vi "TLB Native Dynamic Events ver 0.17h.vi"() -> ()   [LabVIEW 2018]
uses:
  Labview Training Phase 2/Enum Controls/States for Action Engine.ctl
  TLB Type Definitions/State Type Definitions, for 0.26g versions and later 2.ctl
  TLB Type Definitions/Intruction Type Definitions.ctl
  TLB Type Definitions/Encoder cluster.ctl
  TLB Type Definitions/PING CLUSTER.ctl
  <vilib>/Studica/Studica Toolkit/NavX/NavX.lvlib
  <vilib>/Studica/Studica Toolkit/Background/DIO Channel.ctl
  Underlying VI's/NavX VI/navX type def.ctl
  <vilib>/Studica/Studica Toolkit/Background/I2C Channel.ctl
  TLB Type Definitions/Vision cluster.ctl
  <vilib>/NI_Real-Time Target Support.lvlib
  TLB Type Definitions/Stepper cluster.ctl
  Experimental VI's/Archived VI's/MOTOR CONTROL NO PID Type Def.ctl
  Underlying VI's/I2C Master VI/I2C MASTER Type Def.ctl
  Underlying VI's/I2C Master VI/I2C_MASTER_WRITE_NEW Type Def.ctl
  <vilib>/userdefined/High Color/IMAQdx.ctl
  Underlying VI's/I2C Master VI/Arduino_Interfacing.ctl
  TLB Type Definitions/Yaw Cluster.ctl
  TLB Type Definitions/Time cluster.ctl
  TLB Type Definitions/Y Stepper cluster.ctl
  Underlying VI's/Modified webcam FGV/Webcam AE.ctl
  Underlying VI's/Elasped Timer/Elapsed timer control.ctl
  Underlying VI's/Motor Control VI with PID/MOTOR CONTROL WITH PID AE DATA MODE TYPE DEF.ctl
  Underlying VI's/Motor Control VI with PID/MOTOR CONTROL WITH PID AE DIRECTION TYPE DEF.ctl
  TLB Type Definitions/IR Sensor Type Def.ctl
  <vilib>/myRIO/Common/Instrument Driver Framework/myRIO v1.0/AI/typedefs/AI Channels Enum.ctl
  <vilib>/myRIO/Common/Instrument Driver Framework/myRIO v1.0/AI/typedefs/AI Channels List.ctl
  TLB Type Definitions/Motor Speed Cluster.ctl
  <vilib>/Utility/RT CPU Load.ctl
panel:
  out "x-y":dbl
  out "Left IR Sensor":dbl
  out "Obstacle detected":bool
  out "Speed & distance":T1
  out "Object Center Coordinates":cluster{"x":sgl, "y":sgl}
  out "Object detection cluster":T2
  out "Time up flag":bool
  out "Task selection":u8
  in  "Object recognition mode":enum16{"Ball", "Soap", "Gel", "Pipe", "None"}(ring)
  out "NavX Readings":T3
  out "Arduino Data":T4
  out "CPU loads":T5[](array[typedef]) {"ISR (%)" format="%#.2f"; "Idle (%)" format="%#.2f"; "Background (%)" format="%#.2f"; "Normal (%)" format="%#.2f"; "Above Normal (%)" format="%#.2f"; "High (%)" format="%#.2g"; "Timed Structures (%)" format="%#.2g"; "Time Critical (%)" format="%#.2g"; "Total (%)" format="%#.2g"}
  out "TASK ENABLE":bool
  out "Rising Edge":bool
  in  "Green LED":bool
  out "I2C Error":errorcluster
  out "State Logic":T6=enum."Startup"
  out "elements":T7[](array[typedef])
  in  "STOP TASK":bool
  in  "OK Button":bool
  in  "STOP":bool
  out "error out":errorcluster
  out "Action Queue Items":i32
  out "State Logic Queue Items":i32
  out "Action Queues items":string[](array[string])=["Hardware reset", "Software reset", ""]
  out "Action State":string
  # "System Health Status Update"
  # "VISION"
  # "TLB FRAMEWORK STATUS"
  # "Test Programme written by Calvin Loke    Dated: 28 Aug 2019\nTest Programme revised by Dr Alex See   Dated 30 Aug 2019\n\nRevision date: 20/03/2020\nProgramme version:   TLB Native Dynamic Events ver 0.14a"
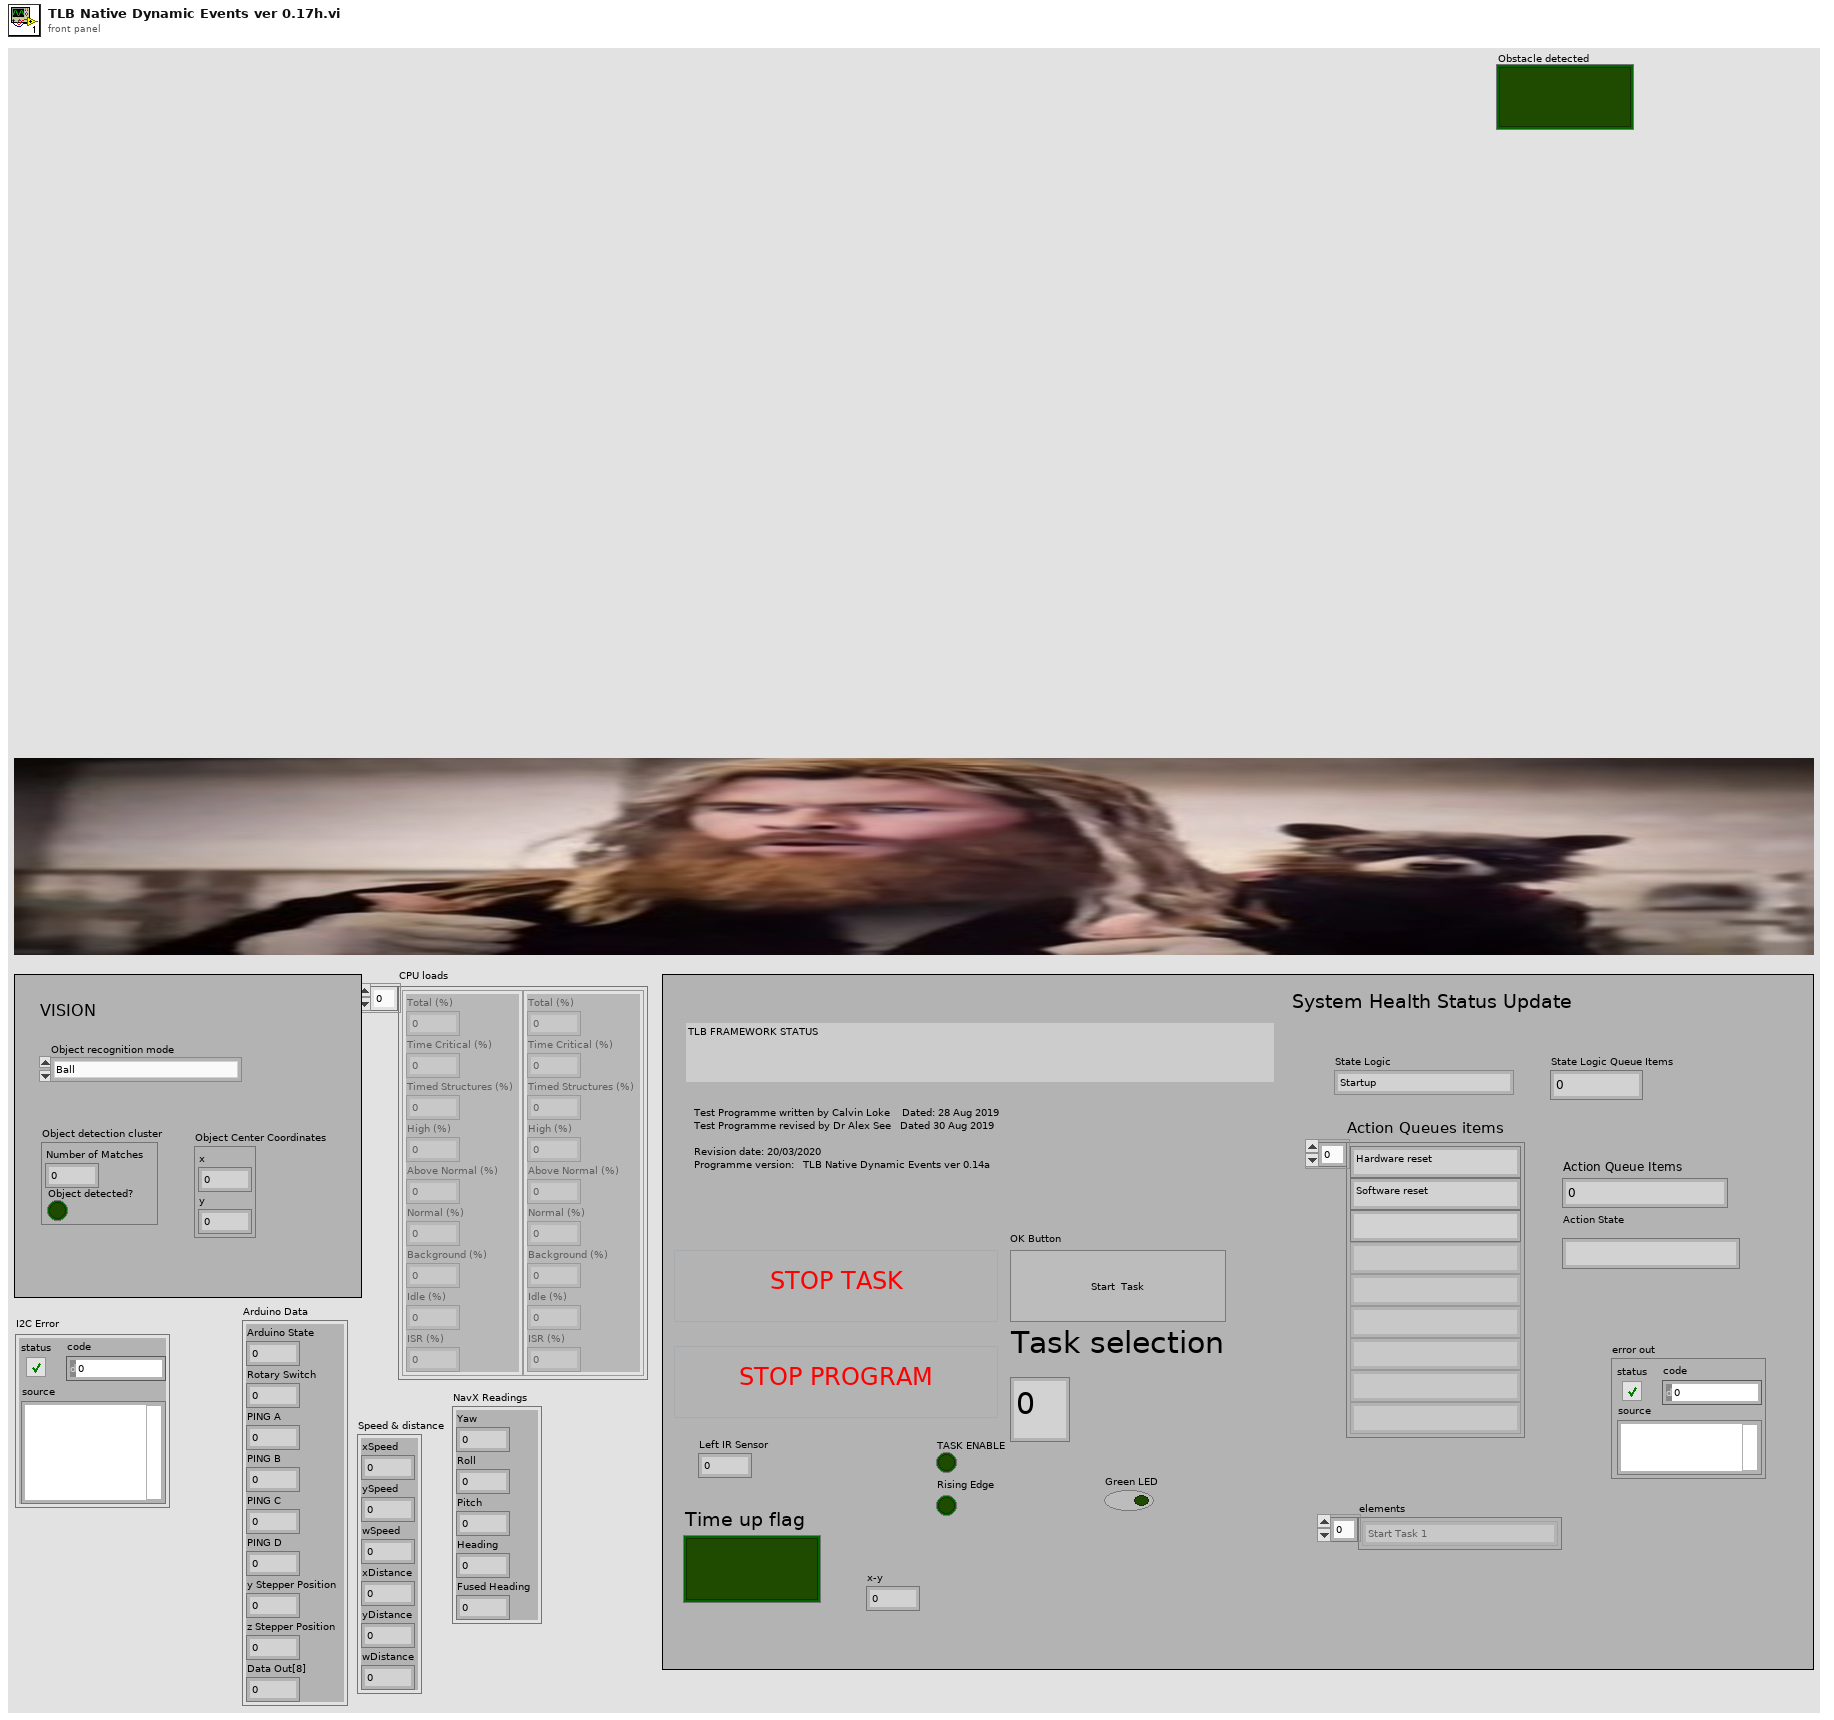
[diagram p1: front panel]
types:
  T1 = cluster{"xSpeed":dbl, "ySpeed":dbl, "wSpeed":dbl, "xDistance":dbl, "yDistance":dbl, "wDistance":dbl}
  T2 = cluster{"Number of Matches":i32, "Object detected?":bool}
  T3 = cluster{"Yaw":dbl, "Roll":dbl, "Pitch":dbl, "Heading":dbl, "Fused Heading":dbl}
  T4 = cluster{"Arduino State":u8, "Rotary Switch":u8, "PING A":u8, "PING B":u8, "PING C":u8, "PING D":u8, "y Stepper Position":u8, "z Stepper Position":u8, "Data Out[8]":u8}
  T5 = typedef "NI_Real-Time Target Support.lvlib/RT CPU Load.ctl" = cluster{"Total (%)":dbl, "Time Critical (%)":dbl, "Timed Structures (%)":dbl, "High (%)":dbl, "Above Normal (%)":dbl, "Normal (%)":dbl, "Background (%)":dbl, "Idle (%)":dbl, "ISR (%)":dbl}
  T6 = typedef "State Type Definitions, for 0.26g versions and later 2.ctl" = enum16{"None", "Startup", "Move to Angle", "True Stop", "Idle", "Shutdown", "Task 1A", "Task 1B", "Task 2:Raise Arm", "Task 2:Sensor Mode", "Task 2:Reverse Mode", "Task 3", "Task 4_A", "Task 4_B", "Task 4_C", "Task 4_D", "Task 5A", "Task 5B", "Task 5C", "Task 5D", "Task 5E: POSITION ARM", "Task 5F: ARM GRAB HEIGHT", "Task 5G: CLOSE CLAW", "Task 5H: RAISE ARM", "Task 6_A", "Task 6_B", "Task 7", "Task 8A: RAISE ARM", "Task 8B: MOVE TO BOX", "Task 8C: CAM BURST", "Task 8D: PROCESS IMAGE", "Task 8E: ROBOT ADJUST", "Task 8F: CAM BURST 2", "Task 8G: PROCESS IMAGE 2", "Task 8H: ARM ADJUST", "Task 8I: ARM GRAB HEIGHT", "Task 8J: CLOSE CLAW", "Task 8K: RAISE MY SWORD", "Task 9A: Raise Arm", "Task 9B: Rotate to Angle", "Task 9C: Detect Box", "Task 9D: MOVE FORWARD", "Task 9E: MOVE LEFT", "Task 9F: SCAN BOX", "Task 9G: MOVE RIGHT", "Task 9H: SCAN BOX 2", "Task 9I: ROTATE 90 CW", "Task 9J: FORWARD", "Task 9K: RAM WALL", "Task 9L: MOVE RIGHT", "Task 9M: SCAN BOX 3", "Task 9M: MOVE RIGHT", "Task 9N: SCAN BOX 4", "PENIS", "PENIS 2", "PENIS 3", "Task 9R: PROCESS COLOUR", "Task A1: Task 9 Open cam", "Task A2: Task 9 Move Arm", "Task A3: Task 9 Set Timer", "Task A4: Tasl 9 Capture images", "Task A5: Task 9 Close camera", "Task A6: Process Colour", "Task A7: Dispose Camera Buffer"}
  T7 = typedef "Intruction Type Definitions.ctl" = enum16{"None", "Start Task 1", "Start Task 2", "Start Task 3", "Start Task 4", "Start Task 5", "Start Task 6", "Start Task 7", "Start Task 8 - BALL", "Start Task 8 - Gel", "Start Task 8 - Pipe", "Start Task 8 - Soap", "Start Task 9", "Start Task A", "Start Task B", "Exit"}
  T8 = typedef "Motor Speed Cluster.ctl" = cluster{"ySpeed":dbl, "xSpeed":dbl, "wSpeed":dbl}
  T9 = typedef "IR Sensor Type Def.ctl" = cluster{"Left IR Sensor":dbl, "Arm IR Sensor":dbl, "Bottom IR Sensor":dbl}
  T10 = typedef "Y Stepper cluster.ctl" = cluster{"yStepper desired":u8}
  T11 = typedef "Time cluster.ctl" = cluster{"Time up flag":bool, "SET TIME TO CHECK":dbl}
  T12 = typedef "Yaw Cluster.ctl" = cluster{"Yaw":dbl, "Compass":dbl}
  T13 = typedef "Stepper cluster.ctl" = cluster{"y Stepper Position":u8, "z Stepper Position":u8}
  T14 = typedef "DIO Channel.ctl" = enum16{"Not Connected", "A/DIO1", "A/DIO2", "A/DIO3", "A/DIO4", "A/DIO5", "A/DIO6", "A/DIO7", "A/DIO13", "B/DIO1", "B/DIO2", "B/DIO3", "B/DIO4", "B/DIO5", "B/DIO6", "B/DIO7", "B/DIO13", "C/DIO0", "C/DIO1", "C/DIO2", "C/DIO3", "C/DIO4", "C/DIO5", "C/DIO6", "C/DIO7"}
  T15 = typedef "Vision cluster.ctl" = cluster{"Recognized Object":bool, "Object X coordinate":dbl, "Object Y coordinate":dbl}
  T16 = typedef "PING CLUSTER.ctl" = cluster{"PING_A":u8, "PING_B":u8, "PING_C":u8, "PING_D":u8}
  T17 = typedef "Encoder cluster.ctl" = cluster{"xDistance":dbl, "yDistance":dbl, "wDistance":dbl}
  T18 = cluster{"DIO Channel":T14, "FPGA VI Reference Out":refnum<k20>}
  T19 = typedef "navX type def.ctl" = enum16{"Get i2C reference", "Read Values", "Zero Yaw"}
  T20 = typedef "Arduino_Interfacing.ctl" = enum16{"Initialize", "Write to Arduino", "Read From Arduino"}
  T21 = typedef "I2C Channel.ctl" = enum16{"Not Connected", "A", "B"}
  T22 = typedef "States for Action Engine.ctl" = enum16{"Initialize", "Write", "Read"}
  T23 = cluster{"I2C Ref Out":cluster{"I2C Channel":T21, "FPGA VI Reference Out":refnum<k20>}, "Connected":bool, "Slave Address (7-bit)":u8, "Registry":u8[]}
  T24 = typedef "Intruction Type Definitions.ctl" = enum16{"None", "Start Task 1", "Start Task 2", "Start Task 3", "Start Task 4", "Start Task 5", "Start Task 6", "Start Task 7", "Start Task 8", "Start Task 9", "Start Task A", "Start Task B", "Exit"}
  T25 = typedef "IMAQ Image.ctl" = refnum<image>
  T26 = typedef "State Type Definitions.ctl" = enum16{"None", "Startup", "Move to Angle", "True Stop", "Idle", "Shutdown", "Task 1", "Task 2:Raise Arm", "Task 2:Sensor Mode", "Task 2:Reverse Mode", "Task 3", "Task 4_A", "Task 4_B", "Task 4_C", "Task 4_D", "Task 5A: ARM CAM HEIGHT", "Task 5B: MOVE TO BOX", "Task 5C: CAM BURST", "Task 5D: PROCESS IMAGE", "Task 5E: POSITION ARM", "Task 5F: ARM GRAB HEIGHT", "Task 5G: CLOSE CLAW", "Task 5H: RAISE ARM", "Task 6_A", "Task 6_B", "Task 7", "Task 8A: RAISE ARM", "Task 8B: MOVE TO BOX", "Task 8C: CAM BURST", "Task 8D: PROCESS IMAGE", "Task 8E: ROBOT ADJUST", "Task 8F: CAM BURST 2", "Task 8G: PROCESS IMAGE 2", "Task 8H: ARM ADJUST", "Task 8I: ARM GRAB HEIGHT", "Task 8J: CLOSE CLAW", "Task 8K: RAISE MY SWORD", "Task 9A: Raise Arm", "Task 9B: Rotate to Angle", "Task 9C: Rotation alignmnet", "Task B"}
  T27 = typedef "MOTOR CONTROL WITH PID AE DIRECTION TYPE DEF.ctl" = enum16{"y-axis movement", "x-axis movement", "rotation", "stop", "reset encoders"}
  T28 = typedef "MOTOR CONTROL WITH PID AE DATA MODE TYPE DEF.ctl" = enum16{"Init AE", "Write to AE", "Read from AE"}
  T29 = typedef "Elapsed timer control.ctl" = enum16{"Start", "Pause", "Initialize"}
  T30 = typedef "I2C_MASTER_WRITE_NEW Type Def.ctl" = enum16{"Ultrasonic sensors", "Stepper origin", "zStepper 13.3k", "zStepper 13k", "zStepper 12k", "zStepper 11k", "zStepper 10k", "zStepper 9k", "zStepper 8k", "zStepper 7k", "zStepper 6k", "zStepper 5k", "zStepper 4k", "zStepper 3k", "zStepper 2k", "zStepper 1k", "zStepper 900", "zStepper 800", "zStepper 700", "zStepper 600", "zStepper 500", "zStepper 400", "zStepper 300", "zStepper 200", "zStepper 100", "zStepper 0", "yStepper control", "Open Claw", "Close Claw", "Soft Reset"}
  T31 = typedef "Webcam AE.ctl" = enum16{"Initialize Camera", "Open Camera", "Continuous Acquisition", "Close Camera", "Retrieve Image", "Dispose Camera Image Buffer"}
  T32 = typedef "IMAQdx.ctl" = refnum<k21>
  T33 = typedef "Webcam AE.ctl" = enum16{"Initialize Camera", "Open Camera", "Continuous Acquisition", "Close Camera", "Retrieve Image", "Dispose Image Buffers"}
  T34 = typedef "MOTOR CONTROL NO PID Type Def.ctl" = enum16{"Init", "Front Back", "Left Right", "Rotate", "Stop", "Latch"}
  T35 = typedef "AI Channels List.ctl" = T36[]
  T36 = typedef "AI Channels Enum.ctl" = enum16{"Not Connected", "AudioIn/Left", "AudioIn/Right", "C/AI0", "C/AI1", "A/AI0", "A/AI1", "A/AI2", "A/AI3", "A/AI4", "A/AI5", "A/AI6", "A/AI7", "B/AI0", "B/AI1", "B/AI2", "B/AI3", "B/AI4", "B/AI5", "B/AI6", "B/AI7", "AI/AI0", "AI/AI1", "AI/AI2", "AI/AI3", "A/AI0 (DIFF)", "A/AI1 (DIFF)", "A/AI2 (DIFF)", "A/AI3 (DIFF)", "B/AI0 (DIFF)", "B/AI1 (DIFF)", "B/AI2 (DIFF)", "B/AI3 (DIFF)"}
  T37 = typedef "I2C MASTER Type Def.ctl" = enum16{"Last State", "Mode 0", "Mode 1", "Mode 2", "Mode 3", "Mode 4", "Mode 5", "Mode 6", "Mode 7", "Mode 8", "Mode 9", "Mode 10"}
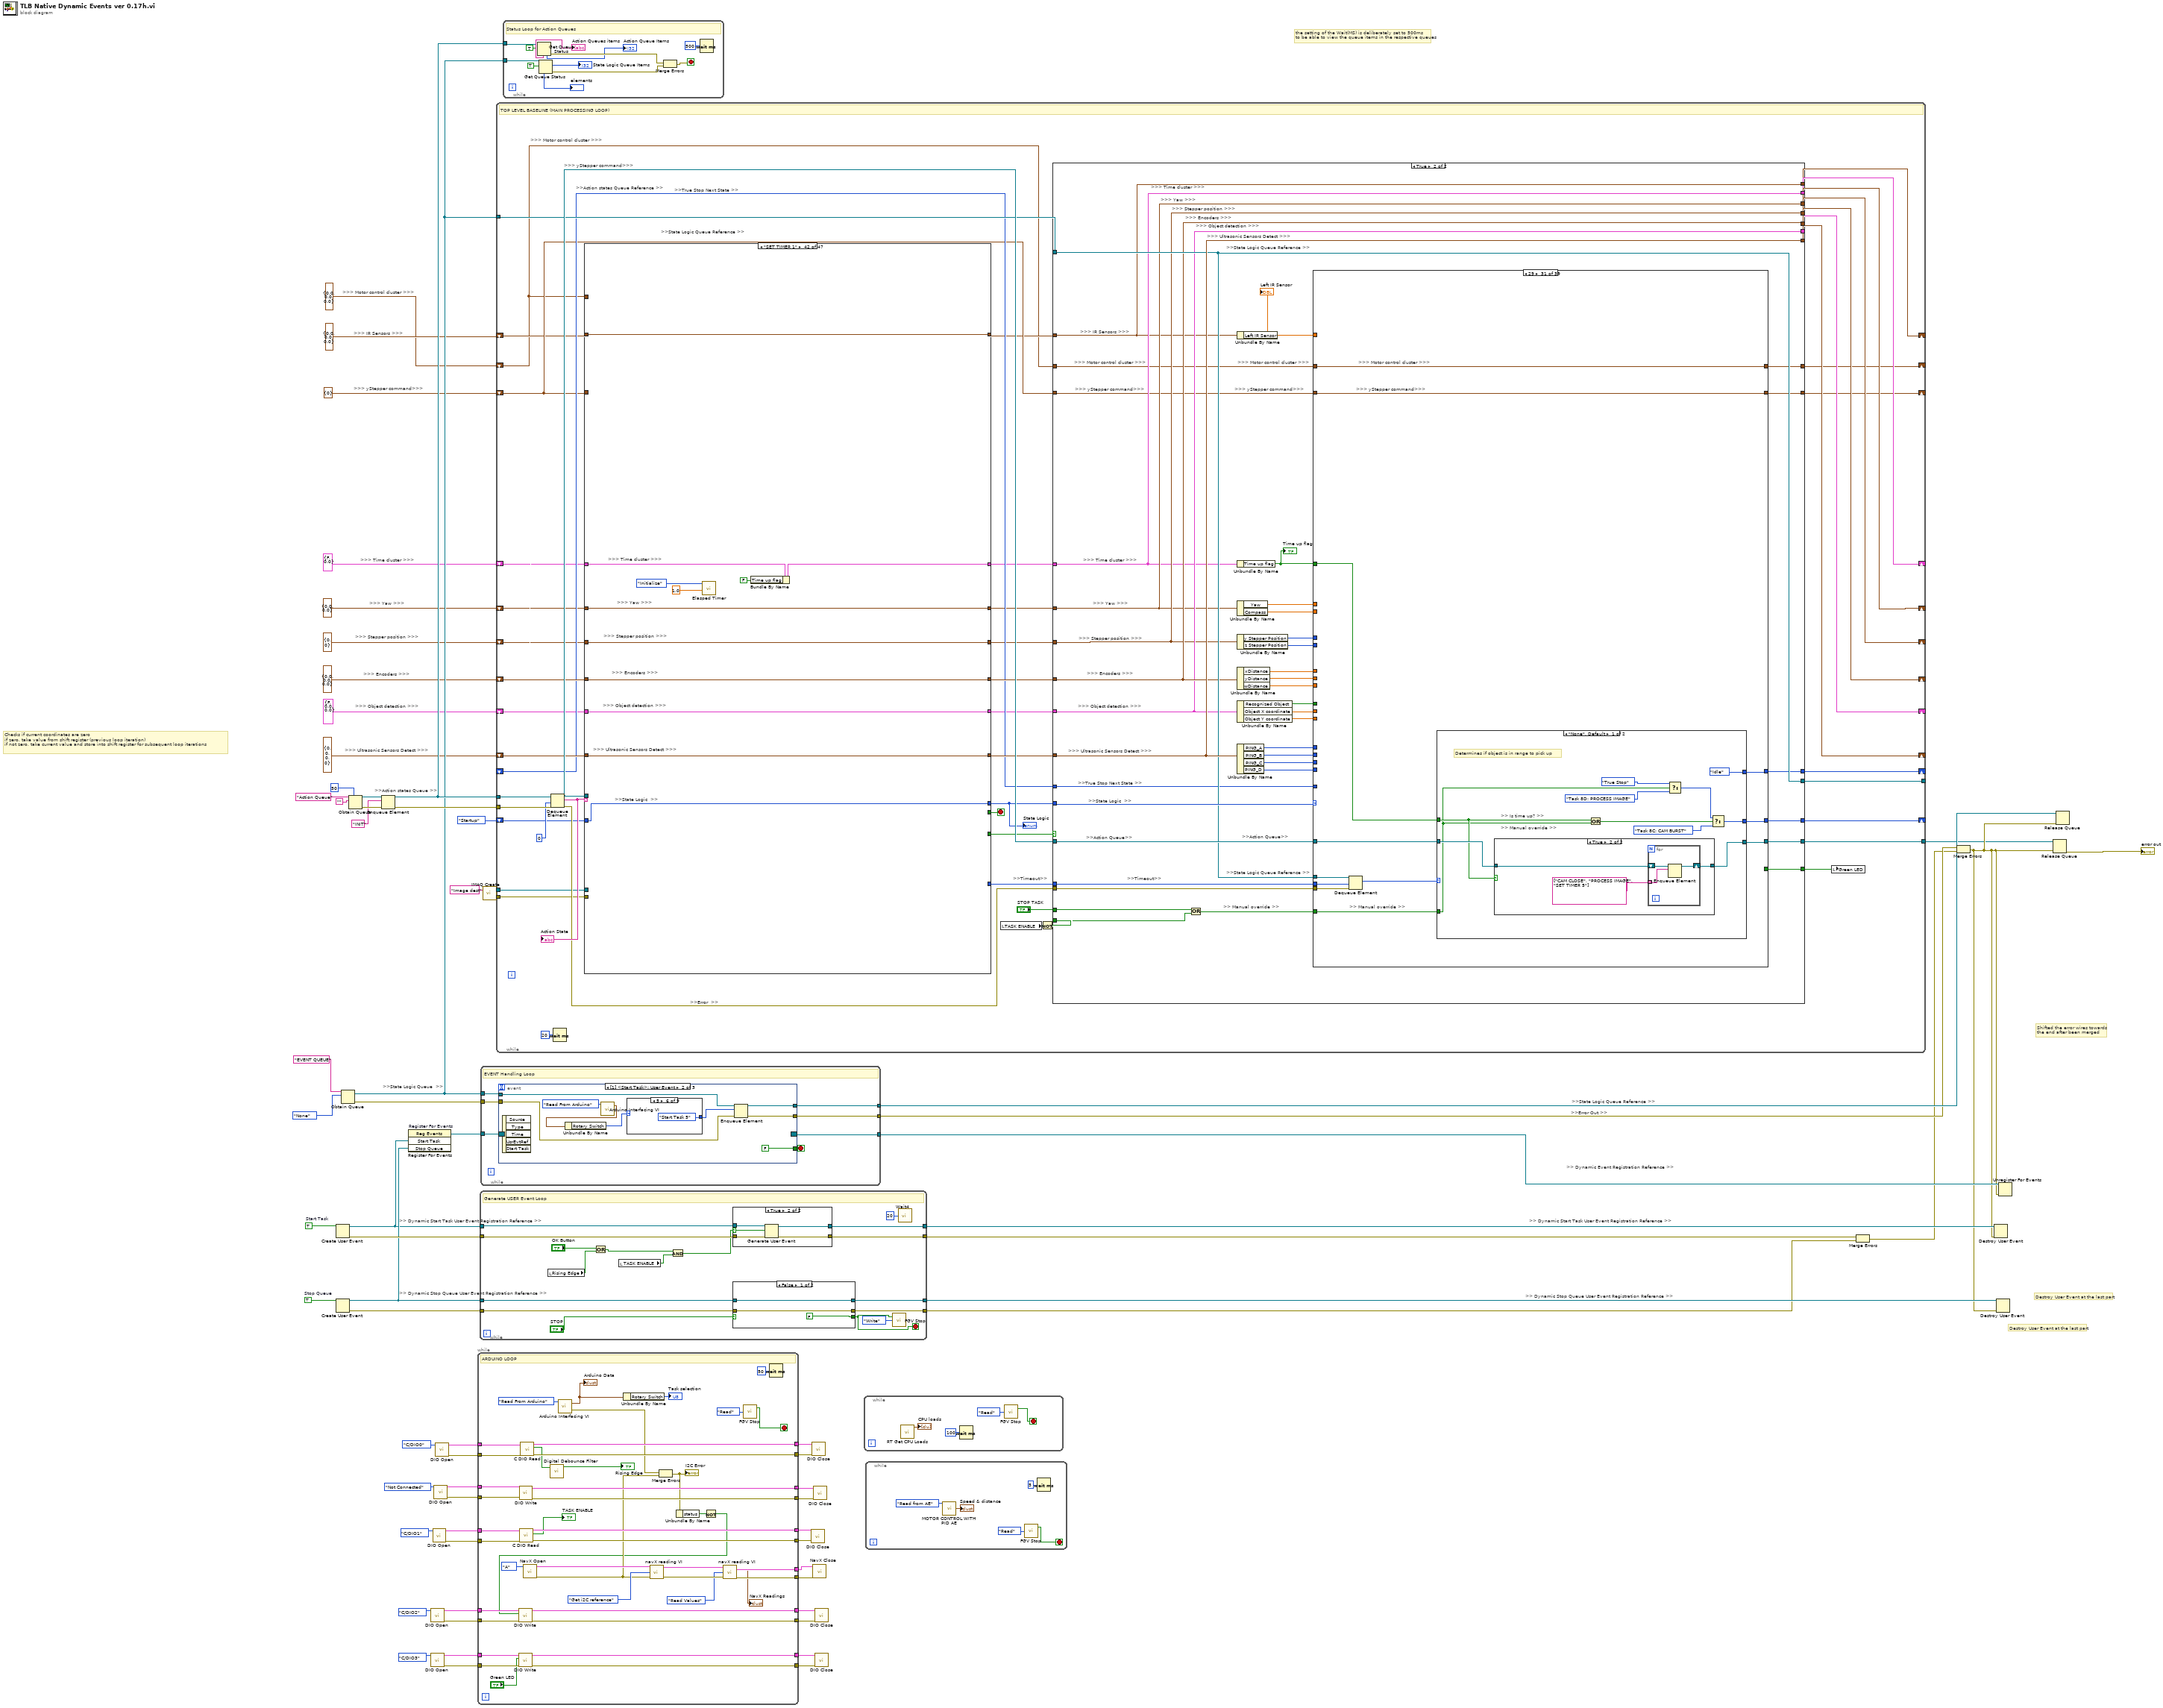
[diagram p0: block diagram]
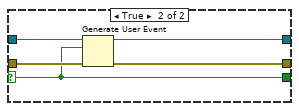
[diagram p2: hidden frame]
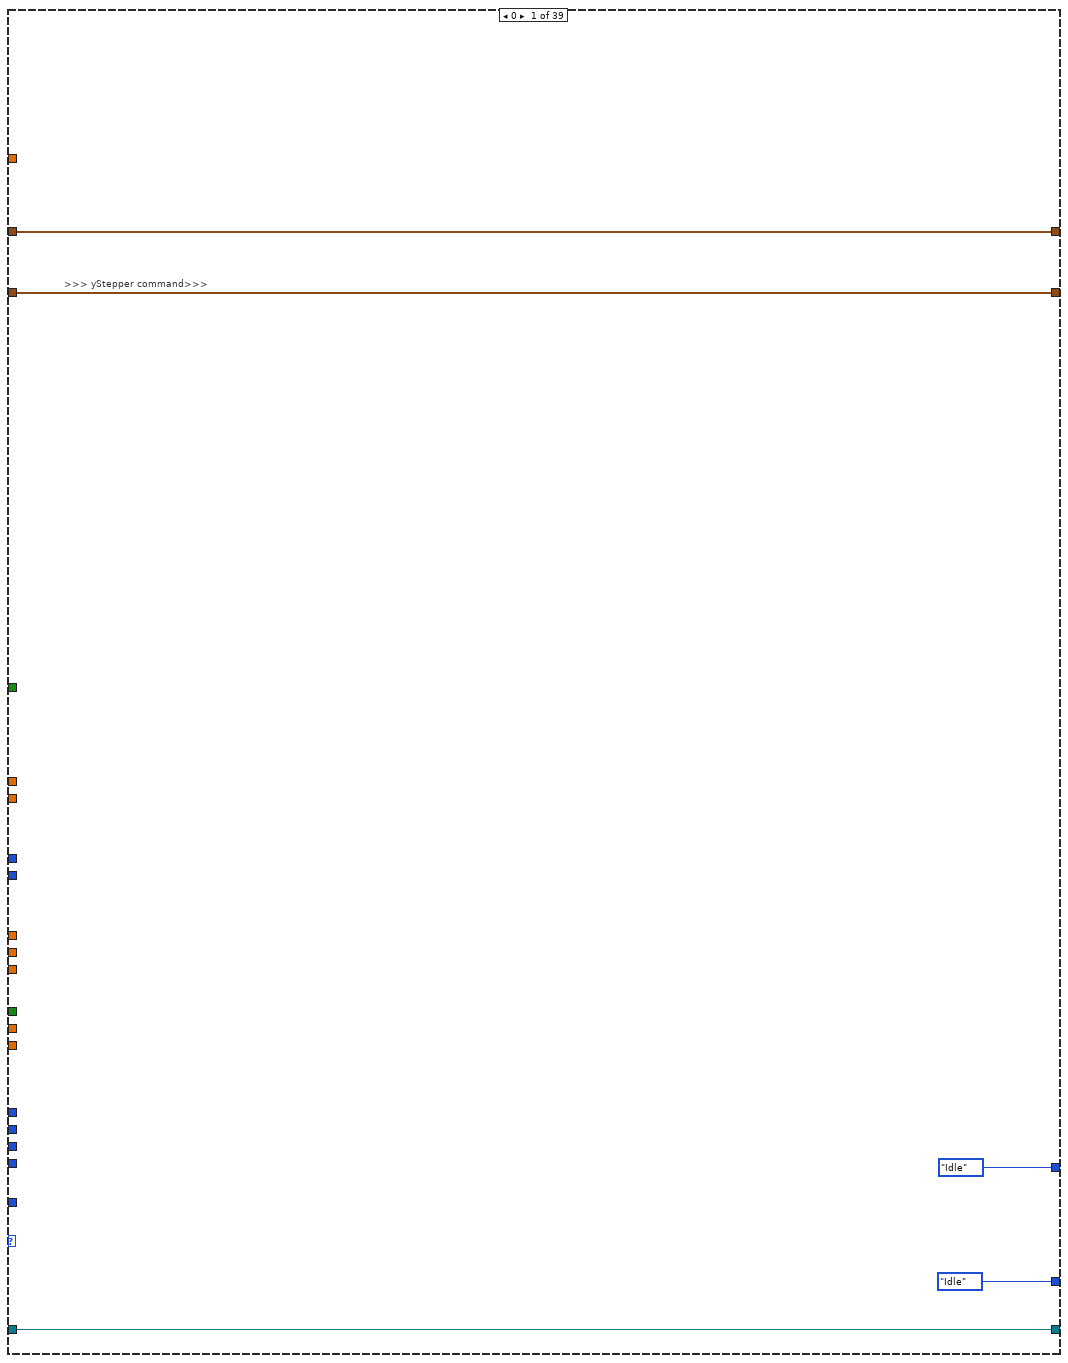
[diagram p5: hidden frame]
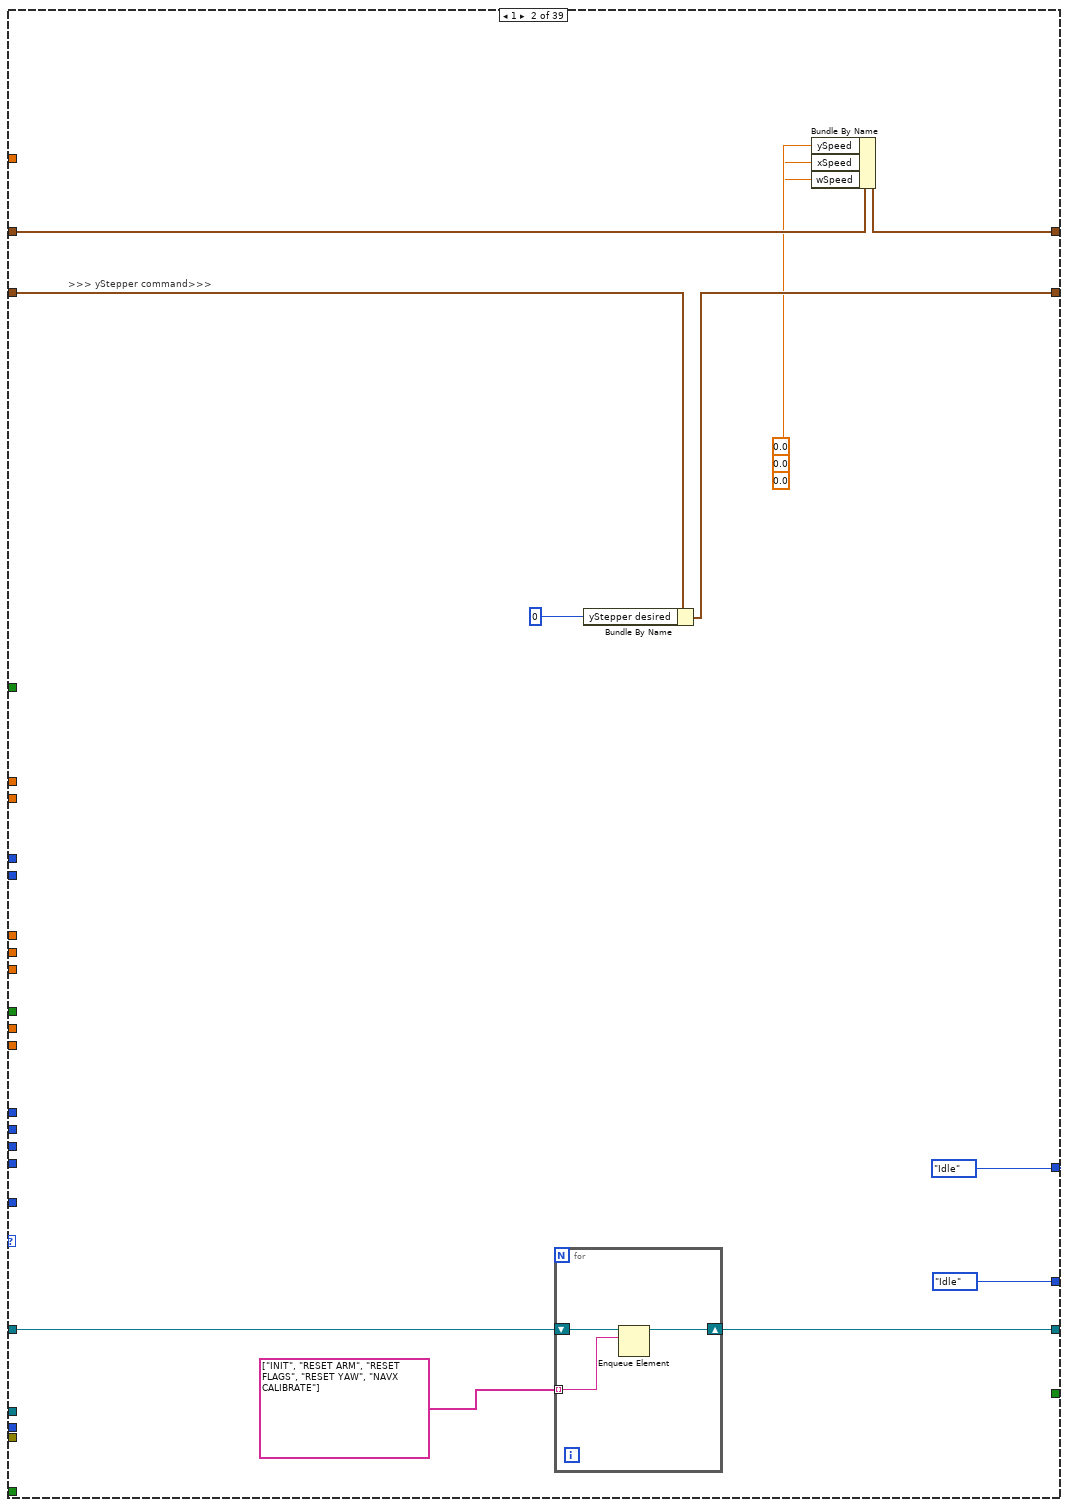
[diagram p6: hidden frame]
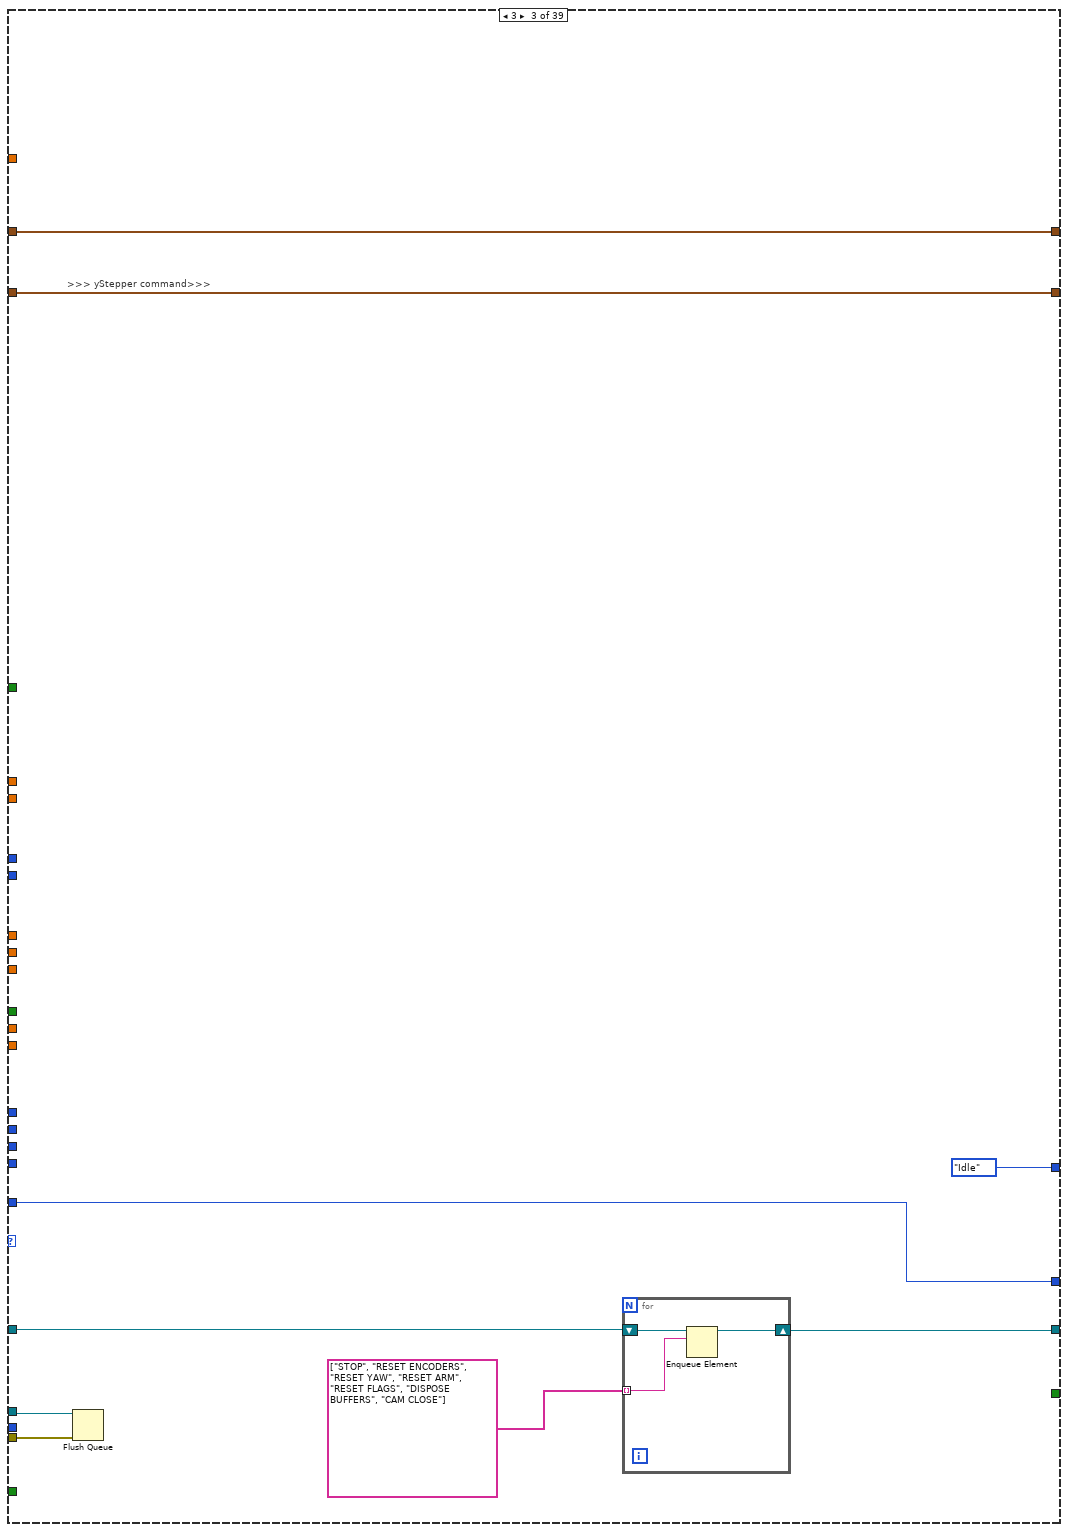
[diagram p7: hidden frame]
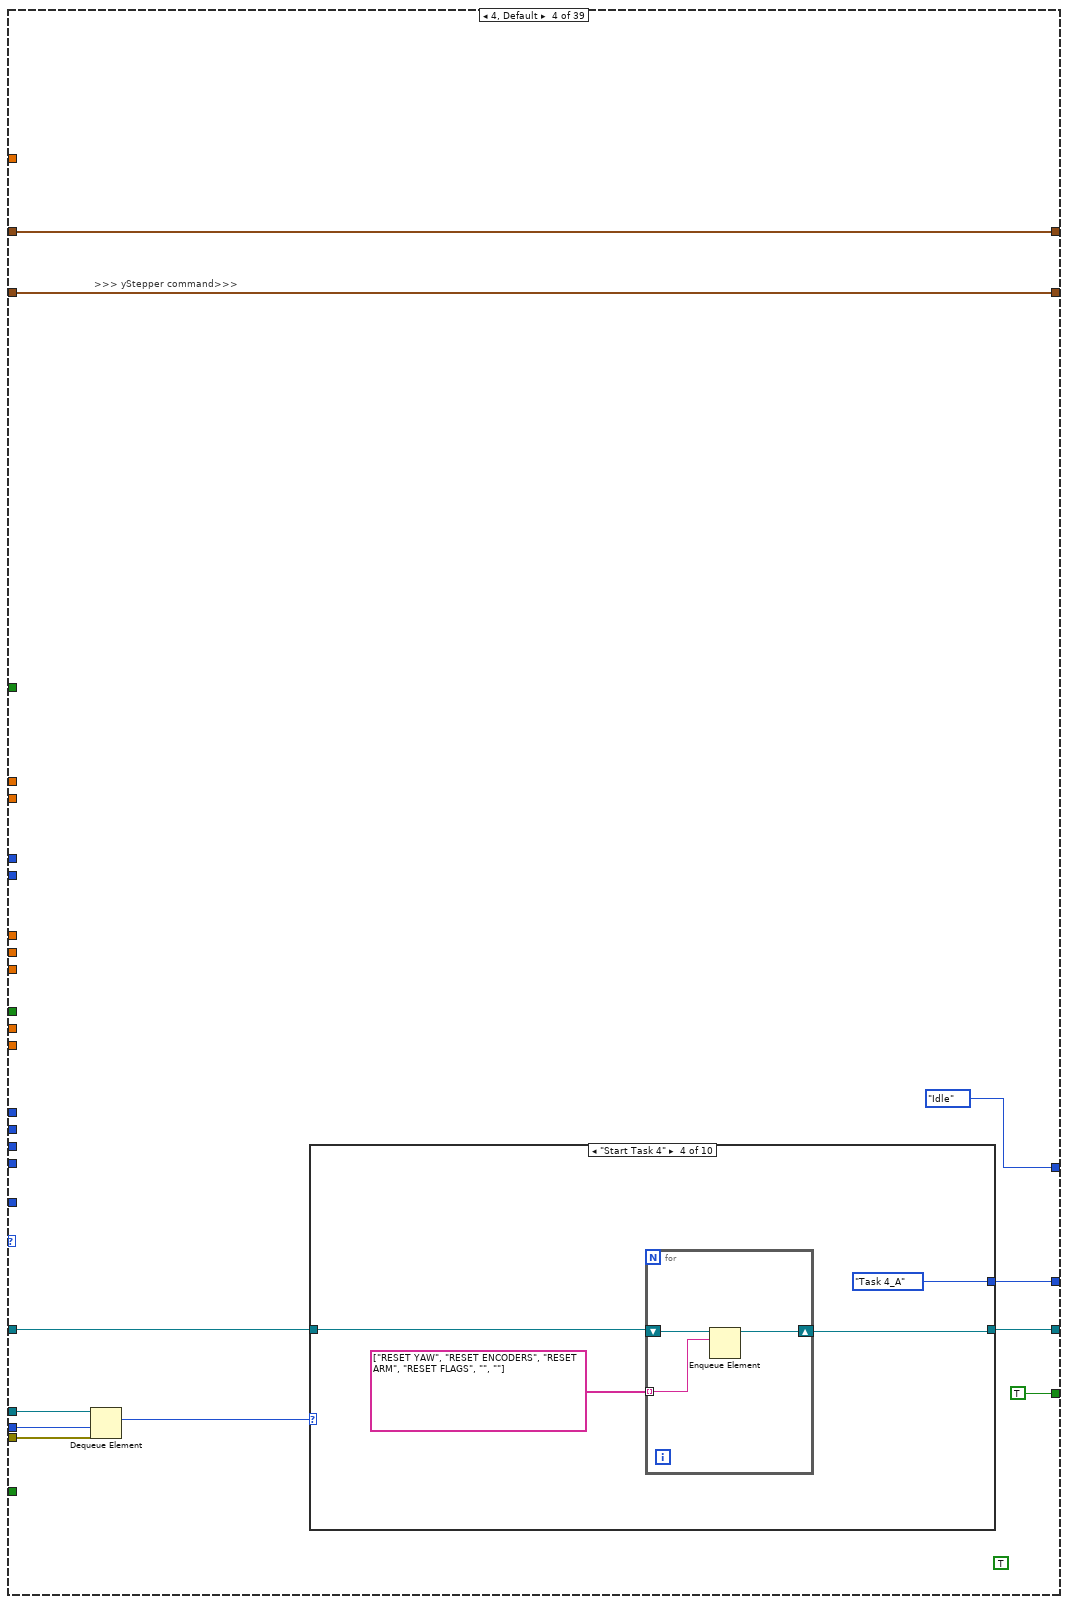
[diagram p8: hidden frame]
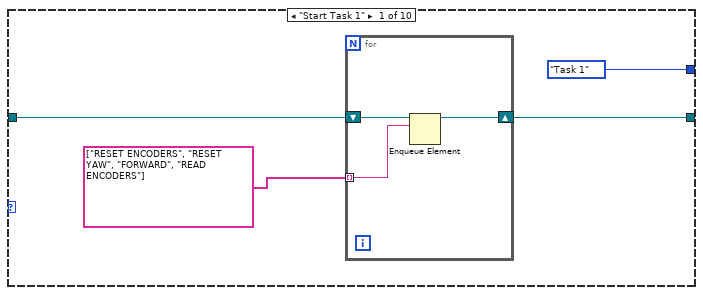
[diagram p9: hidden frame]
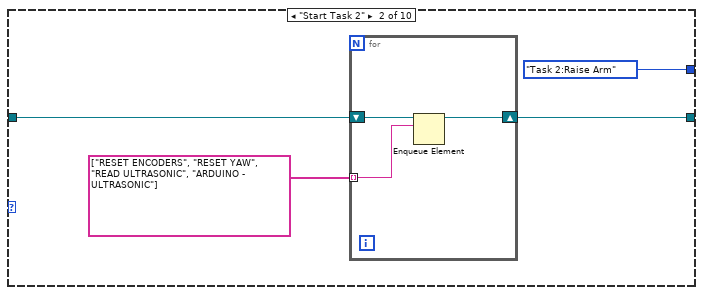
[diagram p10: hidden frame]
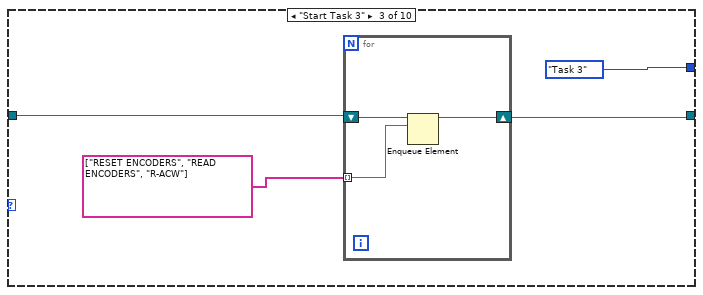
[diagram p11: hidden frame]
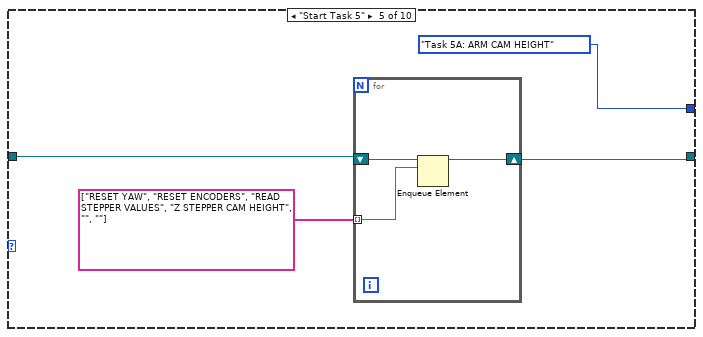
[diagram p12: hidden frame]
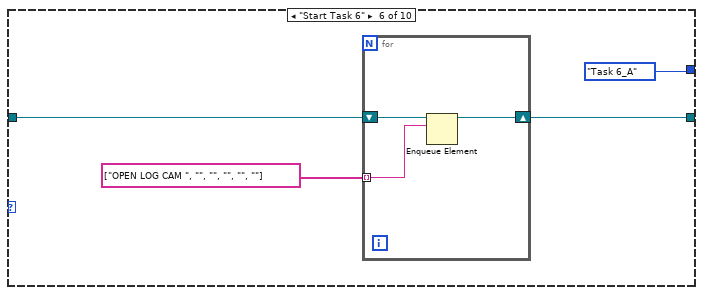
[diagram p13: hidden frame]
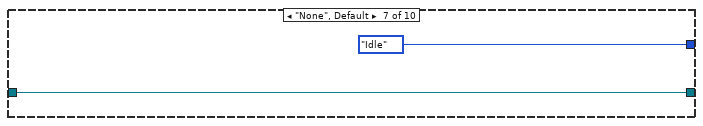
[diagram p14: hidden frame]
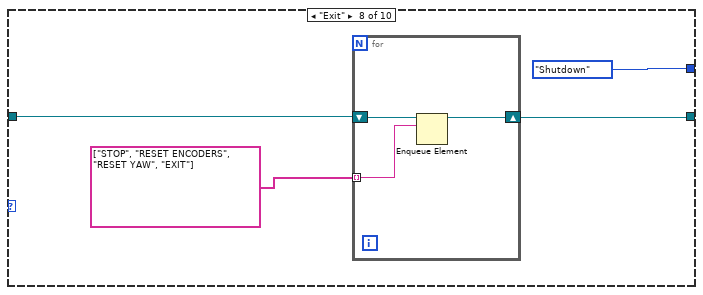
[diagram p15: hidden frame]
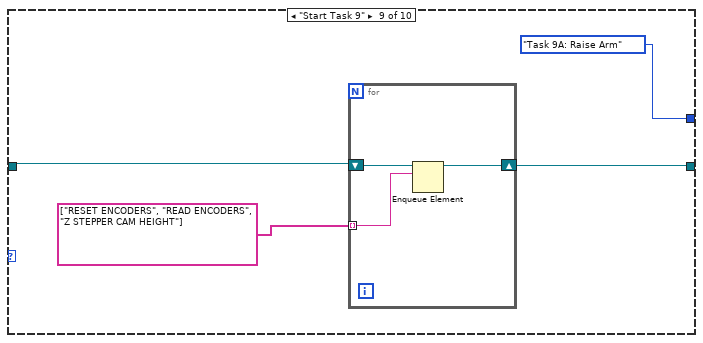
[diagram p16: hidden frame]
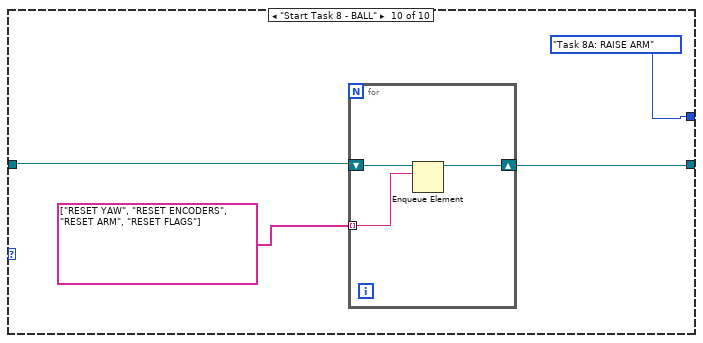
[diagram p17: hidden frame]
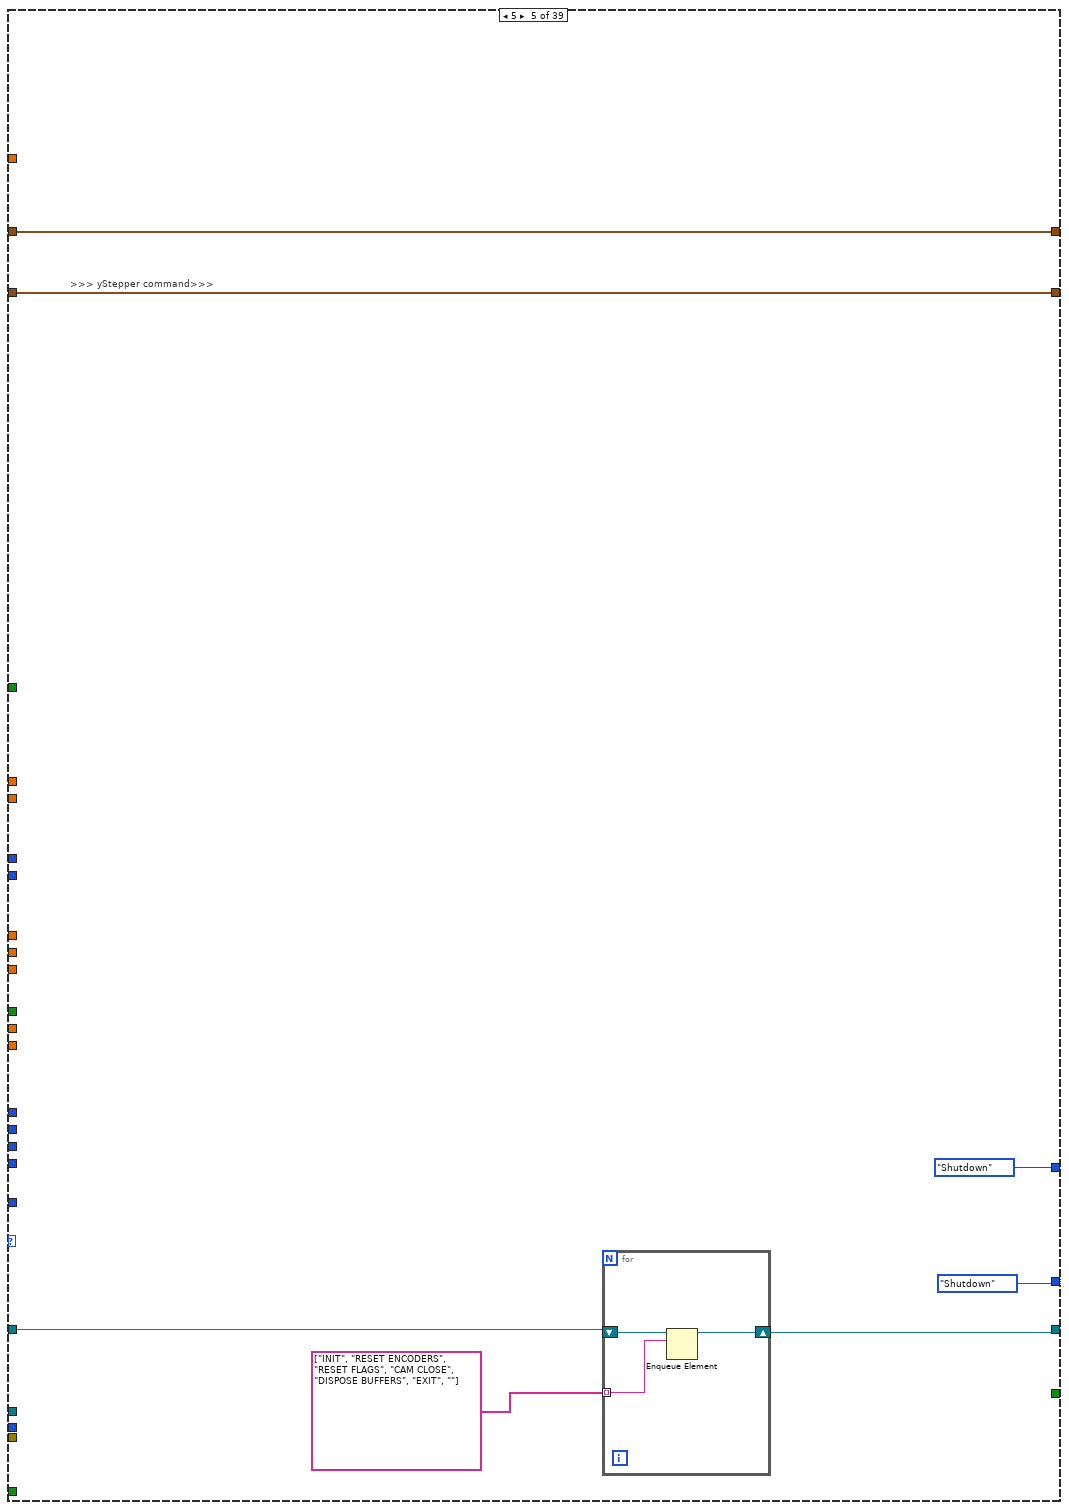
[diagram p18: hidden frame]
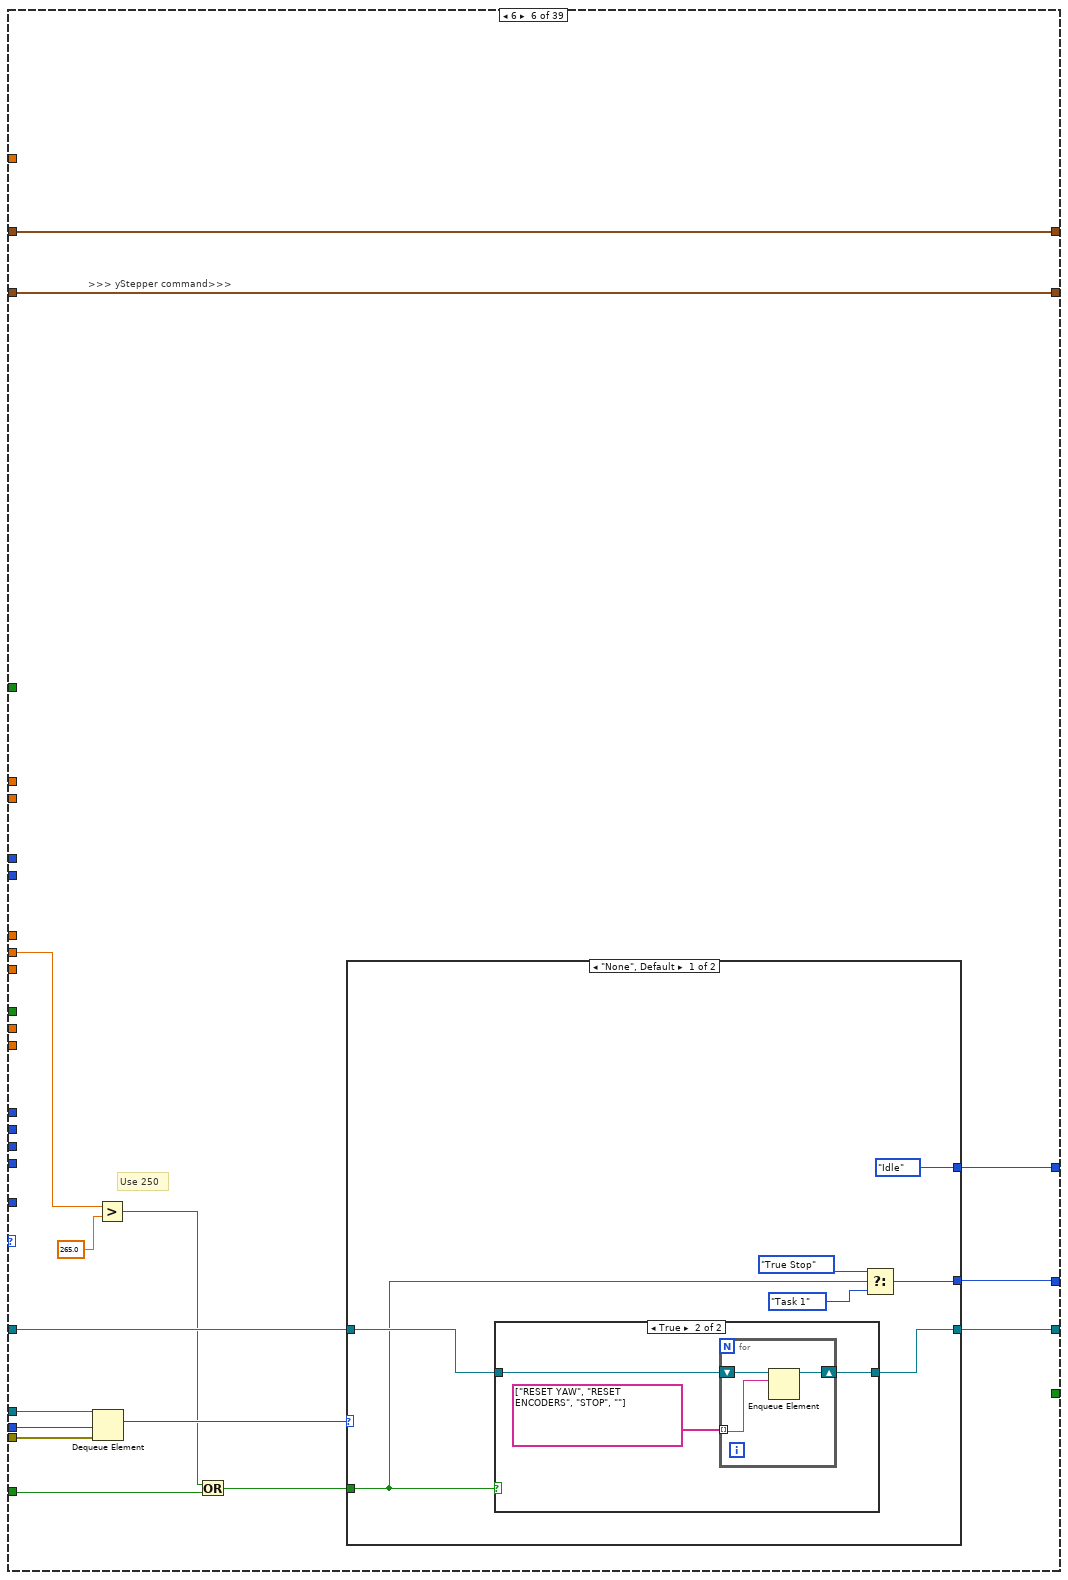
[diagram p19: hidden frame]
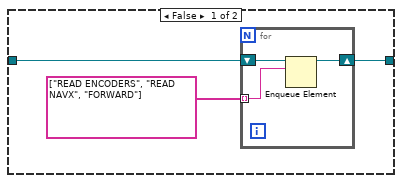
[diagram p20: hidden frame]
diagram:
  w70 = TRUE  # Stop Queue
  w69 = TRUE  # Start Task
  # ">>> Motor control cluster >>>"
  # ">>> IR Sensors >>>"
  # "Checks if current coordinates are zero\nif zero, take value from shift register (previous loop iteration)\nif not zero, take current value and store into shift register for subsequent loop iterations"
  # ">>> yStepper command>>>"
  # ">>> Time cluster >>>"
  # ">>> Yaw >>>"
  # ">>> Stepper position >>>"
  # ">>> Encoders >>>"
  # ">>> Object detection >>>"
  # ">>> Ultrasonic Sensors Detect >>>"
  # "the setting of the Wait(MS) is deliberately set to 500ms\nto be able to view the queue items in the respective queues"
  # ">>Error Out >>"
  # ">> Dynamic Stop Queue User Event Registration Reference >>"
  # ">> Dynamic Start Task User Event Registration Reference >>"
  # ">> Dynamic Stop Queue User Event Registration Reference >>"
  # ">> Dynamic Start Task User Event Registration Reference >>"
  # ">> Dynamic Event Registration Reference >>"
  # ">>Action states Queue >>"
  # ">>State Logic Queue  >>"
  # ">>State Logic Queue Reference >>"
  # "Destroy User Event at the last part"
  # "Destroy User Event at the last part"
  # "Shifted the error wires towards\nthe end after been merged"
  n1 = Create User Event(user event datatype=w69) -> (user event=w61:refnum<user-event>, error out=w66:errorcluster)  [unwired: 1 in]
  n2 = Create User Event(user event datatype=w70) -> (user event=w62:refnum<user-event>, error out=w65:errorcluster)  [unwired: 1 in]
  n3 = Obtain Queue(name (unnamed)="EVENT QUEUE", element data type=Intruction_Type_Definitions."None" ("Enum")) -> (queue out=w47:refnum<queue>, error out=w53:errorcluster)  [unwired: 3 in, 1 out]
  n4 = Obtain Queue(max queue size (-1, unlimited)=50, name (unnamed)="Action Queue", element data type="") -> (queue out=w56:refnum<queue>, error out=w52:errorcluster)  [unwired: 2 in, 1 out]
  n5 = Enqueue Element(queue=w56, element="INIT", error in (no error)=w52) -> (queue out=w48:refnum<queue>, error out=w51:errorcluster)  [unwired: 1 in, 1 out]
  n6 = register-events "Register For Events"(w61, w62) -> (reference out=w60:refnum<event-registration>)  [unwired: 2 in, 1 out]
  n7 = call <vilib>:"DIO Open.vi"("DIO Channel"=DIO_Channel."C/DIO2") -> ("error out"=w17:errorcluster, "DIO Info Out"=w18:T18)  [unwired: 9 in]
  n8 = call <vilib>:"DIO Open.vi"("DIO Channel"=DIO_Channel."C/DIO3") -> ("error out"=w12:errorcluster, "DIO Info Out"=w13:T18)  [unwired: 9 in]
  n9 = call <vilib>:"DIO Open.vi"("DIO Channel"=DIO_Channel."C/DIO1") -> ("error out"=w25:errorcluster, "DIO Info Out"=w26:T18)  [unwired: 9 in]
  n10 = call <vilib>:"DIO Open.vi"("DIO Channel"=DIO_Channel."Not Connected") -> ("error out"=w30:errorcluster, "DIO Info Out"=w32:T18)  [unwired: 9 in]
  n11 = call <vilib>:"DIO Open.vi"("DIO Channel"=DIO_Channel."C/DIO0") -> ("error out"=w35:errorcluster, "DIO Info Out"=w38:T18)  [unwired: 9 in]
  n12 = while {
    tunnel: w38 -> [w111]
    tunnel: [w110] -> w36
    tunnel: w35 -> [w109]
    tunnel: [w108] -> w34
    tunnel: w32 -> [w105]
    tunnel: [w104] -> w31
    tunnel: w30 -> [w103]
    tunnel: [w102] -> w29
    tunnel: [w101] -> w27
    tunnel: w26 -> [w100]
    tunnel: w25 -> [w99]
    tunnel: [w98] -> w24
    tunnel: w18 -> [w92]
    tunnel: w17 -> [w91]
    tunnel: [w90] -> w16
    tunnel: [w89] -> w15
    tunnel: w13 -> [w88]
    tunnel: w12 -> [w87]
    tunnel: [w86] -> w11
    tunnel: [w85] -> w10
    tunnel: [w79] -> w7
    tunnel: [w78] -> w8
    stop <- w113 stop-if-true
    # "ARDUINO LOOP"
    n13 = call <vilib>:"DIO Write.vi"("error in (no error)"=w87, "Input"="Green LED", "DIO Info In"=w88) -> ("error out"=w85:errorcluster, "DIO Info Out"=w86:T18)  [unwired: 7 in]
    n14 = call <vilib>:"DIO Write.vi"("error in (no error)"=w103, "DIO Info In"=w105) -> ("error out"=w102:errorcluster, "DIO Info Out"=w104:T18)  [unwired: 8 in]
    n15 = call <vilib>:"C DIO Read.vi"("error in (no error)"=w99, "DIO Info In in"=w100) -> ("error out"=w98:errorcluster, "IN"=→"TASK ENABLE":bool, "DIO Info In out"=w101:T18)  [unwired: 7 in]
    n16 = call <vilib>:"C DIO Read.vi"("error in (no error)"=w109, "DIO Info In in"=w111) -> ("error out"=w108:errorcluster, "IN"=w107:bool, "DIO Info In out"=w110:T18)  [unwired: 7 in]
    n17 = call <vilib>:"NavX Open.vi"("I2C Channel"=I2C_Channel."A") -> ("error out"=w94:errorcluster, "NavX Info"=w96:T23)  [unwired: 9 in]
    n18 = call "Digital Debounce Filter.vi"("Boolean input"=w107) -> ("Rising Edge"=→"Rising Edge":bool)  [unwired: 1 in, 2 out]
    n19 = call "Arduino Interfacing VI.vi"("AE Mode"=Arduino_Interfacing."Read From Arduino") -> ("error out"=w82:errorcluster, "Arduino Data"=w75:T4)  [unwired: 3 in]
    "Arduino Data" <- w75
    n20 = Unbundle By Name(w75) -> ("Rotary Switch"=→"Task selection":u8)
    n21 = call "navX reading VI.vi"("NavX Info In"=w96, "Mode"=navX_type_def."Get i2C reference", "error in (no error)"=w94) -> ("NavX Info Out"=w81:T23, "Error Out"=w80:errorcluster)  [unwired: 2 out]
    n22 = Merge Errors(w82, w94) -> (w73:errorcluster)
    "I2C Error" <- w73
    n23 = Unbundle By Name(w73) -> ("status"=w72:bool)
    n24 = Not(x=w72) -> (.not. x?=w71:bool)
    n25 = call <vilib>:"DIO Write.vi"("error in (no error)"=w91, "Input"=w71, "DIO Info In"=w92) -> ("error out"=w89:errorcluster, "DIO Info Out"=w90:T18)  [unwired: 7 in]
    n26 = call "navX reading VI.vi"("NavX Info In"=w81, "Mode"=navX_type_def."Read Values", "error in (no error)"=w80) -> ("NavX Info Out"=w79:T23, "NavX Readings"=→"NavX Readings":T3, "Error Out"=w78:errorcluster)  [unwired: 1 out]
    n27 = call "FGV Stop.vi"("Init/Read/Write State"=States_for_Action_Engine."Read") -> ("Output node"=w113:bool)  [unwired: 2 in, 1 out]
    n28 = Wait (ms)(milliseconds to wait=u32 50) -> ()  [unwired: 1 out]
  }
  n29 = while {
    tunnel: w61 -> [w131]
    tunnel: w62 -> [w130]
    tunnel: [w129] -> w68
    tunnel: [w128] -> w67
    tunnel: w66 -> [w127]
    tunnel: [w126] -> w64
    tunnel: w65 -> [w125]
    tunnel: [w124] -> w63
    stop <- w122 stop-if-true
    # "Generate USER Event Loop"
    n30 = local read "Rising Edge"() -> (w118:bool)
    n31 = Or(x="OK Button", y=w118) -> (x .or. y?=w117:bool)
    n32 = local read "TASK ENABLE"() -> (w116:bool)
    n33 = And(x=w117, y=w116) -> (x .and. y?=w115:bool)
    n34 = case shown="True" w115 {
      selector: w115 -> [_ w142]
      tunnel: w131 -> [w141 w146]
      tunnel: [w141 w145] -> w128
      tunnel: w127 -> [w140 w144]
      tunnel: [w140 w143] -> w126
      frame False {
      }
      frame True {
        n35 = Generate User Event(user event=w146, event data cluster=w142, error in=w144) -> (user event out=w145:refnum<user-event>, error out=w143:errorcluster)  [unwired: 1 in]
      }
    }
    n36 = case shown="False" "STOP" {
      selector: "STOP" -> [_ w135]
      tunnel: w130 -> [w134 w139]
      tunnel: [w134 w138] -> w129
      tunnel: w125 -> [w133 w137]
      tunnel: [w133 w136] -> w124
      tunnel: [FALSE w135] -> w122
      frame False {
      }
      frame True {
        n37 = Generate User Event(user event=w139, event data cluster=w135, error in=w137) -> (user event out=w138:refnum<user-event>, error out=w136:errorcluster)  [unwired: 1 in]
      }
    }
    n38 = call "FGV Stop.vi"("Init/Read/Write State"=States_for_Action_Engine."Write", "Input Node"=w122) -> ()  [unwired: 1 in, 2 out]
    n39 = call "Wait4"("Count(uSec)"=u32 20) -> ()  [unwired: 1 out]
  }
  n40 = while {
    tunnel: w60 -> [w153]
    tunnel: [w152] -> w59
    tunnel: w47 -> [w150]
    tunnel: [w149] -> w58
    tunnel: w53 -> [w148]
    tunnel: [w147] -> w50
    stop <- w151 stop-if-true
    # "EVENT Handling Loop"
    n41 = event shown="[1] <Start Task>: User Event" {
      selector: w153 -> [_ _ _]
      dyn-events: [_ _ _] -> w152
      timeout: _ -> [_ _ _]
      tunnel: [FALSE FALSE w183] -> w151
      tunnel: w150 -> [w158 w167 w181]
      tunnel: [w157 w166 w182] -> w149
      tunnel: w148 -> [w156 w165 w180]
      tunnel: [w155 w164 w179] -> w147
      event Timeout {
        n42 = event-data() -> ()  [unwired: 1 in, 3 out]
        n43 = Enqueue Element(queue=w158, element=Intruction_Type_Definitions."None" ("Enum"), error in (no error)=w156) -> (queue out=w157:refnum<queue>, error out=w155:errorcluster)  [unwired: 1 in, 1 out]
      }
      event User Event {
        n44 = event-data() -> ()  [unwired: 1 in, 5 out]
        n45 = call "Arduino Interfacing VI.vi"("AE Mode"=Arduino_Interfacing."Read From Arduino") -> ("Arduino Data"=w161:T4)  [unwired: 3 in, 1 out]
        n46 = Unbundle By Name(w161) -> ("Rotary Switch"=w160:u8)
        n47 = case shown="5" w160 {
          tunnel: [Intruction_Type_Definitions."None" ("Enum") Intruction_Type_Definitions."Start Task 1" ("Enum") Intruction_Type_Definitions."Start Task 2" ("Enum") Intruction_Type_Definitions."Start Task 3" ("Enum") Intruction_Type_Definitions."Start Task 4" ("Enum") Intruction_Type_Definitions."Start Task 5" ("Enum") Intruction_Type_Definitions."Start Task 6" ("Enum") Intruction_Type_Definitions."Start Task 8" ("Enum") Intruction_Type_Definitions."Start Task 9" ("Enum")] -> w163
          frame 0, Default {
          }
          frame 1 {
          }
          frame 2 {
          }
          frame 3 {
          }
          frame 4 {
          }
          frame 5 {
          }
          frame 6 {
          }
          frame 8 {
          }
          frame 9 {
          }
        }
        n48 = Enqueue Element(queue=w167, element=w163, error in (no error)=w165) -> (queue out=w166:refnum<queue>, error out=w164:errorcluster)  [unwired: 1 in, 1 out]
      }
      event User Event {
        n49 = event-data() -> ("Stop Queue"=w183:bool)  [unwired: 1 in, 4 out]
        n50 = Enqueue Element At Opposite End(queue=w181, element=Intruction_Type_Definitions."Exit" ("Enum"), error in (no error)=w180) -> (queue out=w182:refnum<queue>, error out=w179:errorcluster)  [unwired: 1 in, 1 out]
      }
    }
  }
  n51 = call "IMAQ Create"("Image Name"="Image dest") -> ("New Image"=w22:T25, "error out"=w21:errorcluster)  [unwired: 4 in]
  n52 = while {
    tunnel: w47 -> [w220]
    tunnel: w48 -> [w232]
    tunnel: w51 -> [w230]
    tunnel: [w229] -> _
    tunnel: [w228] -> w41
    shift-right: [w221] -> _
    shift-left: T16 {"PING_A"=0, "PING_B"=0, "PING_C"=0, "PING_D"=0} -> [w223]
    shift-right: [w214] -> _
    shift-left: State_Type_Definitions,_for_0.26g_versions_and_later_2."Startup" ("Enum") -> [w217]
    shift-right: [w210] -> _
    shift-left: T17 {"xDistance"=0.0, "yDistance"=0.0, "wDistance"=0.0} -> [w212]
    shift-right: [w207] -> _
    shift-left: _ -> [w206]
    tunnel: w22 -> [w205]
    tunnel: w21 -> [w204]
    shift-right: [w201] -> _
    shift-left: T15 {"Recognized Object"=FALSE, "Object X coordinate"=0.0, "Object Y coordinate"=0.0} -> [w203]
    shift-right: [w198] -> _
    shift-left: T13 {"y Stepper Position"=0, "z Stepper Position"=0} -> [w200]
    shift-right: [w195] -> _
    shift-left: T12 {"Yaw"=0.0, "Compass"=0.0} -> [w197]
    shift-right: [w192] -> _
    shift-left: T11 {"Time up flag"=FALSE, "SET TIME TO CHECK"=0.0} -> [w194]
    shift-right: [w190] -> _
    shift-left: T10 {"yStepper desired"=0} -> [w191]
    shift-right: [w186] -> _
    shift-left: T9 {"Left IR Sensor"=0.0, "Arm IR Sensor"=0.0, "Bottom IR Sensor"=0.0} -> [w188]
    shift-right: [w184] -> _
    shift-left: T8 {"ySpeed"=0.0, "xSpeed"=0.0, "wSpeed"=0.0} -> [w185]
    stop <- w219 stop-if-true
    # ">>> Motor control cluster >>>"
    # ">>> yStepper command>>>"
    # ">>True Stop Next State >>"
    # ">>Error  >>"
    # ">>Timeout>>"
    # ">>Action states Queue Reference >>"
    # ">>State Logic Queue Reference >>"
    # "TOP LEVEL BASELINE (MAIN PROCESSING LOOP)"
    n53 = Dequeue Element(queue=w232, timeout in ms (-1)=0, error in (no error)=w230) -> (queue out=w224:refnum<queue>, element=w231:string, error out=w225:errorcluster)  [unwired: 1 out]
    "Action State" <- w231
    n54 = Wait (ms)(milliseconds to wait=u32 20) -> ()  [unwired: 1 out]
    n55 = case shown="\"SET TIMER 1\"" w231 {
      tunnel: [_ _ _ _ _ _ _ _ _ _ _ _ _ _ _ _ _ _ _ 0 w2150 _ _ _ _ _ _ _ _ _ _ _ _ _ _ _ _ _ _ _ _ _ _ _ _ _ _] -> w227
      tunnel: w224 -> [_ _ _ _ _ _ _ _ _ _ _ _ _ _ _ _ _ _ _ _ _ _ _ _ _ _ _ _ _ _ _ _ _ _ _ _ _ _ _ _ _ _ _ _ _ _ _]
      tunnel: w223 -> [w1908 w1917 w1929 w1940 w1957 w1968 w1979 w1991 w2004 w2016 w2027 w2034 w2049 w2063 w2075 w2083 w2095 w2120 w2130 w2141 w2151 w2160 w2170 w2200 w2211 w2219 w2228 w2241 w2254 w2264 w2273 w2290 w2299 w2310 w2320 w2330 w2340 w2347 w2359 w2375 w2381 w2393 w2405 w2417 w2429 w2441 w2452]
      tunnel: [w1908 w1917 w1929 w1940 w1957 w1968 w1979 w1991 w2004 w2016 w2027 w2034 w2049 w2064 w2075 w2083 w2095 w2121 w2130 w2141 w2151 w2160 w2170 w2199 w2211 w2219 w2228 w2241 w2254 w2264 w2273 w2290 w2299 w2310 w2320 w2330 w2340 w2347 w2359 w2375 w2381 w2393 w2405 w2417 w2429 w2441 w2452] -> w222
      tunnel: [TRUE TRUE _ _ _ _ _ _ _ _ _ _ _ _ _ _ _ _ _ _ _ _ _ _ _ _ _ _ _ _ _ _ _ _ _ _ _ _ _ _ _ _ _ _ _ _ _] -> w219
      tunnel: w217 -> [w1906 w1915 w1928 w1939 w1956 w1967 w1978 w1990 w2003 w2015 w2026 w2033 w2048 w2062 w2074 w2081 w2094 w2119 w2129 w2138 w2148 w2159 w2169 w2198 w2210 w2218 w2227 w2240 w2253 w2263 w2272 w2289 w2298 w2309 w2319 w2329 w2339 w2346 w2358 w2374 w2380 w2392 w2404 w2416 w2428 w2440 w2451]
      tunnel: [_ _ _ _ _ _ _ _ _ _ _ _ _ _ _ _ _ _ _ _ TRUE _ _ _ _ _ _ _ _ _ _ _ _ _ _ _ _ _ _ _ _ _ _ _ _ _ _] -> w216
      tunnel: [w1906 w1915 w1928 w1939 w1956 w1967 w1978 w1990 w2003 w2015 w2026 w2033 w2048 w2062 w2074 w2081 w2094 w2119 w2129 w2138 w2148 w2159 w2169 w2198 w2210 w2218 w2227 w2240 w2253 w2263 w2272 w2289 w2298 w2309 w2319 w2329 w2339 w2346 w2358 w2374 w2380 w2392 w2404 w2416 w2428 w2440 w2451] -> w215
      tunnel: w212 -> [w1905 w1914 w1927 w1942 w1955 w1966 w1977 w1989 w2002 w2014 w2025 w2035 w2047 w2061 w2076 w2085 w2096 w2118 w2131 w2137 w2147 w2161 w2171 w2188 w2209 w2221 w2229 w2242 w2255 w2265 w2274 w2291 w2301 w2312 w2322 w2332 w2342 w2349 w2361 w2377 w2383 w2395 w2407 w2419 w2431 w2443 w2454]
      tunnel: [w1905 w1914 w1927 w1942 w1955 w1966 w1977 w1989 w2002 w2014 w2025 w2035 w2046 w2061 w2076 w2085 w2096 w2117 w2131 w2137 w2147 w2161 w2171 w2187 w2209 w2221 w2229 w2242 w2255 w2265 w2274 w2291 w2301 w2312 w2322 w2332 w2342 w2349 w2361 w2377 w2383 w2395 w2407 w2419 w2431 w2443 w2454] -> w211
      tunnel: w205 -> [w1900 _ _ _ _ _ _ _ _ _ _ _ _ _ _ _ _ _ _ _ _ _ _ _ _ _ _ _ _ _ _ w2285 _ _ _ _ _ _ _ _ _ _ _ _ _ _ _]
      tunnel: w204 -> [_ _ _ _ _ _ _ _ _ _ _ _ _ _ _ _ _ _ _ _ _ _ _ _ _ _ _ _ _ w2257 _ w2287 w2297 _ _ _ _ _ _ _ _ _ _ _ _ _ _]
      tunnel: w203 -> [w1904 w1913 w1926 w1941 w1954 w1965 w1976 w1988 w2001 w2013 w2023 w2032 w2045 w2060 w2069 w2084 w2093 w2109 w2128 w2136 w2146 w2158 w2168 w2193 w2207 w2220 w2226 w2239 w2252 w2259 w2271 w2282 w2300 w2311 w2321 w2331 w2341 w2348 w2360 w2376 w2382 w2394 w2406 w2418 w2430 w2442 w2453]
      tunnel: [w1904 w1913 w1926 w1941 w1954 w1965 w1976 w1988 w2001 w2013 w2023 w2032 w2045 w2060 w2069 w2084 w2093 w2108 w2128 w2136 w2146 w2158 w2168 w2192 w2207 w2220 w2226 w2239 w2252 w2259 w2271 w2281 w2300 w2311 w2321 w2331 w2341 w2348 w2360 w2376 w2382 w2394 w2406 w2418 w2430 w2442 w2453] -> w202
      tunnel: w200 -> [w1903 w1912 w1925 w1943 w1953 w1964 w1975 w1987 w2000 w2012 w2022 w2031 w2044 w2059 w2077 w2086 w2092 w2114 w2127 w2135 w2145 w2157 w2167 w2183 w2206 w2217 w2225 w2238 w2251 w2262 w2270 w2292 w2302 w2308 w2318 w2328 w2338 w2350 w2362 w2373 w2384 w2396 w2408 w2420 w2432 w2444 w2455]
      tunnel: [w1903 w1912 w1925 w1943 w1953 w1964 w1975 w1987 w2000 w2012 w2022 w2031 w2044 w2059 w2077 w2086 w2092 w2113 w2127 w2135 w2145 w2157 w2167 w2182 w2206 w2217 w2225 w2238 w2251 w2262 w2270 w2292 w2302 w2308 w2318 w2328 w2338 w2350 w2362 w2372 w2384 w2396 w2408 w2420 w2432 w2444 w2455] -> w199
      tunnel: w197 -> [w1902 w1911 w1923 w1944 w1951 w1962 w1974 w1985 w1998 w2010 w2021 w2030 w2043 w2052 w2072 w2087 w2091 w2104 w2126 w2134 w2144 w2156 w2166 w2179 w2205 w2214 w2224 w2237 w2250 w2261 w2269 w2293 w2303 w2307 w2315 w2325 w2335 w2351 w2363 w2367 w2385 w2397 w2409 w2421 w2433 w2445 w2456]
      tunnel: [w1902 w1911 w1923 w1944 w1951 w1962 w1974 w1985 w1998 w2010 w2021 w2030 w2043 w2052 w2071 w2087 w2091 w2103 w2126 w2134 w2144 w2156 w2166 w2178 w2205 w2214 w2224 w2237 w2250 w2261 w2269 w2293 w2303 w2307 w2315 w2325 w2335 w2351 w2363 w2367 w2385 w2397 w2409 w2421 w2433 w2445 w2456] -> w196
      tunnel: w194 -> [w1899 w1910 w1924 w1945 w1952 w1963 w1973 w1986 w1999 w2011 w2020 w2029 w2042 w2051 w2068 w2088 w2090 w2100 w2123 w2133 w2143 w2155 w2165 w2176 w2203 w2213 w2223 w2236 w2249 w2260 w2268 w2294 w2304 w2306 w2314 w2324 w2334 w2352 w2364 w2366 w2379 w2391 w2403 w2415 w2427 w2439 w2450]
      tunnel: [w1899 w1910 w1924 w1945 w1952 w1963 w1973 w1986 w1999 w2011 w2020 w2029 w2042 w2051 w2068 w2088 w2090 w2100 w2123 w2133 w2143 w2155 w2165 w2175 w2203 w2213 w2223 w2236 w2249 w2260 w2268 w2294 w2304 w2306 w2314 w2324 w2334 w2352 w2364 w2366 w2379 w2389 w2401 w2413 w2425 w2437 w2449] -> w193
      tunnel: w191 -> [_ _ _ _ _ _ _ _ _ _ _ _ _ _ _ _ _ _ _ _ _ _ _ _ _ _ _ _ _ _ _ _ _ _ _ _ _ _ w2355 _ _ _ _ _ _ _ _]
      tunnel: [w1898 w1909 w1918 w1935 w1946 w1958 w1969 w1980 w1994 w2005 w2017 w2028 w2036 w2050 w2065 w2079 w2089 w2097 w2122 w2132 w2142 w2154 w2162 w2172 w2202 w2212 w2222 w2230 w2243 w2256 w2266 w2275 w2295 w2305 w2313 w2323 w2333 w2343 w2353 w2365 w2378 w2386 w2398 w2410 w2422 w2434 w2446] -> w187
      tunnel: w188 -> [w1898 w1909 w1918 w1935 w1946 w1958 w1969 w1980 w1994 w2005 w2017 w2028 w2036 w2050 w2065 w2080 w2089 w2097 w2122 w2132 w2142 w2154 w2162 w2172 w2202 w2212 w2222 w2230 w2243 w2256 w2266 w2275 w2295 w2305 w2313 w2323 w2333 w2343 w2353 w2365 w2378 w2386 w2398 w2410 w2422 w2434 w2446]
      tunnel: w185 -> [_ _ _ _ _ _ _ _ w1993 _ _ _ _ _ _ _ _ _ _ _ _ _ _ _ _ _ _ _ _ _ _ _ _ _ _ _ _ _ _ _ _ _ _ _ _ _ _]
      frame "Exit" {
        # ">>State Logic  >>"
        # ">>> Time cluster >>>"
        # ">>> Yaw >>>"
        # ">>> Stepper position >>>"
        # ">>> Encoders >>>"
        # ">>> Object detection >>>"
        # ">>> Ultrasonic Sensors Detect >>>"
        n56 = call "Imaq Dispose"("All Images? (No)"=TRUE, "Image"=w1900) -> ()  [unwired: 4 in, 1 out]
      }
      frame "----Movement States----" {
        # ">>State Logic  >>"
        # ">>> Time cluster >>>"
        # ">>> Yaw >>>"
        # ">>> Stepper position >>>"
        # ">>> Encoders >>>"
        # ">>> Object detection >>>"
        # ">>> Ultrasonic Sensors Detect >>>"
      }
      frame "FORWARD" {
        # ">>State Logic  >>"
        # ">>> Time cluster >>>"
        # ">>> Yaw >>>"
        # ">>> Stepper position >>>"
        # ">>> Encoders >>>"
        # ">>> Object detection >>>"
        # ">>> Ultrasonic Sensors Detect >>>"
        n57 = Unbundle By Name(w1923) -> ("Yaw"=w1919:dbl)
        n58 = call "MOTOR CONTROL WITH PID AE.vi"("Yaw"=w1919, "Speed"=50.0, "Direction"=MOTOR_CONTROL_WITH_PID_AE_DIRECTION_TYPE_DEF."y-axis movement", "AE Mode"=MOTOR_CONTROL_WITH_PID_AE_DATA_MODE_TYPE_DEF."Write to AE") -> ()  [unwired: 1 out]
      }
      frame "FORWARD - IR ASSIST" {
        # ">>State Logic  >>"
        # ">>> Time cluster >>>"
        # ">>> Yaw >>>"
        # ">>> Stepper position >>>"
        # ">>> Encoders >>>"
        # ">>> Object detection >>>"
        # ">>> Ultrasonic Sensors Detect >>>"
        n59 = Unbundle By Name(w1935) -> ("Left IR Sensor"=w1934:dbl)
        n60 = Subtract(x=w1934, y=15.0) -> (x-y=w1932:dbl)
        n61 = Multiply(x=w1932, y=0.5) -> (x*y=w1930:dbl)
        n62 = call "MOTOR CONTROL WITH PID AE.vi"("Yaw"=w1930, "Speed"=30.0, "Direction"=MOTOR_CONTROL_WITH_PID_AE_DIRECTION_TYPE_DEF."y-axis movement", "AE Mode"=MOTOR_CONTROL_WITH_PID_AE_DATA_MODE_TYPE_DEF."Write to AE") -> ()  [unwired: 1 out]
      }
      frame "LEFT" {
        # ">>State Logic  >>"
        # ">>> Time cluster >>>"
        # ">>> Yaw >>>"
        # ">>> Stepper position >>>"
        # ">>> Encoders >>>"
        # ">>> Object detection >>>"
        # ">>> Ultrasonic Sensors Detect >>>"
        n63 = Unbundle By Name(w1951) -> ("Yaw"=w1948:dbl)
        n64 = call "MOTOR CONTROL WITH PID AE.vi"("Yaw"=w1948, "Speed"=-25.0, "Direction"=MOTOR_CONTROL_WITH_PID_AE_DIRECTION_TYPE_DEF."x-axis movement", "AE Mode"=MOTOR_CONTROL_WITH_PID_AE_DATA_MODE_TYPE_DEF."Write to AE") -> ()  [unwired: 1 out]
      }
      frame "R-ACW" {
        # ">>> IR Sensors >>>"
        # ">>> Time cluster >>>"
        # ">>> Yaw >>>"
        # ">>> Stepper position >>>"
        # ">>> Encoders >>>"
        # ">>> Object detection >>>"
        # ">>> Ultrasonic Sensors Detect >>>"
        n65 = call "MOTOR CONTROL WITH PID AE.vi"("Speed"=-10.0, "Direction"=MOTOR_CONTROL_WITH_PID_AE_DIRECTION_TYPE_DEF."rotation", "AE Mode"=MOTOR_CONTROL_WITH_PID_AE_DATA_MODE_TYPE_DEF."Write to AE") -> ()  [unwired: 1 in, 1 out]
      }
      frame "R-CW" {
        (unwired) -0.2 ("Speed")
        # ">>> Time cluster >>>"
        # ">>> Yaw >>>"
        # ">>> Stepper position >>>"
        # ">>> Encoders >>>"
        # ">>> Object detection >>>"
        # ">>> Ultrasonic Sensors Detect >>>"
        n66 = call "MOTOR CONTROL WITH PID AE.vi"("Speed"=10.0, "Direction"=MOTOR_CONTROL_WITH_PID_AE_DIRECTION_TYPE_DEF."rotation", "AE Mode"=MOTOR_CONTROL_WITH_PID_AE_DATA_MODE_TYPE_DEF."Write to AE") -> ()  [unwired: 1 in, 1 out]
      }
      frame "RIGHT" {
        # ">>> Time cluster >>>"
        # ">>> Yaw >>>"
        # ">>> Stepper position >>>"
        # ">>> Encoders >>>"
        # ">>> Object detection >>>"
        # ">>> Ultrasonic Sensors Detect >>>"
        n67 = Unbundle By Name(w1985) -> ("Yaw"=w1981:dbl)
        n68 = call "MOTOR CONTROL WITH PID AE.vi"("Yaw"=w1981, "Speed"=50.0, "Direction"=MOTOR_CONTROL_WITH_PID_AE_DIRECTION_TYPE_DEF."x-axis movement", "AE Mode"=MOTOR_CONTROL_WITH_PID_AE_DATA_MODE_TYPE_DEF."Write to AE") -> ()  [unwired: 1 out]
      }
      frame "X AXIS - SLOW" {
        # ">>> IR Sensors >>>"
        # ">>> Time cluster >>>"
        # ">>> Yaw >>>"
        # ">>> Stepper position >>>"
        # ">>> Encoders >>>"
        # ">>> Object detection >>>"
        # ">>> Ultrasonic Sensors Detect >>>"
        n69 = Unbundle By Name(w1993) -> ("xSpeed"=w1992:dbl)
        n70 = Unbundle By Name(w1998) -> ("Yaw"=w1995:dbl)
        n71 = call "MOTOR CONTROL WITH PID AE.vi"("Yaw"=w1995, "Speed"=w1992, "Direction"=MOTOR_CONTROL_WITH_PID_AE_DIRECTION_TYPE_DEF."x-axis movement", "AE Mode"=MOTOR_CONTROL_WITH_PID_AE_DATA_MODE_TYPE_DEF."Write to AE") -> ()  [unwired: 1 out]
      }
      frame "REVERSE" {
        # ">>> Time cluster >>>"
        # ">>> Yaw >>>"
        # ">>> Stepper position >>>"
        # ">>> Encoders >>>"
        # ">>> Object detection >>>"
        # ">>> Ultrasonic Sensors Detect >>>"
        n72 = Unbundle By Name(w2010) -> ("Yaw"=w2006:dbl)
        n73 = call "MOTOR CONTROL WITH PID AE.vi"("Yaw"=w2006, "Speed"=-50.0, "Direction"=MOTOR_CONTROL_WITH_PID_AE_DIRECTION_TYPE_DEF."y-axis movement", "AE Mode"=MOTOR_CONTROL_WITH_PID_AE_DATA_MODE_TYPE_DEF."Write to AE") -> ()  [unwired: 1 out]
      }
      frame "STOP" {
        n74 = Wait (ms)(milliseconds to wait=u32 100) -> ()  [unwired: 1 out]
        n75 = call "MOTOR CONTROL WITH PID AE.vi"("Direction"=MOTOR_CONTROL_WITH_PID_AE_DIRECTION_TYPE_DEF."stop", "AE Mode"=MOTOR_CONTROL_WITH_PID_AE_DATA_MODE_TYPE_DEF."Write to AE") -> ()  [unwired: 2 in, 1 out]
      }
      frame "----SENSOR READING---- " {
      }
      frame "READ ENCODERS" {
        # ">>> Time cluster >>>"
        # ">>> Yaw >>>"
        # ">>> Stepper position >>>"
        # ">>> Object detection >>>"
        # ">>> Current encoder distance >>>"
        # ">>> Ultrasonic Sensors Detect >>>"
        n76 = call "MOTOR CONTROL WITH PID AE.vi"("AE Mode"=MOTOR_CONTROL_WITH_PID_AE_DATA_MODE_TYPE_DEF."Read from AE") -> ("Speed & distance"=w2040:T1)  [unwired: 3 in]
        n77 = Unbundle By Name(w2040) -> ("xDistance"=w2039:dbl, "yDistance"=w2038:dbl, "wDistance"=w2037:dbl)
        n78 = Bundle By Name(cluster=w2047, "xDistance"=w2039, "yDistance"=w2038, "wDistance"=w2037) -> (w2046:T17)
      }
      frame "READ ULTRASONIC" {
        (unwired) navX_type_def."Read Values" ("Mode")
        (unwired) MOTOR_CONTROL_NO_PID_Type_Def."Latch" ("Direction")
        # ">>State Logic  >>"
        # ">>> Time cluster >>>"
        # ">>> Ultrasonic Sensors Detect >>>"
        # ">>> Object detection >>>"
        # ">>> Encoders >>>"
        # ">>> Stepper position >>>"
        # ">>> Yaw >>>"
        n79 = call "Arduino Interfacing VI.vi"("AE Mode"=Arduino_Interfacing."Read From Arduino") -> ("Arduino Data"=w2057:T4)  [unwired: 3 in, 1 out]
        n80 = Unbundle By Name(w2057) -> ("PING A"=w2056:u8, "PING B"=w2055:u8, "PING C"=w2054:u8, "PING D"=w2053:u8)
        n81 = Bundle By Name(cluster=w2063, "PING_A"=w2056, "PING_B"=w2055, "PING_C"=w2054, "PING_D"=w2053) -> (w2064:T16)
      }
      frame "READ NAVX" {
        # ">>> Time cluster >>>"
        # ">>> Yaw >>>"
        # ">>> Ultrasonic Sensors Detect >>>"
        # ">>> Object detection >>>"
        # ">>> Encoders >>>"
        # ">>> Stepper position >>>"
        n82 = call "navX reading VI.vi"("Mode"=navX_type_def."Read Values") -> ("NavX Readings"=w2067:T3)  [unwired: 2 in, 3 out]
        n83 = Unbundle By Name(w2067) -> ("Heading"=w2066:dbl)
        n84 = Unbundle By Name(w2067) -> ("Yaw"=w2070:dbl)
        n85 = Bundle By Name(cluster=w2072, "Yaw"=w2070, "Compass"=w2066) -> (w2071:T12)
      }
      frame "READ IR" {
        w2082 = T35 [enum."A/AI0"] items=["Not Connected", "AudioIn/Left", "AudioIn/Right", "C/AI0", "C/AI1", "A/AI0", "A/AI1", "A/AI2", "A/AI3", "A/AI4", "A/AI5", "A/AI6", "A/AI7", "B/AI0", "B/AI1", "B/AI2", "B/AI3", "B/AI4", "B/AI5", "B/AI6", "B/AI7", "AI/AI0", "AI/AI1", "AI/AI2", "AI/AI3", "A/AI0 (DIFF)", "A/AI1 (DIFF)", "A/AI2 (DIFF)", "A/AI3 (DIFF)", "B/AI0 (DIFF)", "B/AI1 (DIFF)", "B/AI2 (DIFF)", "B/AI3 (DIFF)"] ("AI Channel")
        # ">>State Logic  >>"
        # ">>> Time cluster >>>"
        # ">>> Ultrasonic Sensors Detect >>>"
        # ">>> Object detection >>>"
        # ">>> Encoders >>>"
        # ">>> Stepper position >>>"
        # ">>> Yaw >>>"
        n86 = call <vilib>:"Sharp IR.vi"("AI Channel"=w2082) -> ("Sharp IR Distance"=w2078:dbl)  [unwired: 8 in, 2 out]
        n87 = Bundle By Name(cluster=w2080, "Left IR Sensor"=w2078) -> (w2079:T9)
      }
      frame "----SYSTEM MODES----" {
        (unwired) I2C_MASTER_Type_Def."Last State" ("Arduino Mode")
        # ">>> Object detection >>>"
        # ">>> Yaw >>>"
        # ">>> Ultrasonic Sensors Detect >>>"
        # ">>> Encoders >>>"
        # ">>> Stepper position >>>"
      }
      frame "INIT" {
        w2115 = u8 0
        w2116 = 0.0
        # ">>> Time cluster >>>"
        # ">>> Object detection >>>"
        # ">>> Yaw >>>"
        # ">>> Ultrasonic Sensors Detect >>>"
        # ">>> Encoders >>>"
        # ">>> Stepper position >>>"
        # ">>State Logic  >>"
        n88 = call "Arduino Interfacing VI.vi"("AE Mode"=Arduino_Interfacing."Initialize") -> ()  [unwired: 3 in, 2 out]
        n89 = call "FGV Stop.vi"("Init/Read/Write State"=States_for_Action_Engine."Initialize") -> ()  [unwired: 2 in, 2 out]
        n90 = call "Elasped Timer.vi"("Action"=Elapsed_timer_control."Initialize") -> ()  [unwired: 7 in, 4 out]
        n91 = call "MOTOR CONTROL WITH PID AE.vi"("AE Mode"=MOTOR_CONTROL_WITH_PID_AE_DATA_MODE_TYPE_DEF."Init AE") -> ()  [unwired: 3 in, 1 out]
        n92 = Bundle By Name(cluster=w2109, "Recognized Object"=FALSE, "Object X coordinate"=0.0, "Object Y coordinate"=0.0) -> (w2108:T15)
        n93 = Bundle By Name(cluster=w2114, "y Stepper Position"=u8 0, "z Stepper Position"=u8 0) -> (w2113:T13)
        n94 = Bundle By Name(cluster=w2118, "xDistance"=w2116, "yDistance"=w2116, "wDistance"=w2116) -> (w2117:T17)
        n95 = Bundle By Name(cluster=w2120, "PING_A"=w2115, "PING_B"=w2115, "PING_C"=w2115, "PING_D"=w2115) -> (w2121:T16)
        n96 = Bundle By Name(cluster=w2104, "Yaw"=0.0) -> (w2103:T12)
      }
      frame "ARDUINO - ULTRASONIC" {
        # ">>> Object detection >>>"
        # ">>> Yaw >>>"
        # ">>> Ultrasonic Sensors Detect >>>"
        # ">>> Encoders >>>"
        # ">>> Stepper position >>>"
        # ">>State Logic  >>"
        n97 = call "Arduino Interfacing VI.vi"("Data to Write"=I2C_MASTER_WRITE_NEW_Type_Def."Ultrasonic sensors", "AE Mode"=Arduino_Interfacing."Write to Arduino") -> ()  [unwired: 2 in, 2 out]
      }
      frame "NAVX CALIBRATE" {
        # ">>> Object detection >>>"
        # ">>> Yaw >>>"
        # ">>> Ultrasonic Sensors Detect >>>"
        # ">>> Encoders >>>"
        # ">>> Stepper position >>>"
        # ">>State Logic  >>"
        # "Adds a 15 second delay to the startup process \nfor the NavX to calibrate"
        n98 = Wait (ms)(milliseconds to wait=u32 1000) -> ()  [unwired: 1 out]
      }
      frame "NO ACTION", Default {
        (unwired) u8 0 ("y Stepper value")
        (unwired) TRUE ("Latch")
        (unwired) navX_type_def."Read Values" ("Mode")
        (unwired) MOTOR_CONTROL_NO_PID_Type_Def."Latch" ("Direction")
        # ">>> Object detection >>>"
        # ">>> Yaw >>>"
        # ">>> Ultrasonic Sensors Detect >>>"
        # ">>> Encoders >>>"
        # ">>> Stepper position >>>"
        # ">>State Logic  >>"
        n99 = case shown="4" w2148 {
          tunnel: [0 100] -> w2150
          frame 1, Default {
          }
          frame 4 {
          }
        }
      }
      frame "----RESET CASES----" {
        (unwired) I2C_MASTER_Type_Def."Last State" ("Arduino Mode")
        # ">>> Object detection >>>"
        # ">>> Yaw >>>"
        # ">>> Ultrasonic Sensors Detect >>>"
        # ">>> Encoders >>>"
        # ">>> Stepper position >>>"
        # ">>State Logic  >>"
      }
      frame "RESET ENCODERS" {
        # ">>> Object detection >>>"
        # ">>> Yaw >>>"
        # ">>> Ultrasonic Sensors Detect >>>"
        # ">>> Encoders >>>"
        # ">>> Stepper position >>>"
        # ">>State Logic  >>"
        n100 = call "MOTOR CONTROL WITH PID AE.vi"("Direction"=MOTOR_CONTROL_WITH_PID_AE_DIRECTION_TYPE_DEF."reset encoders", "AE Mode"=MOTOR_CONTROL_WITH_PID_AE_DATA_MODE_TYPE_DEF."Write to AE") -> ()  [unwired: 2 in, 1 out]
      }
      frame "RESET FLAGS" {
        (unwired) I2C_MASTER_Type_Def."Last State" ("Arduino Mode")
        # "Resets any software variables\nand/or non-critical states"
        n101 = Wait (ms)(milliseconds to wait=u32 20) -> ()  [unwired: 1 out]
        n102 = Bundle By Name(cluster=w2176, "Time up flag"=FALSE, "SET TIME TO CHECK"=0.0) -> (w2175:T11)
        n103 = Bundle By Name(cluster=w2193, "Recognized Object"=FALSE, "Object X coordinate"=0.0, "Object Y coordinate"=0.0) -> (w2192:T15)
        n104 = Bundle By Name(cluster=w2183, "y Stepper Position"=u8 0, "z Stepper Position"=u8 0) -> (w2182:T13)
        n105 = Bundle By Name(cluster=w2188, "xDistance"=0.0, "yDistance"=0.0, "wDistance"=0.0) -> (w2187:T17)
        n106 = Bundle By Name(cluster=w2200, "PING_A"=u8 0, "PING_B"=u8 0, "PING_C"=u8 0, "PING_D"=u8 0) -> (w2199:T16)
        n107 = Bundle By Name(cluster=w2179, "Yaw"=0.0) -> (w2178:T12)
      }
      frame "RESET YAW" {
        n108 = Wait (ms)(milliseconds to wait=u32 100) -> ()  [unwired: 1 out]
        n109 = call "navX reading VI.vi"("Mode"=navX_type_def."Zero Yaw") -> ()  [unwired: 2 in, 4 out]
      }
      frame "RESET ARM" {
        n110 = call "Arduino Interfacing VI.vi"("Data to Write"=I2C_MASTER_WRITE_NEW_Type_Def."Soft Reset", "AE Mode"=Arduino_Interfacing."Write to Arduino") -> ()  [unwired: 2 in, 2 out]
      }
      frame "--------CAM STATES-------" {
      }
      frame "OPEN LOG CAM" {
        n111 = call "Webcam AE.vi"("Session In"=T32 "cam0", "Camera states"=Webcam_AE."Initialize Camera") -> ("error out"=w2233:errorcluster, "Session Out"=w2232:T32)  [unwired: 1 in, 1 out]
        n112 = call "Webcam AE.vi"("error in (no error)"=w2233, "Session In"=w2232, "Camera states"=Webcam_AE."Open Camera") -> ()  [unwired: 3 out]
      }
      frame "OPEN LIFE CAM" {
        n113 = call "Webcam AE.vi"("Session In"=T32 "cam1", "Camera states"=Webcam_AE."Initialize Camera") -> ("error out"=w2246:errorcluster, "Session Out"=w2245:T32)  [unwired: 1 in, 1 out]
        n114 = call "Webcam AE.vi"("error in (no error)"=w2246, "Session In"=w2245, "Camera states"=Webcam_AE."Open Camera") -> ()  [unwired: 3 out]
      }
      frame "CAM ACQ" {
        # ">>State Logic  >>"
        # ">>> Time cluster >>>"
        # ">>> Yaw >>>"
        # ">>> Stepper position >>>"
        # ">>> Encoders >>>"
        # ">>> Object detection >>>"
        # ">>> Ultrasonic Sensors Detect >>>"
        n115 = call "Webcam AE.vi"("error in (no error)"=w2257, "Camera states"=Webcam_AE."Continuous Acquisition") -> ()  [unwired: 1 in, 3 out]
      }
      frame "CAM CLOSE" {
        # ">>State Logic  >>"
        # ">>> Time cluster >>>"
        # ">>> Yaw >>>"
        # ">>> Stepper position >>>"
        # ">>> Encoders >>>"
        # ">>> Object detection >>>"
        # ">>> Ultrasonic Sensors Detect >>>"
        n116 = call "Webcam AE.vi"("Camera states"=Webcam_AE."Close Camera") -> ()  [unwired: 2 in, 3 out]
      }
      frame "PROCESS IMAGE" {
        # ">>State Logic  >>"
        # ">>> Time cluster >>>"
        # ">>> Yaw >>>"
        # ">>> Stepper position >>>"
        # ">>> Encoders >>>"
        # ">>> Object detection >>>"
        # ">>> Ultrasonic Sensors Detect >>>"
        n117 = call "Webcam AE.vi"("error in (no error)"=w2287, "Camera states"=Webcam_AE."Retrieve Image") -> ("error out"=w2283:errorcluster, "Image Out"=w2286:T25)  [unwired: 1 in, 1 out]
        n118 = call "Object Detection SubVI.vi"("Error In"=w2283, "Mode"="Object recognition mode", "Image Dest"=w2285, "Image in"=w2286) -> ("Object Center Coordinates"=w2280:cluster{"x":sgl, "y":sgl}, "Object detection cluster"=w2276:T2)  [unwired: 2 out]
        "Object detection cluster" <- w2276
        "Object Center Coordinates" <- w2280
        n119 = Unbundle By Name(w2276) -> ("Object detected?"=w2277:bool)
        n120 = Unbundle By Name(w2280) -> ("x"=w2279:sgl, "y"=w2278:sgl)
        n121 = Bundle By Name(cluster=w2282, "Recognized Object"=w2277, "Object X coordinate"=w2279, "Object Y coordinate"=w2278) -> (w2281:T15)
      }
      frame "DISPOSE BUFFERS" {
        # ">>State Logic  >>"
        # ">>> Time cluster >>>"
        # ">>> Yaw >>>"
        # ">>> Stepper position >>>"
        # ">>> Encoders >>>"
        # ">>> Object detection >>>"
        # ">>> Ultrasonic Sensors Detect >>>"
        n122 = call "Webcam AE.vi"("error in (no error)"=w2297, "Camera states"=Webcam_AE."Dispose Image Buffers") -> ()  [unwired: 1 in, 3 out]
      }
      frame "-----ARM ACTIONS-----" {
      }
      frame "CLOSE CLAW" {
        n123 = call "Arduino Interfacing VI.vi"("Data to Write"=I2C_MASTER_WRITE_NEW_Type_Def."Close Claw", "AE Mode"=Arduino_Interfacing."Write to Arduino") -> ()  [unwired: 2 in, 2 out]
      }
      frame "OPEN CLAW" {
        n124 = call "Arduino Interfacing VI.vi"("Data to Write"=I2C_MASTER_WRITE_NEW_Type_Def."Open Claw", "AE Mode"=Arduino_Interfacing."Write to Arduino") -> ()  [unwired: 2 in, 2 out]
      }
      frame "Z STEPPER CAM HEIGHT" {
        n125 = call "Arduino Interfacing VI.vi"("Data to Write"=I2C_MASTER_WRITE_NEW_Type_Def."zStepper 6k", "AE Mode"=Arduino_Interfacing."Write to Arduino") -> ()  [unwired: 2 in, 2 out]
      }
      frame "Z STEPPER GRAB HEIGHT" {
        # ">>State Logic  >>"
        # ">>> Time cluster >>>"
        # ">>> Yaw >>>"
        # ">>> Stepper position >>>"
        # ">>> Encoders >>>"
        # ">>> Object detection >>>"
        # ">>> Ultrasonic Sensors Detect >>>"
        n126 = call "Arduino Interfacing VI.vi"("Data to Write"=I2C_MASTER_WRITE_NEW_Type_Def."zStepper 100", "AE Mode"=Arduino_Interfacing."Write to Arduino") -> ()  [unwired: 2 in, 2 out]
      }
      frame "Y STEPPER CONTROL" {
        # ">>State Logic  >>"
        # ">>> yStepper command>>>"
        # ">>> Time cluster >>>"
        # ">>> Yaw >>>"
        # ">>> Stepper position >>>"
        # ">>> Encoders >>>"
        # ">>> Object detection >>>"
        # ">>> Ultrasonic Sensors Detect >>>"
        n127 = Unbundle By Name(w2355) -> ("yStepper desired"=w2354:u8)
        n128 = call "Arduino Interfacing VI.vi"("y Stepper value"=w2354, "Data to Write"=I2C_MASTER_WRITE_NEW_Type_Def."yStepper control", "AE Mode"=Arduino_Interfacing."Write to Arduino") -> ()  [unwired: 1 in, 2 out]
      }
      frame "READ STEPPER VALUES" {
        # ">>State Logic  >>"
        # ">>> Time cluster >>>"
        # ">>> Yaw >>>"
        # ">>> Stepper position >>>"
        # ">>> Encoders >>>"
        # ">>> Object detection >>>"
        # ">>> Ultrasonic Sensors Detect >>>"
        n129 = call "Arduino Interfacing VI.vi"("AE Mode"=Arduino_Interfacing."Read From Arduino") -> ("Arduino Data"=w2370:T4)  [unwired: 3 in, 1 out]
        n130 = Unbundle By Name(w2370) -> ("y Stepper Position"=w2369:u8, "z Stepper Position"=w2368:u8)
        n131 = Bundle By Name(cluster=w2373, "y Stepper Position"=w2369, "z Stepper Position"=w2368) -> (w2372:T13)
      }
      frame " -----TIMING-----" {
        # ">>State Logic  >>"
        # ">>> Time cluster >>>"
        # ">>> Yaw >>>"
        # ">>> Stepper position >>>"
        # ">>> Encoders >>>"
        # ">>> Object detection >>>"
        # ">>> Ultrasonic Sensors Detect >>>"
      }
      frame "SET TIMER 1" {
        # ">>State Logic  >>"
        # ">>> Time cluster >>>"
        # ">>> Yaw >>>"
        # ">>> Stepper position >>>"
        # ">>> Encoders >>>"
        # ">>> Object detection >>>"
        # ">>> Ultrasonic Sensors Detect >>>"
        n132 = call "Elasped Timer.vi"("Time Setting"=1.0, "Action"=Elapsed_timer_control."Initialize") -> ()  [unwired: 6 in, 4 out]
        n133 = Bundle By Name(cluster=w2391, "Time up flag"=FALSE) -> (w2389:T11)
      }
      frame "SET TIMER 2" {
        # ">>State Logic  >>"
        # ">>> Time cluster >>>"
        # ">>> Yaw >>>"
        # ">>> Stepper position >>>"
        # ">>> Encoders >>>"
        # ">>> Object detection >>>"
        # ">>> Ultrasonic Sensors Detect >>>"
        n134 = call "Elasped Timer.vi"("Time Setting"=2.0, "Action"=Elapsed_timer_control."Initialize") -> ()  [unwired: 6 in, 4 out]
        n135 = Bundle By Name(cluster=w2403, "Time up flag"=FALSE) -> (w2401:T11)
      }
      frame "SET TIMER 3" {
        # ">>State Logic  >>"
        # ">>> Time cluster >>>"
        # ">>> Yaw >>>"
        # ">>> Stepper position >>>"
        # ">>> Encoders >>>"
        # ">>> Object detection >>>"
        # ">>> Ultrasonic Sensors Detect >>>"
        n136 = call "Elasped Timer.vi"("Time Setting"=3.0, "Action"=Elapsed_timer_control."Initialize") -> ()  [unwired: 6 in, 4 out]
        n137 = Bundle By Name(cluster=w2415, "Time up flag"=FALSE) -> (w2413:T11)
      }
      frame "SET TIMER 4" {
        # ">>State Logic  >>"
        # ">>> Time cluster >>>"
        # ">>> Yaw >>>"
        # ">>> Stepper position >>>"
        # ">>> Encoders >>>"
        # ">>> Object detection >>>"
        # ">>> Ultrasonic Sensors Detect >>>"
        n138 = call "Elasped Timer.vi"("Time Setting"=4.0, "Action"=Elapsed_timer_control."Initialize") -> ()  [unwired: 6 in, 4 out]
        n139 = Bundle By Name(cluster=w2427, "Time up flag"=FALSE) -> (w2425:T11)
      }
      frame "SET TIMER 5" {
        # ">>State Logic  >>"
        # ">>> Time cluster >>>"
        # ">>> Yaw >>>"
        # ">>> Stepper position >>>"
        # ">>> Encoders >>>"
        # ">>> Object detection >>>"
        # ">>> Ultrasonic Sensors Detect >>>"
        n140 = call "Elasped Timer.vi"("Time Setting"=5.0, "Action"=Elapsed_timer_control."Initialize") -> ()  [unwired: 6 in, 4 out]
        n141 = Bundle By Name(cluster=w2439, "Time up flag"=FALSE) -> (w2437:T11)
      }
      frame "START TIMER" {
        # ">>State Logic  >>"
        # ">>> Time cluster >>>"
        # ">>> Yaw >>>"
        # ">>> Stepper position >>>"
        # ">>> Encoders >>>"
        # ">>> Object detection >>>"
        # ">>> Ultrasonic Sensors Detect >>>"
        n142 = call "Elasped Timer.vi"("Action"=Elapsed_timer_control."Start") -> ("Time Out?!"=w2447:bool)  [unwired: 7 in, 3 out]
        n143 = Bundle By Name(cluster=w2450, "Time up flag"=w2447) -> (w2449:T11)
      }
    }
    "State Logic" <- w215
    n144 = local read "TASK ENABLE"() -> (w209:bool)
    n145 = Not(x=w209) -> (.not. x?=w208:bool)
    n146 = case shown="True" w216 {
      tunnel: w220 -> [w245 w280]
      tunnel: w224 -> [w241 w282]
      tunnel: [w245 w280] -> w229
      tunnel: [w241 w283] -> w228
      tunnel: w225 -> [_ w278]
      tunnel: w227 -> [_ w279]
      tunnel: w222 -> [w244 w285]
      tunnel: [w244 w285] -> w221
      tunnel: "STOP TASK" -> [_ w268]
      tunnel: w215 -> [w243 w284]
      tunnel: [w243 w281] -> w214
      tunnel: w211 -> [w242 w274]
      tunnel: [w242 w274] -> w210
      tunnel: w208 -> [_ w269]
      tunnel: [w240 w266] -> w207
      tunnel: w206 -> [w240 w265]
      tunnel: w202 -> [w239 w262]
      tunnel: [w239 w262] -> w201
      tunnel: w199 -> [w238 w258]
      tunnel: [w238 w258] -> w198
      tunnel: w196 -> [w237 w256]
      tunnel: [w237 w256] -> w195
      tunnel: w193 -> [w236 w254]
      tunnel: [w236 w254] -> w192
      tunnel: w191 -> [w235 w253]
      tunnel: [w235 w252] -> w190
      tunnel: [_ w250] -> w189
      tunnel: w187 -> [w234 w248]
      tunnel: [w234 w248] -> w186
      tunnel: w185 -> [w233 w247]
      tunnel: [w233 w246] -> w184
      frame False {
        # ">>> Motor control cluster >>>"
        # ">>> yStepper command>>>"
        # ">>> Motor control cluster >>>"
        # ">>> yStepper command>>>"
        # ">>> Motor control cluster >>>"
        # ">>> IR Sensors >>>"
        # ">>> IR Sensors >>>"
        # ">>> yStepper command>>>"
        # ">>> Time cluster >>>"
        # ">>> Yaw >>>"
        # ">>> Stepper position >>>"
        # ">>> Encoders >>>"
        # ">>> Object detection >>>"
        # ">>> Ultrasonic Sensors Detect >>>"
        # ">>> Time cluster >>>"
        # ">>> Yaw >>>"
        # ">>> Stepper position >>>"
        # ">>> Encoders >>>"
        # ">>> Object detection >>>"
        # ">>> Ultrasonic Sensors Detect >>>"
      }
      frame True {
        # ">>> Motor control cluster >>>"
        # ">>> yStepper command>>>"
        # ">>> IR Sensors >>>"
        # ">>> Motor control cluster >>>"
        # ">>State Logic Queue Reference >>"
        # ">>Timeout>>"
        # ">>> yStepper command>>>"
        # ">>> Time cluster >>>"
        # ">>> Object detection >>>"
        # ">>> Yaw >>>"
        # ">>> Ultrasonic Sensors Detect >>>"
        # ">>> Encoders >>>"
        # ">>> Stepper position >>>"
        # ">>State Logic  >>"
        # ">>True Stop Next State >>"
        # ">>Action Queue>>"
        # ">> Manual override >>"
        # ">>> Time cluster >>>"
        # ">>> Yaw >>>"
        # ">>> Stepper position >>>"
        # ">>> Encoders >>>"
        # ">>> Object detection >>>"
        # ">>> Ultrasonic Sensors Detect >>>"
        # ">>Action Queue>>"
        # ">>State Logic Queue Reference >>"
        n147 = Or(x=w268, y=w269) -> (x .or. y?=w267:bool)
        n148 = Unbundle By Name(w248) -> ("Left IR Sensor"=w249:dbl)
        "Left IR Sensor" <- w249
        n149 = Unbundle By Name(w254) -> ("Time up flag"=w255:bool)
        "Time up flag" <- w255
        n150 = Unbundle By Name(w256) -> ("Yaw"=w257:dbl, "Compass"=w251:dbl)
        n151 = Unbundle By Name(w258) -> ("y Stepper Position"=w260:u8, "z Stepper Position"=w259:u8)
        n152 = Unbundle By Name(w274) -> ("xDistance"=w271:dbl, "yDistance"=w272:dbl, "wDistance"=w273:dbl)
        n153 = Unbundle By Name(w262) -> ("Recognized Object"=w261:bool, "Object X coordinate"=w264:dbl, "Object Y coordinate"=w263:dbl)
        n154 = Unbundle By Name(w285) -> ("PING_A"=w277:u8, "PING_B"=w276:u8, "PING_C"=w275:u8, "PING_D"=w270:u8)
        n155 = case shown="29" w284 {
          tunnel: [w289 w300 w313 w323 w398 w412 w448 w501 w543 w590 w633 w687 w734 w774 w834 w879 w919 w967 w1009 w1061 w1098 w1149 w1192 w1235 w1264 w1271 w1319 w1360 w1411 w1456 w1496 w1544 w1597 w1635 w1683 w1725 w1777 w1814 w1865] -> w283
          tunnel: w282 -> [w289 w303 w314 w326 w400 w413 w457 w499 w547 w591 w639 w680 w737 w781 w824 w882 w925 w966 w1012 w1051 w1104 w1139 w1187 w1226 w1264 w1275 w1326 w1365 w1401 w1459 w1502 w1543 w1596 w1641 w1682 w1728 w1767 w1820 w1855]
          tunnel: [State_Type_Definitions,_for_0.26g_versions_and_later_2."Idle" ("Enum") State_Type_Definitions,_for_0.26g_versions_and_later_2."Idle" ("Enum") w309 w325 State_Type_Definitions,_for_0.26g_versions_and_later_2."Shutdown" ("Enum") w414 w455 w502 w544 w589 w634 w686 w735 w776 w833 w880 w926 w968 w1011 w1060 w1105 w1148 w1193 w1227 State_Type_Definitions,_for_0.26g_versions_and_later_2."Idle" ("Enum") w1272 w1320 w1361 w1410 w1457 w1503 w1545 w1598 w1642 w1684 w1727 w1776 w1821 w1864] -> w281
          tunnel: w280 -> [_ _ w312 w329 _ w419 w451 w498 w548 w598 w638 w684 w738 w780 w831 w877 w924 w964 w1013 w1058 w1103 w1146 w1190 w1234 _ w1279 w1325 w1368 w1408 w1454 w1501 w1541 w1594 w1640 w1680 w1729 w1774 w1819 w1862]
          tunnel: w279 -> [_ _ _ w328 _ w418 w450 w497 w549 w597 w637 w683 w731 w779 w830 w876 w923 w963 w1014 w1057 w1102 w1145 w1189 w1232 _ w1274 w1324 w1367 w1407 w1453 w1500 w1540 w1593 w1639 w1679 w1730 w1773 w1818 w1861]
          tunnel: w278 -> [_ _ w311 w324 _ w417 w449 w496 w550 w596 w636 w682 w730 w778 w832 w878 w922 w962 w1015 w1059 w1101 w1147 w1188 w1233 _ w1278 w1323 w1366 w1409 w1455 w1499 w1539 w1592 w1638 w1678 w1731 w1775 w1817 w1863]
          tunnel: w267 -> [_ _ _ _ _ w411 w456 w495 w551 w593 w632 w685 w736 w782 w825 w883 w920 w965 w1016 w1052 w1099 w1140 w1191 w1230 _ w1277 w1318 w1364 w1402 w1460 w1497 w1542 w1595 w1636 w1681 w1732 w1768 w1815 w1856]
          tunnel: w277 -> [_ _ _ _ _ _ _ _ _ _ _ _ _ _ _ _ _ _ _ _ _ _ _ _ _ _ _ _ _ _ _ _ _ _ _ _ _ _ _]
          tunnel: w276 -> [_ _ _ _ _ _ _ w494 _ _ _ w676 w719 w772 _ w869 _ _ _ _ _ _ _ _ _ _ _ _ _ w1446 _ _ _ _ _ _ _ _ _]
          tunnel: w275 -> [_ _ _ _ _ _ _ w493 _ _ _ w677 w720 w773 _ w870 _ _ _ _ _ _ _ _ _ _ _ _ _ w1447 _ _ _ _ _ _ _ _ _]
          tunnel: w273 -> [_ _ _ _ _ _ _ _ _ w595 _ _ _ _ _ _ _ _ _ _ _ _ _ _ _ _ _ _ _ _ _ _ _ _ _ _ _ _ _]
          tunnel: w272 -> [_ _ _ _ _ w410 _ _ w542 _ _ _ _ w777 _ _ _ _ _ _ _ _ _ _ _ _ _ _ _ _ _ _ _ _ _ _ _ _ _]
          tunnel: w271 -> [_ _ _ _ _ _ _ _ _ _ _ _ w725 _ _ _ _ _ _ _ _ _ _ _ _ _ _ _ _ _ _ _ w1580 _ _ _ _ _ _]
          tunnel: w270 -> [_ _ _ _ _ _ _ _ _ _ _ _ _ _ _ _ _ _ _ _ _ _ _ _ _ _ _ _ _ _ _ _ _ _ _ _ _ _ _]
          tunnel: [State_Type_Definitions,_for_0.26g_versions_and_later_2."Idle" ("Enum") State_Type_Definitions,_for_0.26g_versions_and_later_2."Idle" ("Enum") State_Type_Definitions,_for_0.26g_versions_and_later_2."Idle" ("Enum") State_Type_Definitions,_for_0.26g_versions_and_later_2."Idle" ("Enum") State_Type_Definitions,_for_0.26g_versions_and_later_2."Shutdown" ("Enum") w407 w454 w500 w545 w586 w631 w679 w733 w775 w835 w881 w918 w969 w1010 w1062 w1097 w1150 w1194 w1228 w1266 w1273 w1321 w1363 w1412 w1458 w1495 w1546 w1599 w1634 w1685 w1726 w1778 w1813 w1866] -> w266
          tunnel: w265 -> [_ _ w309 _ _ _ _ _ _ _ _ _ _ _ _ _ _ _ _ _ _ _ _ _ w1266 _ _ _ _ _ _ _ _ _ _ _ _ _ _]
          tunnel: w261 -> [_ _ _ _ _ _ _ _ _ _ _ _ _ _ _ _ _ _ _ _ _ _ _ w1229 _ _ _ _ _ _ _ _ _ _ _ _ _ _ _]
          tunnel: w264 -> [_ _ _ _ _ _ _ _ _ _ _ _ _ _ _ _ _ _ _ _ _ _ _ _ _ _ _ _ _ _ _ _ w1589 _ _ _ _ _ _]
          tunnel: w263 -> [_ _ _ _ _ _ _ _ _ _ _ _ _ _ _ _ _ _ w1005 _ _ _ _ _ _ _ _ _ _ _ _ _ _ _ _ w1721 _ _ _]
          tunnel: w260 -> [_ _ _ _ _ _ _ _ _ _ _ _ _ _ _ _ _ _ w1004 _ _ _ _ _ _ _ _ _ _ _ _ _ _ _ _ w1720 _ _ _]
          tunnel: w259 -> [_ _ _ _ _ _ w453 _ _ _ w629 _ _ _ w828 _ _ _ _ w1055 _ w1143 w1186 _ _ w1276 _ _ w1405 _ _ _ _ _ _ _ w1771 _ w1859]
          tunnel: w257 -> [_ _ _ _ _ _ _ _ _ _ _ _ _ _ _ _ _ _ _ _ _ _ _ _ _ _ _ _ _ _ _ _ _ _ _ _ _ _ _]
          tunnel: w255 -> [_ _ _ _ _ _ _ _ _ _ _ _ _ _ _ _ w916 w959 _ _ w1095 _ _ _ _ _ _ _ _ _ w1493 w1536 _ w1632 w1675 _ _ w1811 _]
          tunnel: w253 -> [w287 w298 w308 w321 w396 w406 w452 w492 w546 w585 w630 w678 w729 w771 w823 w874 w917 w960 w1007 w1050 w1096 w1138 w1183 w1225 w1267 w1270 w1322 w1362 w1400 w1451 w1494 w1537 w1590 w1633 w1676 w1723 w1766 w1812 w1854]
          tunnel: [w287 w297 w308 w321 w396 w406 w452 w492 w546 w585 w630 w678 w729 w771 w823 w874 w917 w960 w1006 w1050 w1096 w1138 w1183 w1225 w1267 w1270 w1322 w1362 w1400 w1451 w1494 w1537 w1590 w1633 w1676 w1722 w1766 w1812 w1854] -> w252
          tunnel: w251 -> [_ _ _ _ _ _ _ _ _ _ _ _ _ _ _ _ _ _ _ _ _ _ _ _ _ _ w1317 _ _ _ _ _ _ _ _ _ _ _ _]
          tunnel: [_ _ _ TRUE _ _ _ _ _ _ _ _ _ _ _ _ _ _ _ _ _ _ _ _ _ _ _ _ _ _ _ _ _ _ _ _ _ _ _] -> w250
          tunnel: w249 -> [_ _ _ _ _ _ _ _ _ _ _ _ _ _ _ _ _ _ _ _ _ _ _ _ _ _ _ _ _ _ _ _ _ _ _ _ _ _ _]
          tunnel: w247 -> [w286 w295 w307 w319 w395 w405 w447 w491 w539 w584 w626 w671 w718 w770 w822 w867 w915 w958 w1001 w1049 w1094 w1137 w1182 w1224 w1268 w1269 w1313 w1359 w1399 w1444 w1492 w1535 w1586 w1631 w1674 w1717 w1765 w1810 w1853]
          tunnel: [w286 w294 w307 w319 w395 w405 w447 w491 w539 w584 w626 w671 w718 w770 w822 w867 w915 w958 w1001 w1049 w1094 w1137 w1182 w1224 w1268 w1269 w1313 w1359 w1399 w1444 w1492 w1535 w1585 w1631 w1674 w1717 w1765 w1810 w1853] -> w246
          frame 0 {
            # ">>> yStepper command>>>"
          }
          frame 1 {
            # ">>> yStepper command>>>"
            n156 = for {
              shift-right: [w306] -> w300
              shift-left: w303 -> [w305]
              tunnel: string[] ["INIT", "RESET ARM", "RESET FLAGS", "RESET YAW", "NAVX CALIBRATE"] -> [w304] mode=indexing
              n157 = Enqueue Element(queue=w305, element=w304) -> (queue out=w306:refnum<queue>)  [unwired: 2 in, 2 out]
            }
            n158 = Bundle By Name(cluster=w298, "yStepper desired"=u8 0) -> (w297:T10)
            n159 = Bundle By Name(cluster=w295, "ySpeed"=0.0, "xSpeed"=0.0, "wSpeed"=0.0) -> (w294:T8)
          }
          frame 3 {
            # ">>> yStepper command>>>"
            n160 = Flush Queue(queue=w312, error in (no error)=w311) -> ()  [unwired: 3 out]
            n161 = for {
              shift-right: [w318] -> w313
              shift-left: w314 -> [w317]
              tunnel: string[] ["STOP", "RESET ENCODERS", "RESET YAW", "RESET ARM", "RESET FLAGS", "DISPOSE BUFFERS", "CAM CLOSE"] -> [w316] mode=indexing
              n162 = Enqueue Element(queue=w317, element=w316) -> (queue out=w318:refnum<queue>)  [unwired: 2 in, 2 out]
            }
          }
          frame 4, Default {
            (unwired) TRUE ("Green LED")
            # ">>> yStepper command>>>"
            n163 = Dequeue Element(queue=w329, timeout in ms (-1)=w328, error in (no error)=w324) -> (element=w327:T7)  [unwired: 3 out]
            n164 = case shown="\"Start Task 4\"" w327 {
              tunnel: [w331 w338 w345 w352 w359 w366 w373 w375 w383 w389] -> w323
              tunnel: w326 -> [w332 w339 w346 w353 w360 w367 w373 w376 w382 w390]
              tunnel: [State_Type_Definitions."Task 1" ("Enum") State_Type_Definitions,_for_0.26g_versions_and_later_2."Task 2:Raise Arm" ("Enum") State_Type_Definitions,_for_0.26g_versions_and_later_2."Task 3" ("Enum") State_Type_Definitions,_for_0.26g_versions_and_later_2."Task 4_A" ("Enum") State_Type_Definitions."Task 5A: ARM CAM HEIGHT" ("Enum") State_Type_Definitions,_for_0.26g_versions_and_later_2."Task 6_A" ("Enum") State_Type_Definitions,_for_0.26g_versions_and_later_2."Idle" ("Enum") State_Type_Definitions,_for_0.26g_versions_and_later_2."Shutdown" ("Enum") State_Type_Definitions,_for_0.26g_versions_and_later_2."Task 9A: Raise Arm" ("Enum") State_Type_Definitions,_for_0.26g_versions_and_later_2."Task 8A: RAISE ARM" ("Enum")] -> w325
              frame "Start Task 1" {
                n165 = for {
                  shift-right: [w336] -> w331
                  shift-left: w332 -> [w335]
                  tunnel: string[] ["RESET ENCODERS", "RESET YAW", "FORWARD", "READ ENCODERS"] -> [w334] mode=indexing
                  n166 = Enqueue Element(queue=w335, element=w334) -> (queue out=w336:refnum<queue>)  [unwired: 2 in, 2 out]
                }
              }
              frame "Start Task 2" {
                n167 = for {
                  shift-right: [w343] -> w338
                  shift-left: w339 -> [w342]
                  tunnel: string[] ["RESET ENCODERS", "RESET YAW", "READ ULTRASONIC", "ARDUINO - ULTRASONIC"] -> [w341] mode=indexing
                  n168 = Enqueue Element(queue=w342, element=w341) -> (queue out=w343:refnum<queue>)  [unwired: 2 in, 2 out]
                }
              }
              frame "Start Task 3" {
                n169 = for {
                  shift-right: [w350] -> w345
                  shift-left: w346 -> [w349]
                  tunnel: string[] ["RESET ENCODERS", "READ ENCODERS", "R-ACW"] -> [w348] mode=indexing
                  n170 = Enqueue Element(queue=w349, element=w348) -> (queue out=w350:refnum<queue>)  [unwired: 2 in, 2 out]
                }
              }
              frame "Start Task 4" {
                n171 = for {
                  shift-right: [w357] -> w352
                  shift-left: w353 -> [w356]
                  tunnel: string[] ["RESET YAW", "RESET ENCODERS", "RESET ARM", "RESET FLAGS", "", ""] -> [w355] mode=indexing
                  n172 = Enqueue Element(queue=w356, element=w355) -> (queue out=w357:refnum<queue>)  [unwired: 2 in, 2 out]
                }
              }
              frame "Start Task 5" {
                n173 = for {
                  shift-right: [w364] -> w359
                  shift-left: w360 -> [w363]
                  tunnel: string[] ["RESET YAW", "RESET ENCODERS", "READ STEPPER VALUES", "Z STEPPER CAM HEIGHT", "", ""] -> [w362] mode=indexing
                  n174 = Enqueue Element(queue=w363, element=w362) -> (queue out=w364:refnum<queue>)  [unwired: 2 in, 2 out]
                }
              }
              frame "Start Task 6" {
                n175 = for {
                  shift-right: [w371] -> w366
                  shift-left: w367 -> [w370]
                  tunnel: string[] ["OPEN LOG CAM ", "", "", "", "", ""] -> [w369] mode=indexing
                  n176 = Enqueue Element(queue=w370, element=w369) -> (queue out=w371:refnum<queue>)  [unwired: 2 in, 2 out]
                }
              }
              frame "None", Default {
              }
              frame "Exit" {
                n177 = for {
                  shift-right: [w380] -> w375
                  shift-left: w376 -> [w379]
                  tunnel: string[] ["STOP", "RESET ENCODERS", "RESET YAW", "EXIT"] -> [w378] mode=indexing
                  n178 = Enqueue Element(queue=w379, element=w378) -> (queue out=w380:refnum<queue>)  [unwired: 2 in, 2 out]
                }
              }
              frame "Start Task 9" {
                n179 = for {
                  shift-right: [w387] -> w383
                  shift-left: w382 -> [w386]
                  tunnel: string[] ["RESET ENCODERS", "READ ENCODERS", "Z STEPPER CAM HEIGHT"] -> [w385] mode=indexing
                  n180 = Enqueue Element(queue=w386, element=w385) -> (queue out=w387:refnum<queue>)  [unwired: 2 in, 2 out]
                }
              }
              frame "Start Task 8 - BALL" {
                n181 = for {
                  shift-right: [w394] -> w389
                  shift-left: w390 -> [w393]
                  tunnel: string[] ["RESET YAW", "RESET ENCODERS", "RESET ARM", "RESET FLAGS"] -> [w392] mode=indexing
                  n182 = Enqueue Element(queue=w393, element=w392) -> (queue out=w394:refnum<queue>)  [unwired: 2 in, 2 out]
                }
              }
            }
          }
          frame 5 {
            # ">>> yStepper command>>>"
            n183 = for {
              shift-right: [w404] -> w398
              shift-left: w400 -> [w403]
              tunnel: string[] ["INIT", "RESET ENCODERS", "RESET FLAGS", "CAM CLOSE", "DISPOSE BUFFERS", "EXIT", ""] -> [w402] mode=indexing
              n184 = Enqueue Element(queue=w403, element=w402) -> (queue out=w404:refnum<queue>)  [unwired: 2 in, 2 out]
            }
          }
          frame 6 {
            # ">>> yStepper command>>>"
            # "Use 250"
            n185 = Dequeue Element(queue=w419, timeout in ms (-1)=w418, error in (no error)=w417) -> (element=w416:T7)  [unwired: 3 out]
            n186 = Greater?(x=w410, y=265.0) -> (0:w408:bool)
            n187 = Or(x=w408, y=w411) -> (x .or. y?=w415:bool)
            n188 = case shown="\"None\", Default" w416 {
              tunnel: w415 -> [w422 _]
              tunnel: [w426 State_Type_Definitions,_for_0.26g_versions_and_later_2."True Stop" ("Enum")] -> w414
              tunnel: w413 -> [w423 w441]
              tunnel: [w421 w440] -> w412
              tunnel: [State_Type_Definitions,_for_0.26g_versions_and_later_2."Idle" ("Enum") State_Type_Definitions,_for_0.26g_versions_and_later_2."Shutdown" ("Enum")] -> w407
              frame "None", Default {
                n189 = case shown="True" w422 {
                  tunnel: w423 -> [w429 w435]
                  tunnel: [w428 w433] -> w421
                  frame False {
                    n190 = for {
                      shift-right: [w431] -> w428
                      shift-left: w429 -> [w432]
                      tunnel: string[] ["READ ENCODERS", "READ NAVX", "FORWARD"] ("element") -> [w430] mode=indexing
                      n191 = Enqueue Element(queue=w432, element=w430) -> (queue out=w431:refnum<queue>)  [unwired: 2 in, 2 out]
                    }
                  }
                  frame True {
                    n192 = for {
                      shift-right: [w437] -> w433
                      shift-left: w435 -> [w438]
                      tunnel: string[] ["RESET YAW", "RESET ENCODERS", "STOP", ""] -> [w436] mode=indexing
                      n193 = Enqueue Element(queue=w438, element=w436) -> (queue out=w437:refnum<queue>)  [unwired: 2 in, 2 out]
                    }
                  }
                }
                n194 = Select(t=State_Type_Definitions,_for_0.26g_versions_and_later_2."True Stop" ("Enum"), s=w422, f=State_Type_Definitions."Task 1" ("Enum")) -> (s? t:f=w426:u16)
              }
              frame "Exit" {
                n195 = for {
                  shift-right: [w445] -> w440
                  shift-left: w441 -> [w446]
                  tunnel: string[] ["STOP", "RESET ENCODERS", "RESET YAW", ""] -> [w444] mode=indexing
                  n196 = Enqueue Element(queue=w446, element=w444) -> (queue out=w445:refnum<queue>)  [unwired: 2 in, 2 out]
                }
              }
            }
          }
          frame 8 {
            # ">> Stepper height reeached >>"
            # ">>> yStepper command>>>"
            # ">> Manual override >>"
            n197 = Dequeue Element(queue=w451, timeout in ms (-1)=w450, error in (no error)=w449) -> (element=w460:T7)  [unwired: 3 out]
            n198 = Equal?(x=w453, y=u8 60) -> (x = y?=w458:bool)
            n199 = case shown="\"None\", Default" w460 {
              tunnel: [w471 State_Type_Definitions,_for_0.26g_versions_and_later_2."True Stop" ("Enum")] -> w455
              tunnel: [w469 w486] -> w448
              tunnel: w457 -> [w468 _]
              tunnel: w456 -> [w462 _]
              tunnel: [State_Type_Definitions,_for_0.26g_versions_and_later_2."Idle" ("Enum") State_Type_Definitions,_for_0.26g_versions_and_later_2."Shutdown" ("Enum")] -> w454
              tunnel: w458 -> [w461 _]
              frame "None", Default {
                # ">> WIill proceed to part ii if not manual override >>"
                # ">>If ENABLE or Trigger is set to true>>"
                n200 = Or(x=w461, y=w462) -> (x .or. y?=w463:bool)
                n201 = case shown="True" w461 {
                  tunnel: [w474 w480] -> w469
                  tunnel: w468 -> [w473 w479]
                  frame False {
                    n202 = for {
                      shift-right: [w476] -> w474
                      shift-left: w473 -> [w477]
                      tunnel: string[] ["Z STEPPER CAM HEIGHT", "READ STEPPER VALUES"] ("element") -> [w475] mode=indexing
                      n203 = Enqueue Element(queue=w477, element=w475) -> (queue out=w476:refnum<queue>)  [unwired: 2 in, 2 out]
                    }
                  }
                  frame True {
                    n204 = for {
                      shift-right: [w482] -> w480
                      shift-left: w479 -> [w483]
                      tunnel: string[] ["ARDUINO - ULTRASONIC", "READ ULTRASONIC", "", "", "", ""] -> [w481] mode=indexing
                      n205 = Enqueue Element(queue=w483, element=w481) -> (queue out=w482:refnum<queue>)  [unwired: 2 in, 2 out]
                    }
                  }
                }
                n206 = Select(t=State_Type_Definitions,_for_0.26g_versions_and_later_2."True Stop" ("Enum"), s=w462, f=State_Type_Definitions,_for_0.26g_versions_and_later_2."Task 2:Sensor Mode" ("Enum")) -> (s? t:f=w465:T6)
                n207 = Select(t=w465, s=w463, f=State_Type_Definitions,_for_0.26g_versions_and_later_2."Task 2:Raise Arm" ("Enum")) -> (s? t:f=w471:T6)
              }
              frame "Exit" {
                n208 = for {
                  shift-right: [w489] -> w486
                  shift-left: _ -> [w490]
                  tunnel: string[] ["STOP", "RESET ENCODERS", "RESET YAW", ""] -> [w488] mode=indexing
                  n209 = Enqueue Element(queue=w490, element=w488) -> (queue out=w489:refnum<queue>)  [unwired: 2 in, 2 out]
                }
              }
            }
          }
          frame 9 {
            w506 = u8 20 ("y")
            # ">>> yStepper command>>>"
            # ">>Object detected>>"
            n210 = Dequeue Element(queue=w498, timeout in ms (-1)=w497, error in (no error)=w496) -> (element=w507:T7)  [unwired: 3 out]
            n211 = Less?(x=w494, y=w506) -> (x < y?=w505:bool)
            n212 = Less?(x=w493, y=w506) -> (x < y?=w504:bool)
            n213 = Or(x=w505, y=w504) -> (x .or. y?=w503:bool)
            "Obstacle detected" <- w503
            n214 = case shown="\"None\", Default" w507 {
              tunnel: w503 -> [w510 _]
              tunnel: [w517 State_Type_Definitions,_for_0.26g_versions_and_later_2."True Stop" ("Enum")] -> w502
              tunnel: w495 -> [w509 _]
              tunnel: w499 -> [w516 w533]
              tunnel: [w515 w534] -> w501
              tunnel: [State_Type_Definitions,_for_0.26g_versions_and_later_2."Idle" ("Enum") State_Type_Definitions,_for_0.26g_versions_and_later_2."Shutdown" ("Enum")] -> w500
              frame "None", Default {
                n215 = case shown="True" w510 {
                  tunnel: w516 -> [w520 w527]
                  tunnel: [w521 w526] -> w515
                  frame False {
                    n216 = for {
                      tunnel: string[] ["READ ULTRASONIC", "STOP"] ("element") -> [w522] mode=indexing
                      shift-right: [w524] -> w521
                      shift-left: w520 -> [w523]
                      n217 = Enqueue Element(queue=w523, element=w522) -> (queue out=w524:refnum<queue>)  [unwired: 2 in, 2 out]
                    }
                  }
                  frame True {
                    n218 = for {
                      shift-right: [w529] -> w526
                      shift-left: w527 -> [w530]
                      tunnel: string[] ["RESET ENCODERS", "READ NAVX", "READ ENCODERS"] -> [w528] mode=indexing
                      n219 = Enqueue Element(queue=w530, element=w528) -> (queue out=w529:refnum<queue>)  [unwired: 2 in, 2 out]
                    }
                  }
                }
                n220 = Or(x=w510, y=w509) -> (x .or. y?=w508:bool)
                n221 = Select(t=State_Type_Definitions,_for_0.26g_versions_and_later_2."True Stop" ("Enum"), s=w509, f=State_Type_Definitions,_for_0.26g_versions_and_later_2."Task 2:Reverse Mode" ("Enum")) -> (s? t:f=w511:T6)
                n222 = Select(t=w511, s=w508, f=State_Type_Definitions,_for_0.26g_versions_and_later_2."Task 2:Sensor Mode" ("Enum")) -> (s? t:f=w517:T6)
              }
              frame "Exit" {
                n223 = for {
                  shift-right: [w537] -> w534
                  shift-left: w533 -> [w538]
                  tunnel: string[] ["STOP", "RESET ENCODERS", "RESET YAW", "ARDUINO MODE 0"] -> [w536] mode=indexing
                  n224 = Enqueue Element(queue=w538, element=w536) -> (queue out=w537:refnum<queue>)  [unwired: 2 in, 2 out]
                }
              }
            }
          }
          frame 10 {
            # ">>> yStepper command>>>"
            n225 = Dequeue Element(queue=w548, timeout in ms (-1)=w549, error in (no error)=w550) -> (element=w552:T7)  [unwired: 3 out]
            n226 = Less?(x=w542, y=-50.0) -> (x < y?=w540:bool)
            n227 = case shown="\"None\", Default" w552 {
              tunnel: [w562 State_Type_Definitions,_for_0.26g_versions_and_later_2."True Stop" ("Enum")] -> w544
              tunnel: w551 -> [w555 _]
              tunnel: w547 -> [w561 w578]
              tunnel: [w560 w579] -> w543
              tunnel: [State_Type_Definitions,_for_0.26g_versions_and_later_2."Idle" ("Enum") State_Type_Definitions,_for_0.26g_versions_and_later_2."Shutdown" ("Enum")] -> w545
              tunnel: w540 -> [w553 _]
              frame "None", Default {
                n228 = case shown="False" w553 {
                  tunnel: w561 -> [w565 w572]
                  tunnel: [w566 w571] -> w560
                  frame False {
                    n229 = for {
                      tunnel: string[] ["READ ENCODERS", "REVERSE", "READ NAVX"] ("element") -> [w567] mode=indexing
                      shift-right: [w569] -> w566
                      shift-left: w565 -> [w568]
                      n230 = Enqueue Element(queue=w568, element=w567) -> (queue out=w569:refnum<queue>)  [unwired: 2 in, 2 out]
                    }
                  }
                  frame True {
                    n231 = for {
                      shift-right: [w574] -> w571
                      shift-left: w572 -> [w575]
                      tunnel: string[] ["STOP", "ARDUINO - ULTRASONIC", "READ ULTRASONIC", "RESET ENCODERS"] -> [w573] mode=indexing
                      n232 = Enqueue Element(queue=w575, element=w573) -> (queue out=w574:refnum<queue>)  [unwired: 2 in, 2 out]
                    }
                  }
                }
                n233 = Or(x=w553, y=w555) -> (x .or. y?=w554:bool)
                n234 = Select(t=State_Type_Definitions,_for_0.26g_versions_and_later_2."True Stop" ("Enum"), s=w555, f=State_Type_Definitions,_for_0.26g_versions_and_later_2."Task 2:Sensor Mode" ("Enum")) -> (s? t:f=w556:T6)
                n235 = Select(t=w556, s=w554, f=State_Type_Definitions,_for_0.26g_versions_and_later_2."Task 2:Reverse Mode" ("Enum")) -> (s? t:f=w562:T6)
              }
              frame "Exit" {
                n236 = for {
                  shift-right: [w582] -> w579
                  shift-left: w578 -> [w583]
                  tunnel: string[] ["STOP", "RESET ENCODERS", "RESET YAW", "ARDUINO MODE 0"] -> [w581] mode=indexing
                  n237 = Enqueue Element(queue=w583, element=w581) -> (queue out=w582:refnum<queue>)  [unwired: 2 in, 2 out]
                }
              }
            }
          }
          frame 11 {
            # ">>> yStepper command>>>"
            n238 = Dequeue Element(queue=w598, timeout in ms (-1)=w597, error in (no error)=w596) -> (element=w587:T7)  [unwired: 3 out]
            n239 = Greater?(x=w595, y=160.0) -> (0:w592:bool)
            n240 = Or(x=w592, y=w593) -> (x .or. y?=w588:bool)
            n241 = case shown="\"None\", Default" w587 {
              tunnel: w588 -> [w601 _]
              tunnel: [w605 State_Type_Definitions,_for_0.26g_versions_and_later_2."True Stop" ("Enum")] -> w589
              tunnel: w591 -> [w602 w621]
              tunnel: [w600 w620] -> w590
              tunnel: [State_Type_Definitions,_for_0.26g_versions_and_later_2."Idle" ("Enum") State_Type_Definitions,_for_0.26g_versions_and_later_2."Shutdown" ("Enum")] -> w586
              frame "None", Default {
                n242 = case shown="False" w601 {
                  tunnel: w602 -> [w608 w614]
                  tunnel: [w607 w612] -> w600
                  frame False {
                    n243 = for {
                      shift-right: [w610] -> w607
                      shift-left: w608 -> [w611]
                      tunnel: string[] ["READ ENCODERS", "R-CW"] ("element") -> [w609] mode=indexing
                      n244 = Enqueue Element(queue=w611, element=w609) -> (queue out=w610:refnum<queue>)  [unwired: 2 in, 2 out]
                    }
                  }
                  frame True {
                    n245 = for {
                      shift-right: [w616] -> w612
                      shift-left: w614 -> [w617]
                      tunnel: string[] ["RESET YAW", "RESET ENCODERS", "STOP", "ARDUINO MODE 0"] -> [w615] mode=indexing
                      n246 = Enqueue Element(queue=w617, element=w615) -> (queue out=w616:refnum<queue>)  [unwired: 2 in, 2 out]
                    }
                  }
                }
                n247 = Select(t=State_Type_Definitions,_for_0.26g_versions_and_later_2."True Stop" ("Enum"), s=w601, f=State_Type_Definitions,_for_0.26g_versions_and_later_2."Task 3" ("Enum")) -> (s? t:f=w605:T6)
              }
              frame "Exit" {
                n248 = for {
                  shift-right: [w624] -> w620
                  shift-left: w621 -> [w625]
                  tunnel: string[] ["STOP", "RESET ENCODERS", "RESET YAW", ""] -> [w623] mode=indexing
                  n249 = Enqueue Element(queue=w625, element=w623) -> (queue out=w624:refnum<queue>)  [unwired: 2 in, 2 out]
                }
              }
            }
          }
          frame 12 {
            # ">> Stepper height reeached >>"
            # ">>> yStepper command>>>"
            # ">> Manual override >>"
            n250 = Dequeue Element(queue=w638, timeout in ms (-1)=w637, error in (no error)=w636) -> (element=w635:T7)  [unwired: 3 out]
            n251 = Equal?(x=w629, y=u8 60) -> (x = y?=w627:bool)
            n252 = case shown="\"Exit\"" w635 {
              tunnel: [w650 State_Type_Definitions,_for_0.26g_versions_and_later_2."True Stop" ("Enum")] -> w634
              tunnel: [w648 w666] -> w633
              tunnel: w639 -> [w647 w663]
              tunnel: w632 -> [w641 _]
              tunnel: [State_Type_Definitions,_for_0.26g_versions_and_later_2."Idle" ("Enum") State_Type_Definitions,_for_0.26g_versions_and_later_2."Shutdown" ("Enum")] -> w631
              tunnel: w627 -> [w640 _]
              frame "None", Default {
                # ">> WIill proceed to part ii if not manual override >>"
                # ">>If ENABLE or Trigger is set to true>>"
                n253 = Or(x=w640, y=w641) -> (x .or. y?=w642:bool)
                n254 = case shown="False" w640 {
                  tunnel: [w653 w659] -> w648
                  tunnel: w647 -> [w652 w658]
                  frame False {
                    n255 = for {
                      shift-right: [w655] -> w653
                      shift-left: w652 -> [w656]
                      tunnel: string[] ["Z STEPPER CAM HEIGHT", "READ STEPPER VALUES"] ("element") -> [w654] mode=indexing
                      n256 = Enqueue Element(queue=w656, element=w654) -> (queue out=w655:refnum<queue>)  [unwired: 2 in, 2 out]
                    }
                  }
                  frame True {
                    n257 = for {
                      shift-right: [w661] -> w659
                      shift-left: w658 -> [w662]
                      tunnel: string[] ["ARDUINO - ULTRASONIC", "READ ULTRASONIC", "FORWARD", "", "", ""] -> [w660] mode=indexing
                      n258 = Enqueue Element(queue=w662, element=w660) -> (queue out=w661:refnum<queue>)  [unwired: 2 in, 2 out]
                    }
                  }
                }
                n259 = Select(t=State_Type_Definitions,_for_0.26g_versions_and_later_2."True Stop" ("Enum"), s=w641, f=State_Type_Definitions,_for_0.26g_versions_and_later_2."Task 4_B" ("Enum")) -> (s? t:f=w644:T6)
                n260 = Select(t=w644, s=w642, f=State_Type_Definitions,_for_0.26g_versions_and_later_2."Task 4_A" ("Enum")) -> (s? t:f=w650:T6)
              }
              frame "Exit" {
                n261 = for {
                  shift-right: [w669] -> w666
                  shift-left: w663 -> [w670]
                  tunnel: string[] ["STOP", "RESET ENCODERS", "RESET YAW", ""] -> [w668] mode=indexing
                  n262 = Enqueue Element(queue=w670, element=w668) -> (queue out=w669:refnum<queue>)  [unwired: 2 in, 2 out]
                }
              }
            }
          }
          frame 13 {
            w675 = u8 20
            # ">> Path blocked >>"
            # ">>> yStepper command>>>"
            # ">> Manual override >>"
            n263 = Dequeue Element(queue=w684, timeout in ms (-1)=w683, error in (no error)=w682) -> (element=w681:T7)  [unwired: 3 out]
            n264 = Less?(x=w677, y=w675) -> (x < y?=w672:bool)
            n265 = Less?(x=w676, y=w675) -> (x < y?=w673:bool)
            n266 = And(x=w673, y=w672) -> (x .and. y?=w674:bool)
            n267 = case shown="\"None\", Default" w681 {
              tunnel: [w698 State_Type_Definitions,_for_0.26g_versions_and_later_2."True Stop" ("Enum")] -> w686
              tunnel: [w696 w713] -> w687
              tunnel: w680 -> [w695 _]
              tunnel: w685 -> [w689 _]
              tunnel: [State_Type_Definitions,_for_0.26g_versions_and_later_2."Idle" ("Enum") State_Type_Definitions,_for_0.26g_versions_and_later_2."Shutdown" ("Enum")] -> w679
              tunnel: w674 -> [w688 _]
              frame "None", Default {
                # ">> Manual override forces program to true stop >>"
                # ">>If ENABLE or Trigger is set to true>>"
                n268 = Or(x=w688, y=w689) -> (x .or. y?=w694:bool)
                n269 = case shown="True" w688 {
                  tunnel: [w701 w706] -> w696
                  tunnel: w695 -> [w700 w705]
                  frame False {
                    n270 = for {
                      shift-right: [w703] -> w701
                      shift-left: w700 -> [w704]
                      tunnel: string[] ["FORWARD", "READ ULTRASONIC", "READ NAVX"] ("element") -> [w702] mode=indexing
                      n271 = Enqueue Element(queue=w704, element=w702) -> (queue out=w703:refnum<queue>)  [unwired: 2 in, 2 out]
                    }
                  }
                  frame True {
                    n272 = for {
                      shift-right: [w709] -> w706
                      shift-left: w705 -> [w710]
                      tunnel: string[] ["STOP", "RESET YAW", "RESET ENCODERS", "RESET FLAGS"] -> [w708] mode=indexing
                      n273 = Enqueue Element(queue=w710, element=w708) -> (queue out=w709:refnum<queue>)  [unwired: 2 in, 2 out]
                    }
                  }
                }
                n274 = Select(t=State_Type_Definitions,_for_0.26g_versions_and_later_2."True Stop" ("Enum"), s=w689, f=State_Type_Definitions,_for_0.26g_versions_and_later_2."Task 4_C" ("Enum")) -> (s? t:f=w691:T6)
                n275 = Select(t=w691, s=w694, f=State_Type_Definitions,_for_0.26g_versions_and_later_2."Task 4_B" ("Enum")) -> (s? t:f=w698:T6)
              }
              frame "Exit" {
                n276 = for {
                  shift-right: [w716] -> w713
                  shift-left: _ -> [w717]
                  tunnel: string[] ["STOP", "RESET ENCODERS", "RESET YAW", ""] -> [w715] mode=indexing
                  n277 = Enqueue Element(queue=w717, element=w715) -> (queue out=w716:refnum<queue>)  [unwired: 2 in, 2 out]
                }
              }
            }
          }
          frame 14 {
            w728 = u8 20
            # ">> xDistance travelled>>"
            # ">> Path NOT blocked >>"
            # ">>> yStepper command>>>"
            # ">> Manual override >>"
            n278 = Dequeue Element(queue=w738, timeout in ms (-1)=w731, error in (no error)=w730) -> (element=w732:T7)  [unwired: 3 out]
            n279 = Greater?(x=w720, y=w728) -> (0:w726:bool)
            n280 = Greater?(x=w725, y=80.0) -> (0:w723:bool)
            n281 = Greater?(x=w719, y=w728) -> (0:w727:bool)
            n282 = And(x=w727, y=w726) -> (x .and. y?=w722:bool)
            n283 = And(x=w723, y=w722) -> (x .and. y?=w721:bool)
            n284 = case shown="\"Exit\"" w732 {
              tunnel: [w749 State_Type_Definitions,_for_0.26g_versions_and_later_2."True Stop" ("Enum")] -> w735
              tunnel: [w747 w765] -> w734
              tunnel: w737 -> [w746 w762]
              tunnel: w736 -> [w740 _]
              tunnel: [State_Type_Definitions,_for_0.26g_versions_and_later_2."Idle" ("t") State_Type_Definitions,_for_0.26g_versions_and_later_2."Shutdown" ("Enum")] -> w733
              tunnel: w721 -> [w739 _]
              frame "None", Default {
                # ">> Manual override forces program to true stop >>"
                # ">>If ENABLE or Trigger is set to true>>"
                n285 = Or(x=w739, y=w740) -> (x .or. y?=w745:bool)
                n286 = case shown="False" w739 {
                  tunnel: [w752 w757] -> w747
                  tunnel: w746 -> [w750 w756]
                  frame False {
                    n287 = for {
                      shift-right: [w754] -> w752
                      shift-left: w750 -> [w755]
                      tunnel: string[] ["RIGHT", "READ NAVX", "READ ENCODERS", "READ ULTRASONIC"] ("element") -> [w753] mode=indexing
                      n288 = Enqueue Element(queue=w755, element=w753) -> (queue out=w754:refnum<queue>)  [unwired: 2 in, 2 out]
                    }
                  }
                  frame True {
                    n289 = for {
                      shift-right: [w760] -> w757
                      shift-left: w756 -> [w761]
                      tunnel: string[] ["STOP", "RESET YAW", "RESET ENCODERS", "ARDUINO - ULTRASONIC"] -> [w759] mode=indexing
                      n290 = Enqueue Element(queue=w761, element=w759) -> (queue out=w760:refnum<queue>)  [unwired: 2 in, 2 out]
                    }
                  }
                }
                n291 = Select(t=State_Type_Definitions,_for_0.26g_versions_and_later_2."True Stop" ("Enum"), s=w740, f=State_Type_Definitions,_for_0.26g_versions_and_later_2."Task 4_D" ("Enum")) -> (s? t:f=w741:T6)
                n292 = Select(t=w741, s=w745, f=State_Type_Definitions,_for_0.26g_versions_and_later_2."Task 4_C" ("Enum")) -> (s? t:f=w749:T6)
              }
              frame "Exit" {
                n293 = for {
                  shift-right: [w768] -> w765
                  shift-left: w762 -> [w769]
                  tunnel: string[] ["STOP", "RESET ENCODERS", "RESET YAW", ""] -> [w767] mode=indexing
                  n294 = Enqueue Element(queue=w769, element=w767) -> (queue out=w768:refnum<queue>)  [unwired: 2 in, 2 out]
                }
              }
            }
          }
          frame 15 {
            w789 = u8 20
            # ">> yDistance travelled>>"
            # ">> Path blocked >>"
            # ">>> yStepper command>>>"
            # ">> Manual override >>"
            n295 = Dequeue Element(queue=w780, timeout in ms (-1)=w779, error in (no error)=w778) -> (element=w790:T7)  [unwired: 3 out]
            n296 = Less?(x=w773, y=w789) -> (x < y?=w787:bool)
            n297 = Greater?(x=w777, y=200.0) -> (0:w785:bool)
            n298 = Less?(x=w772, y=w789) -> (x < y?=w788:bool)
            n299 = And(x=w788, y=w787) -> (x .and. y?=w784:bool)
            n300 = Or(x=w785, y=w784) -> (x .or. y?=w783:bool)
            n301 = case shown="\"None\", Default" w790 {
              tunnel: [w801 State_Type_Definitions,_for_0.26g_versions_and_later_2."True Stop" ("Enum")] -> w776
              tunnel: [w799 w817] -> w774
              tunnel: w781 -> [w798 w814]
              tunnel: w782 -> [w792 _]
              tunnel: [State_Type_Definitions,_for_0.26g_versions_and_later_2."Idle" ("t") State_Type_Definitions,_for_0.26g_versions_and_later_2."Shutdown" ("Enum")] -> w775
              tunnel: w783 -> [w791 _]
              frame "None", Default {
                # ">> Manual override forces program to true stop >>"
                # ">>If ENABLE or Trigger is set to true>>"
                n302 = Or(x=w791, y=w792) -> (x .or. y?=w797:bool)
                n303 = case shown="True" w791 {
                  tunnel: [w804 w809] -> w799
                  tunnel: w798 -> [w802 w808]
                  frame False {
                    n304 = for {
                      shift-right: [w806] -> w804
                      shift-left: w802 -> [w807]
                      tunnel: string[] ["FORWARD", "READ NAVX", "READ ENCODERS", "READ ULTRASONIC"] ("element") -> [w805] mode=indexing
                      n305 = Enqueue Element(queue=w807, element=w805) -> (queue out=w806:refnum<queue>)  [unwired: 2 in, 2 out]
                    }
                  }
                  frame True {
                    n306 = for {
                      shift-right: [w812] -> w809
                      shift-left: w808 -> [w813]
                      tunnel: string[] ["STOP", "RESET YAW", "RESET ENCODERS", "RESET FLAGS"] -> [w811] mode=indexing
                      n307 = Enqueue Element(queue=w813, element=w811) -> (queue out=w812:refnum<queue>)  [unwired: 2 in, 2 out]
                    }
                  }
                }
                n308 = Select(t=State_Type_Definitions,_for_0.26g_versions_and_later_2."True Stop" ("Enum"), s=w792, f=State_Type_Definitions,_for_0.26g_versions_and_later_2."True Stop" ("Enum")) -> (s? t:f=w793:T6)
                n309 = Select(t=w793, s=w797, f=State_Type_Definitions,_for_0.26g_versions_and_later_2."Task 4_D" ("Enum")) -> (s? t:f=w801:T6)
              }
              frame "Exit" {
                n310 = for {
                  shift-right: [w820] -> w817
                  shift-left: w814 -> [w821]
                  tunnel: string[] ["STOP", "RESET ENCODERS", "RESET YAW", ""] -> [w819] mode=indexing
                  n311 = Enqueue Element(queue=w821, element=w819) -> (queue out=w820:refnum<queue>)  [unwired: 2 in, 2 out]
                }
              }
            }
          }
          frame 15 {
            # ">>> yStepper command>>>"
            # ">> Manual override >>"
            n312 = Dequeue Element(queue=w831, timeout in ms (-1)=w830, error in (no error)=w832) -> (element=w829:T7)  [unwired: 3 out]
            n313 = Equal?(x=w828, y=u8 60) -> (x = y?=w826:bool)
            n314 = case shown="\"None\", Default" w829 {
              tunnel: [w842 State_Type_Definitions,_for_0.26g_versions_and_later_2."True Stop" ("Enum")] -> w833
              tunnel: [w845 w862] -> w834
              tunnel: [State_Type_Definitions,_for_0.26g_versions_and_later_2."Idle" ("Enum") State_Type_Definitions,_for_0.26g_versions_and_later_2."Shutdown" ("Enum")] -> w835
              tunnel: w826 -> [w841 _]
              tunnel: w825 -> [w840 _]
              tunnel: w824 -> [w836 w859]
              frame "None", Default {
                # "Stays in Task 5_A until stepper reaches desired \nheight"
                # "T: Go back to idle, F: Continue with task\""
                # ">> Manual override >>"
                n315 = case shown="True" w841 {
                  tunnel: [w849 w855] -> w845
                  tunnel: w836 -> [w847 w853]
                  frame False {
                    n316 = for {
                      tunnel: string[] ["Z STEPPER CAM HEIGHT", "READ STEPPER VALUES"] ("element") -> [w850] mode=indexing
                      shift-right: [w852] -> w849
                      shift-left: w847 -> [w851]
                      n317 = Enqueue Element(queue=w851, element=w850) -> (queue out=w852:refnum<queue>)  [unwired: 2 in, 2 out]
                    }
                  }
                  frame True {
                    n318 = for {
                      shift-right: [w857] -> w855
                      shift-left: w853 -> [w858]
                      tunnel: string[] ["ARDUINO - ULTRASONIC", "READ ULTRASONIC", ""] -> [w856] mode=indexing
                      n319 = Enqueue Element(queue=w858, element=w856) -> (queue out=w857:refnum<queue>)  [unwired: 2 in, 2 out]
                    }
                  }
                }
                n320 = Or(x=w841, y=w840) -> (x .or. y?=w843:bool)
                n321 = Select(t=State_Type_Definitions,_for_0.26g_versions_and_later_2."True Stop" ("Enum"), s=w840, f=State_Type_Definitions."Task 5B: MOVE TO BOX" ("Enum")) -> (s? t:f=w837:u16)
                n322 = Select(t=w837, s=w843, f=State_Type_Definitions."Task 5A: ARM CAM HEIGHT" ("Enum")) -> (s? t:f=w842:u16)
              }
              frame "Exit" {
                n323 = for {
                  shift-right: [w865] -> w862
                  shift-left: w859 -> [w866]
                  tunnel: string[] ["STOP", "RESET ENCODERS", "RESET YAW", "ARDUINO MODE 0"] -> [w864] mode=indexing
                  n324 = Enqueue Element(queue=w866, element=w864) -> (queue out=w865:refnum<queue>)  [unwired: 2 in, 2 out]
                }
              }
            }
          }
          frame 16 {
            w873 = u8 20 ("y")
            # ">>> yStepper command>>>"
            n325 = Less?(x=w870, y=w873) -> (x < y?=w871:bool)
            n326 = Dequeue Element(queue=w877, timeout in ms (-1)=w876, error in (no error)=w878) -> (element=w875:T7)  [unwired: 3 out]
            n327 = Less?(x=w869, y=w873) -> (x < y?=w872:bool)
            n328 = And(x=w872, y=w871) -> (x .and. y?=w868:bool)
            n329 = case shown="\"None\", Default" w875 {
              tunnel: [w890 State_Type_Definitions,_for_0.26g_versions_and_later_2."True Stop" ("Enum")] -> w880
              tunnel: [w893 w910] -> w879
              tunnel: [State_Type_Definitions,_for_0.26g_versions_and_later_2."Idle" ("Enum") State_Type_Definitions,_for_0.26g_versions_and_later_2."Shutdown" ("Enum")] -> w881
              tunnel: w883 -> [w889 _]
              tunnel: w882 -> [w885 w907]
              tunnel: w868 -> [w884 _]
              frame "None", Default {
                # "Stays in Task 5_B to capture image over 5 seconds"
                # "T: Go back to idle, F: Continue with task\""
                # ">> Manual override >>"
                n330 = case shown="True" w884 {
                  tunnel: [w897 w903] -> w893
                  tunnel: w885 -> [w895 w901]
                  frame False {
                    n331 = for {
                      tunnel: string[] ["FORWARD", "READ ULTRASONIC", "READ NAVX"] ("element") -> [w898] mode=indexing
                      shift-right: [w900] -> w897
                      shift-left: w895 -> [w899]
                      n332 = Enqueue Element(queue=w899, element=w898) -> (queue out=w900:refnum<queue>)  [unwired: 2 in, 2 out]
                    }
                  }
                  frame True {
                    n333 = for {
                      shift-right: [w905] -> w903
                      shift-left: w901 -> [w906]
                      tunnel: string[] ["STOP", "RESET ENCODERS", "OPEN LOG CAM", "SET TIMER 5"] -> [w904] mode=indexing
                      n334 = Enqueue Element(queue=w906, element=w904) -> (queue out=w905:refnum<queue>)  [unwired: 2 in, 2 out]
                    }
                  }
                }
                n335 = Or(x=w884, y=w889) -> (x .or. y?=w891:bool)
                n336 = Select(t=State_Type_Definitions,_for_0.26g_versions_and_later_2."True Stop" ("Enum"), s=w889, f=State_Type_Definitions."Task 5C: CAM BURST" ("Enum")) -> (s? t:f=w886:u16)
                n337 = Select(t=w886, s=w891, f=State_Type_Definitions."Task 5B: MOVE TO BOX" ("Enum")) -> (s? t:f=w890:u16)
              }
              frame "Exit" {
                n338 = for {
                  shift-right: [w913] -> w910
                  shift-left: w907 -> [w914]
                  tunnel: string[] ["STOP", "RESET ENCODERS", "RESET YAW", "ARDUINO MODE 0"] -> [w912] mode=indexing
                  n339 = Enqueue Element(queue=w914, element=w912) -> (queue out=w913:refnum<queue>)  [unwired: 2 in, 2 out]
                }
              }
            }
          }
          frame 17 {
            # ">>> Motor control cluster >>>"
            # ">>> yStepper command>>>"
            # ">> Manual override >>"
            n340 = Dequeue Element(queue=w924, timeout in ms (-1)=w923, error in (no error)=w922) -> (element=w921:T7)  [unwired: 3 out]
            n341 = case shown="\"None\", Default" w921 {
              tunnel: [w933 State_Type_Definitions,_for_0.26g_versions_and_later_2."True Stop" ("Enum")] -> w926
              tunnel: [w936 w953] -> w919
              tunnel: [State_Type_Definitions,_for_0.26g_versions_and_later_2."Idle" ("Enum") State_Type_Definitions,_for_0.26g_versions_and_later_2."Shutdown" ("Enum")] -> w918
              tunnel: w920 -> [w927 _]
              tunnel: w925 -> [w932 w950]
              tunnel: w916 -> [w931 _]
              frame "None", Default {
                # ">> Is time up? >>"
                # "Determines if object is in range to pick up"
                # ">> Manual override >>"
                n342 = case shown="False" w931 {
                  tunnel: [w940 w946] -> w936
                  tunnel: w932 -> [w938 w944]
                  frame False {
                    n343 = for {
                      tunnel: string[] ["CAM ACQ", "START TIMER"] ("element") -> [w941] mode=indexing
                      shift-right: [w943] -> w940
                      shift-left: w938 -> [w942]
                      n344 = Enqueue Element(queue=w942, element=w941) -> (queue out=w943:refnum<queue>)  [unwired: 2 in, 2 out]
                    }
                  }
                  frame True {
                    n345 = for {
                      shift-right: [w948] -> w946
                      shift-left: w944 -> [w949]
                      tunnel: string[] ["CAM CLOSE", "PROCESS IMAGE", "SET TIMER 5"] -> [w947] mode=indexing
                      n346 = Enqueue Element(queue=w949, element=w947) -> (queue out=w948:refnum<queue>)  [unwired: 2 in, 2 out]
                    }
                  }
                }
                n347 = Or(x=w931, y=w927) -> (x .or. y?=w934:bool)
                n348 = Select(t=State_Type_Definitions,_for_0.26g_versions_and_later_2."True Stop" ("Enum"), s=w927, f=State_Type_Definitions."Task 5D: PROCESS IMAGE" ("Enum")) -> (s? t:f=w929:u16)
                n349 = Select(t=w929, s=w934, f=State_Type_Definitions."Task 5C: CAM BURST" ("Enum")) -> (s? t:f=w933:u16)
              }
              frame "Exit" {
                n350 = for {
                  shift-right: [w956] -> w953
                  shift-left: w950 -> [w957]
                  tunnel: string[] ["STOP", "RESET ENCODERS", "RESET YAW", "ARDUINO MODE 0"] -> [w955] mode=indexing
                  n351 = Enqueue Element(queue=w957, element=w955) -> (queue out=w956:refnum<queue>)  [unwired: 2 in, 2 out]
                }
              }
            }
          }
          frame 18 {
            # ">>> yStepper command>>>"
            n352 = Dequeue Element(queue=w964, timeout in ms (-1)=w963, error in (no error)=w962) -> (element=w961:T7)  [unwired: 3 out]
            n353 = case shown="\"None\", Default" w961 {
              tunnel: [w976 State_Type_Definitions,_for_0.26g_versions_and_later_2."True Stop" ("Enum")] -> w968
              tunnel: [w979 w996] -> w967
              tunnel: [State_Type_Definitions,_for_0.26g_versions_and_later_2."Idle" ("Enum") State_Type_Definitions,_for_0.26g_versions_and_later_2."Shutdown" ("Enum")] -> w969
              tunnel: w965 -> [w975 _]
              tunnel: w966 -> [w971 w993]
              tunnel: w959 -> [w970 _]
              frame "None", Default {
                # ">> T: Breaks out of state loop; F: Stays in loop>>"
                # ">> Manual override >>"
                # ">> Checks if time is up>>"
                # "Stays in Task 5D until the object is detected"
                # "T: Go back to idle, F: Continue with task\""
                # ">> Manual override >>"
                n354 = case shown="True" w970 {
                  tunnel: [w983 w989] -> w979
                  tunnel: w971 -> [w981 w987]
                  frame False {
                    n355 = for {
                      tunnel: string[] ["START TIMER", "PROCESS IMAGE", ""] ("element") -> [w984] mode=indexing
                      shift-right: [w986] -> w983
                      shift-left: w981 -> [w985]
                      n356 = Enqueue Element(queue=w985, element=w984) -> (queue out=w986:refnum<queue>)  [unwired: 2 in, 2 out]
                    }
                  }
                  frame True {
                    n357 = for {
                      shift-right: [w991] -> w989
                      shift-left: w987 -> [w992]
                      tunnel: string[] ["CAM CLOSE", "", ""] -> [w990] mode=indexing
                      n358 = Enqueue Element(queue=w992, element=w990) -> (queue out=w991:refnum<queue>)  [unwired: 2 in, 2 out]
                    }
                  }
                }
                n359 = Or(x=w970, y=w975) -> (x .or. y?=w977:bool)
                n360 = Select(t=State_Type_Definitions,_for_0.26g_versions_and_later_2."True Stop" ("Enum"), s=w975, f=State_Type_Definitions,_for_0.26g_versions_and_later_2."Task 5E: POSITION ARM" ("Enum")) -> (s? t:f=w972:T6)
                n361 = Select(t=w972, s=w977, f=State_Type_Definitions."Task 5D: PROCESS IMAGE" ("Enum")) -> (s? t:f=w976:u16)
              }
              frame "Exit" {
                n362 = for {
                  shift-right: [w999] -> w996
                  shift-left: w993 -> [w1000]
                  tunnel: string[] ["STOP", "RESET ENCODERS", "RESET YAW", "ARDUINO MODE 0"] -> [w998] mode=indexing
                  n363 = Enqueue Element(queue=w1000, element=w998) -> (queue out=w999:refnum<queue>)  [unwired: 2 in, 2 out]
                }
              }
            }
          }
          frame 20 {
            # ">>> yStepper command>>>"
            n364 = Dequeue Element(queue=w1013, timeout in ms (-1)=w1014, error in (no error)=w1015) -> (element=w1017:T7)  [unwired: 3 out]
            n365 = formula code="if (pos < 100)\ny = 41;\n\nelse if (pos >= 100 && pos <= 140)\ny = 30;\n\nelse if (pos >= 141 && pos <= 170)\ny = 25;\n\nelse if (pos >= 171 &&pos <= 180) \ny = 20;\n\nelse if (pos >= 181&& pos <= 200)\ny = 15;\n\nelse if (pos >= 201 && pos <= 230)\ny = 10;\n\nelse if (pos >= 231 && pos <= 320)\ny = 8;\n\nelse if (pos > 320)\ny = 0;"("pos"=w1005) -> ("y"=w1008:dbl)
            n366 = To Unsigned Byte Integer(number=w1008) -> (unsigned 8bit integer=w1003:u8)
            n367 = Equal?(x=w1004, y=w1003) -> (x = y?=w1002:bool)
            n368 = case shown="\"None\", Default" w1017 {
              tunnel: [w1024 State_Type_Definitions,_for_0.26g_versions_and_later_2."True Stop" ("Enum")] -> w1011
              tunnel: [w1027 w1044] -> w1009
              tunnel: [State_Type_Definitions,_for_0.26g_versions_and_later_2."Idle" ("Enum") State_Type_Definitions,_for_0.26g_versions_and_later_2."Shutdown" ("Enum")] -> w1010
              tunnel: w1016 -> [w1023 _]
              tunnel: w1012 -> [w1019 w1041]
              tunnel: w1002 -> [w1018 _]
              frame "None", Default {
                # ">> T: Breaks out of state loop; F: Stays in loop>>"
                # ">> Manual override >>"
                # ">> Checks if time is up>>"
                # "Stays in Task 5D until the object is detected"
                # "T: Go back to idle, F: Continue with task\""
                # ">> Manual override >>"
                n369 = case shown="False" w1018 {
                  tunnel: [w1031 w1037] -> w1027
                  tunnel: w1019 -> [w1029 w1035]
                  frame False {
                    n370 = for {
                      tunnel: string[] ["READ STEPPER VALUES", "Y STEPPER CONTROL", ""] ("element") -> [w1032] mode=indexing
                      shift-right: [w1034] -> w1031
                      shift-left: w1029 -> [w1033]
                      n371 = Enqueue Element(queue=w1033, element=w1032) -> (queue out=w1034:refnum<queue>)  [unwired: 2 in, 2 out]
                    }
                  }
                  frame True {
                    n372 = for {
                      shift-right: [w1039] -> w1037
                      shift-left: w1035 -> [w1040]
                      tunnel: string[] ["CAM CLOSE", "DISPOSE BUFFERS", ""] -> [w1038] mode=indexing
                      n373 = Enqueue Element(queue=w1040, element=w1038) -> (queue out=w1039:refnum<queue>)  [unwired: 2 in, 2 out]
                    }
                  }
                }
                n374 = Or(x=w1018, y=w1023) -> (x .or. y?=w1025:bool)
                n375 = Select(t=State_Type_Definitions,_for_0.26g_versions_and_later_2."True Stop" ("Enum"), s=w1023, f=State_Type_Definitions,_for_0.26g_versions_and_later_2."Task 5F: ARM GRAB HEIGHT" ("Enum")) -> (s? t:f=w1020:T6)
                n376 = Select(t=w1020, s=w1025, f=State_Type_Definitions,_for_0.26g_versions_and_later_2."Task 5E: POSITION ARM" ("Enum")) -> (s? t:f=w1024:T6)
              }
              frame "Exit" {
                n377 = for {
                  shift-right: [w1047] -> w1044
                  shift-left: w1041 -> [w1048]
                  tunnel: string[] ["STOP", "RESET ENCODERS", "RESET YAW", "ARDUINO MODE 0"] -> [w1046] mode=indexing
                  n378 = Enqueue Element(queue=w1048, element=w1046) -> (queue out=w1047:refnum<queue>)  [unwired: 2 in, 2 out]
                }
              }
            }
            n379 = Bundle By Name(cluster=w1007, "yStepper desired"=w1003) -> (w1006:T10)
          }
          frame 21 {
            # ">>> Motor control cluster >>>"
            # ">>> yStepper command>>>"
            # ">> Manual override >>"
            n380 = Dequeue Element(queue=w1058, timeout in ms (-1)=w1057, error in (no error)=w1059) -> (element=w1056:T7)  [unwired: 3 out]
            n381 = Equal?(x=w1055, y=u8 1) -> (x = y?=w1053:bool)
            n382 = case shown="\"None\", Default" w1056 {
              tunnel: [w1069 State_Type_Definitions,_for_0.26g_versions_and_later_2."True Stop" ("Enum")] -> w1060
              tunnel: [w1072 w1089] -> w1061
              tunnel: [State_Type_Definitions,_for_0.26g_versions_and_later_2."Idle" ("Enum") State_Type_Definitions,_for_0.26g_versions_and_later_2."Shutdown" ("Enum")] -> w1062
              tunnel: w1053 -> [w1068 _]
              tunnel: w1052 -> [w1067 _]
              tunnel: w1051 -> [w1063 w1086]
              frame "None", Default {
                # "Stays in Task 5F until stepper reaches desired \nheight"
                # "T: Go back to idle, F: Continue with task\""
                # ">> Manual override >>"
                n383 = case shown="True" w1068 {
                  tunnel: [w1076 w1082] -> w1072
                  tunnel: w1063 -> [w1074 w1080]
                  frame False {
                    n384 = for {
                      tunnel: string[] ["Z STEPPER GRAB HEIGHT", "READ STEPPER VALUES"] ("element") -> [w1077] mode=indexing
                      shift-right: [w1079] -> w1076
                      shift-left: w1074 -> [w1078]
                      n385 = Enqueue Element(queue=w1078, element=w1077) -> (queue out=w1079:refnum<queue>)  [unwired: 2 in, 2 out]
                    }
                  }
                  frame True {
                    n386 = for {
                      shift-right: [w1084] -> w1082
                      shift-left: w1080 -> [w1085]
                      tunnel: string[] ["SET TIMER 5", "CLOSE CLAW", ""] -> [w1083] mode=indexing
                      n387 = Enqueue Element(queue=w1085, element=w1083) -> (queue out=w1084:refnum<queue>)  [unwired: 2 in, 2 out]
                    }
                  }
                }
                n388 = Or(x=w1068, y=w1067) -> (x .or. y?=w1070:bool)
                n389 = Select(t=State_Type_Definitions,_for_0.26g_versions_and_later_2."True Stop" ("Enum"), s=w1067, f=State_Type_Definitions,_for_0.26g_versions_and_later_2."Task 5G: CLOSE CLAW" ("Enum")) -> (s? t:f=w1064:T6)
                n390 = Select(t=w1064, s=w1070, f=State_Type_Definitions,_for_0.26g_versions_and_later_2."Task 5F: ARM GRAB HEIGHT" ("Enum")) -> (s? t:f=w1069:T6)
              }
              frame "Exit" {
                n391 = for {
                  shift-right: [w1092] -> w1089
                  shift-left: w1086 -> [w1093]
                  tunnel: string[] ["STOP", "RESET ENCODERS", "RESET YAW", "ARDUINO MODE 0"] -> [w1091] mode=indexing
                  n392 = Enqueue Element(queue=w1093, element=w1091) -> (queue out=w1092:refnum<queue>)  [unwired: 2 in, 2 out]
                }
              }
            }
          }
          frame 22 {
            # ">>> yStepper command>>>"
            # ">> Manual override >>"
            n393 = Dequeue Element(queue=w1103, timeout in ms (-1)=w1102, error in (no error)=w1101) -> (element=w1100:T7)  [unwired: 3 out]
            n394 = case shown="\"None\", Default" w1100 {
              tunnel: [w1112 State_Type_Definitions,_for_0.26g_versions_and_later_2."True Stop" ("Enum")] -> w1105
              tunnel: [w1115 w1132] -> w1098
              tunnel: [State_Type_Definitions,_for_0.26g_versions_and_later_2."Idle" ("Enum") State_Type_Definitions,_for_0.26g_versions_and_later_2."Shutdown" ("Enum")] -> w1097
              tunnel: w1099 -> [w1106 _]
              tunnel: w1104 -> [w1111 w1129]
              tunnel: w1095 -> [w1110 _]
              frame "None", Default {
                # ">> Is time up? >>"
                # "Determines if object is in range to pick up"
                # ">> Manual override >>"
                n395 = case shown="True" w1110 {
                  tunnel: [w1119 w1125] -> w1115
                  tunnel: w1111 -> [w1117 w1123]
                  frame False {
                    n396 = for {
                      tunnel: string[] ["CLOSE CLAW", "START TIMER"] ("element") -> [w1120] mode=indexing
                      shift-right: [w1122] -> w1119
                      shift-left: w1117 -> [w1121]
                      n397 = Enqueue Element(queue=w1121, element=w1120) -> (queue out=w1122:refnum<queue>)  [unwired: 2 in, 2 out]
                    }
                  }
                  frame True {
                    n398 = for {
                      shift-right: [w1127] -> w1125
                      shift-left: w1123 -> [w1128]
                      tunnel: string[] ["READ STEPPER VALUES", "", ""] -> [w1126] mode=indexing
                      n399 = Enqueue Element(queue=w1128, element=w1126) -> (queue out=w1127:refnum<queue>)  [unwired: 2 in, 2 out]
                    }
                  }
                }
                n400 = Or(x=w1110, y=w1106) -> (x .or. y?=w1113:bool)
                n401 = Select(t=State_Type_Definitions,_for_0.26g_versions_and_later_2."True Stop" ("Enum"), s=w1106, f=State_Type_Definitions,_for_0.26g_versions_and_later_2."Task 5H: RAISE ARM" ("Enum")) -> (s? t:f=w1108:T6)
                n402 = Select(t=w1108, s=w1113, f=State_Type_Definitions,_for_0.26g_versions_and_later_2."Task 5G: CLOSE CLAW" ("Enum")) -> (s? t:f=w1112:T6)
              }
              frame "Exit" {
                n403 = for {
                  shift-right: [w1135] -> w1132
                  shift-left: w1129 -> [w1136]
                  tunnel: string[] ["STOP", "RESET ENCODERS", "RESET YAW", "ARDUINO MODE 0"] -> [w1134] mode=indexing
                  n404 = Enqueue Element(queue=w1136, element=w1134) -> (queue out=w1135:refnum<queue>)  [unwired: 2 in, 2 out]
                }
              }
            }
          }
          frame 23 {
            # ">>> yStepper command>>>"
            # ">> Manual override >>"
            n405 = Dequeue Element(queue=w1146, timeout in ms (-1)=w1145, error in (no error)=w1147) -> (element=w1144:T7)  [unwired: 3 out]
            n406 = Equal?(x=w1143, y=u8 60) -> (x = y?=w1141:bool)
            n407 = case shown="\"None\", Default" w1144 {
              tunnel: [w1157 State_Type_Definitions,_for_0.26g_versions_and_later_2."True Stop" ("Enum")] -> w1148
              tunnel: [w1160 w1177] -> w1149
              tunnel: [State_Type_Definitions,_for_0.26g_versions_and_later_2."Idle" ("Enum") State_Type_Definitions,_for_0.26g_versions_and_later_2."Shutdown" ("Enum")] -> w1150
              tunnel: w1141 -> [w1156 _]
              tunnel: w1140 -> [w1155 _]
              tunnel: w1139 -> [w1151 w1174]
              frame "None", Default {
                # "Stays in Task 5_A until stepper reaches desired \nheight"
                # "T: Go back to idle, F: Continue with task\""
                # ">> Manual override >>"
                n408 = case shown="False" w1156 {
                  tunnel: [w1164 w1170] -> w1160
                  tunnel: w1151 -> [w1162 w1168]
                  frame False {
                    n409 = for {
                      tunnel: string[] ["Z STEPPER CAM HEIGHT", "READ STEPPER VALUES"] ("element") -> [w1165] mode=indexing
                      shift-right: [w1167] -> w1164
                      shift-left: w1162 -> [w1166]
                      n410 = Enqueue Element(queue=w1166, element=w1165) -> (queue out=w1167:refnum<queue>)  [unwired: 2 in, 2 out]
                    }
                  }
                  frame True {
                    n411 = for {
                      shift-right: [w1172] -> w1170
                      shift-left: w1168 -> [w1173]
                      tunnel: string[] ["ARDUINO - ULTRASONIC", "READ ULTRASONIC", ""] -> [w1171] mode=indexing
                      n412 = Enqueue Element(queue=w1173, element=w1171) -> (queue out=w1172:refnum<queue>)  [unwired: 2 in, 2 out]
                    }
                  }
                }
                n413 = Or(x=w1156, y=w1155) -> (x .or. y?=w1158:bool)
                n414 = Select(t=State_Type_Definitions,_for_0.26g_versions_and_later_2."True Stop" ("Enum"), s=w1155, f=State_Type_Definitions,_for_0.26g_versions_and_later_2."True Stop" ("Enum")) -> (s? t:f=w1152:T6)
                n415 = Select(t=w1152, s=w1158, f=State_Type_Definitions,_for_0.26g_versions_and_later_2."Task 5H: RAISE ARM" ("Enum")) -> (s? t:f=w1157:T6)
              }
              frame "Exit" {
                n416 = for {
                  shift-right: [w1180] -> w1177
                  shift-left: w1174 -> [w1181]
                  tunnel: string[] ["STOP", "RESET ENCODERS", "RESET YAW", "ARDUINO MODE 0"] -> [w1179] mode=indexing
                  n417 = Enqueue Element(queue=w1181, element=w1179) -> (queue out=w1180:refnum<queue>)  [unwired: 2 in, 2 out]
                }
              }
            }
          }
          frame 24 {
            # ">>> yStepper command>>>"
            n418 = Dequeue Element(queue=w1190, timeout in ms (-1)=w1189, error in (no error)=w1188) -> (element=w1195:T7)  [unwired: 3 out]
            n419 = Equal?(x=w1186, y=u8 60) -> (x = y?=w1185:bool)
            n420 = case shown="\"None\", Default" w1195 {
              tunnel: [w1202 State_Type_Definitions,_for_0.26g_versions_and_later_2."True Stop" ("Enum")] -> w1193
              tunnel: [w1201 w1219] -> w1192
              tunnel: [State_Type_Definitions,_for_0.26g_versions_and_later_2."Idle" ("Enum") State_Type_Definitions,_for_0.26g_versions_and_later_2."Shutdown" ("Enum")] -> w1194
              tunnel: w1191 -> [w1197 _]
              tunnel: w1187 -> [w1199 _]
              tunnel: w1185 -> [w1196 _]
              frame "None", Default {
                n421 = case shown="False" w1196 {
                  tunnel: [w1207 w1213] -> w1201
                  tunnel: w1199 -> [w1205 w1211]
                  frame False {
                    n422 = for {
                      tunnel: string[] ["Z STEPPER CAM HEIGHT", "READ STEPPER VALUES"] ("element") -> [w1208] mode=indexing
                      shift-right: [w1210] -> w1207
                      shift-left: w1205 -> [w1209]
                      n423 = Enqueue Element(queue=w1209, element=w1208) -> (queue out=w1210:refnum<queue>)  [unwired: 2 in, 2 out]
                    }
                  }
                  frame True {
                    n424 = for {
                      shift-right: [w1215] -> w1213
                      shift-left: w1211 -> [w1216]
                      tunnel: string[] ["CAM ACQ", "OPEN LOG CAM"] -> [w1214] mode=indexing
                      n425 = Enqueue Element(queue=w1216, element=w1214) -> (queue out=w1215:refnum<queue>)  [unwired: 2 in, 2 out]
                    }
                  }
                }
                n426 = Or(x=w1196, y=w1197) -> (x .or. y?=w1198:bool)
                n427 = Select(t=State_Type_Definitions,_for_0.26g_versions_and_later_2."Task 6_B" ("Enum"), s=w1198, f=State_Type_Definitions,_for_0.26g_versions_and_later_2."Task 6_A" ("Enum")) -> (s? t:f=w1202:T6)
              }
              frame "Exit" {
                n428 = for {
                  shift-right: [w1222] -> w1219
                  shift-left: _ -> [w1223]
                  tunnel: string[] ["STOP", "RESET ENCODERS", "RESET YAW", "ARDUINO MODE 0"] -> [w1221] mode=indexing
                  n429 = Enqueue Element(queue=w1223, element=w1221) -> (queue out=w1222:refnum<queue>)  [unwired: 2 in, 2 out]
                }
              }
            }
          }
          frame 25 {
            # ">>> yStepper command>>>"
            n430 = Dequeue Element(queue=w1234, timeout in ms (-1)=w1232, error in (no error)=w1233) -> (element=w1231:T7)  [unwired: 3 out]
            n431 = case shown="\"None\", Default" w1231 {
              tunnel: [w1241 State_Type_Definitions,_for_0.26g_versions_and_later_2."True Stop" ("Enum")] -> w1227
              tunnel: [w1240 w1259] -> w1235
              tunnel: [State_Type_Definitions,_for_0.26g_versions_and_later_2."Idle" ("Enum") State_Type_Definitions,_for_0.26g_versions_and_later_2."Shutdown" ("Enum")] -> w1228
              tunnel: w1230 -> [w1236 _]
              tunnel: w1229 -> [w1238 _]
              tunnel: w1226 -> [w1237 w1256]
              frame "None", Default {
                # ">> Manual override >>"
                n432 = case shown="True" w1238 {
                  tunnel: [w1246 w1252] -> w1240
                  tunnel: w1237 -> [w1245 w1250]
                  frame False {
                    n433 = for {
                      shift-right: [w1249] -> w1246
                      shift-left: w1245 -> [w1248]
                      tunnel: string[] ["CAM ACQ", "PROCESS IMAGE", "OPEN CLAW"] -> [w1247] mode=indexing
                      n434 = Enqueue Element(queue=w1248, element=w1247) -> (queue out=w1249:refnum<queue>)  [unwired: 2 in, 2 out]
                    }
                  }
                  frame True {
                    n435 = for {
                      shift-right: [w1254] -> w1252
                      shift-left: w1250 -> [w1255]
                      tunnel: string[] ["CAM ACQ", "PROCESS IMAGE", "CLOSE CLAW"] -> [w1253] mode=indexing
                      n436 = Enqueue Element(queue=w1255, element=w1253) -> (queue out=w1254:refnum<queue>)  [unwired: 2 in, 2 out]
                    }
                  }
                }
                n437 = Select(t=State_Type_Definitions,_for_0.26g_versions_and_later_2."True Stop" ("Enum"), s=w1236, f=State_Type_Definitions,_for_0.26g_versions_and_later_2."Task 6_B" ("Enum")) -> (s? t:f=w1241:T6)
              }
              frame "Exit" {
                # ">> State after true stop >>"
                # ">> Goes to true stop >>"
                n438 = for {
                  shift-right: [w1262] -> w1259
                  shift-left: w1256 -> [w1263]
                  tunnel: string[] ["STOP", "RESET ENCODERS", "RESET YAW", ""] -> [w1261] mode=indexing
                  n439 = Enqueue Element(queue=w1263, element=w1261) -> (queue out=w1262:refnum<queue>)  [unwired: 2 in, 2 out]
                }
              }
            }
          }
          frame 26 {
          }
          frame 38 {
            # ">> Stepper height reeached >>"
            # ">>> yStepper command>>>"
            # ">> Manual override >>"
            n440 = Dequeue Element(queue=w1279, timeout in ms (-1)=w1274, error in (no error)=w1278) -> (element=w1282:T7)  [unwired: 3 out]
            n441 = Equal?(x=w1276, y=u8 60) -> (x = y?=w1280:bool)
            n442 = case shown="\"None\", Default" w1282 {
              tunnel: [w1293 State_Type_Definitions,_for_0.26g_versions_and_later_2."True Stop" ("Enum")] -> w1272
              tunnel: [w1291 w1308] -> w1271
              tunnel: w1275 -> [w1290 _]
              tunnel: w1277 -> [w1284 _]
              tunnel: [State_Type_Definitions,_for_0.26g_versions_and_later_2."Idle" ("Enum") State_Type_Definitions,_for_0.26g_versions_and_later_2."Shutdown" ("Enum")] -> w1273
              tunnel: w1280 -> [w1283 _]
              frame "None", Default {
                # ">> WIill proceed to part ii if not manual override >>"
                # ">>If ENABLE or Trigger is set to true>>"
                n443 = Or(x=w1283, y=w1284) -> (x .or. y?=w1285:bool)
                n444 = case shown="True" w1283 {
                  tunnel: [w1296 w1302] -> w1291
                  tunnel: w1290 -> [w1295 w1301]
                  frame False {
                    n445 = for {
                      shift-right: [w1298] -> w1296
                      shift-left: w1295 -> [w1299]
                      tunnel: string[] ["Z STEPPER CAM HEIGHT", "READ STEPPER VALUES"] ("element") -> [w1297] mode=indexing
                      n446 = Enqueue Element(queue=w1299, element=w1297) -> (queue out=w1298:refnum<queue>)  [unwired: 2 in, 2 out]
                    }
                  }
                  frame True {
                    n447 = for {
                      shift-right: [w1304] -> w1302
                      shift-left: w1301 -> [w1305]
                      tunnel: string[] ["ARDUINO - ULTRASONIC", "READ ULTRASONIC", "", "", "", ""] -> [w1303] mode=indexing
                      n448 = Enqueue Element(queue=w1305, element=w1303) -> (queue out=w1304:refnum<queue>)  [unwired: 2 in, 2 out]
                    }
                  }
                }
                n449 = Select(t=State_Type_Definitions,_for_0.26g_versions_and_later_2."True Stop" ("Enum"), s=w1284, f=State_Type_Definitions,_for_0.26g_versions_and_later_2."Task 9B: Rotate to Angle" ("Enum")) -> (s? t:f=w1287:T6)
                n450 = Select(t=w1287, s=w1285, f=State_Type_Definitions,_for_0.26g_versions_and_later_2."Task 9A: Raise Arm" ("Enum")) -> (s? t:f=w1293:T6)
              }
              frame "Exit" {
                n451 = for {
                  shift-right: [w1311] -> w1308
                  shift-left: _ -> [w1312]
                  tunnel: string[] ["STOP", "RESET ENCODERS", "RESET YAW", ""] -> [w1310] mode=indexing
                  n452 = Enqueue Element(queue=w1312, element=w1310) -> (queue out=w1311:refnum<queue>)  [unwired: 2 in, 2 out]
                }
              }
            }
          }
          frame 39 {
            # ">>> yStepper command>>>"
            n453 = Dequeue Element(queue=w1325, timeout in ms (-1)=w1324, error in (no error)=w1323) -> (element=w1327:T7)  [unwired: 3 out]
            n454 = In Range and Coerce(upper limit=305.0, x=w1317, lower limit=295.0) -> (In Range?=w1314:bool)  [unwired: 1 out]
            n455 = case shown="\"None\", Default" w1327 {
              tunnel: w1318 -> [w1330 _]
              tunnel: [w1338 State_Type_Definitions,_for_0.26g_versions_and_later_2."True Stop" ("Enum")] -> w1320
              tunnel: w1326 -> [w1336 w1354]
              tunnel: [w1335 w1353] -> w1319
              tunnel: [State_Type_Definitions,_for_0.26g_versions_and_later_2."Idle" ("Enum") State_Type_Definitions,_for_0.26g_versions_and_later_2."Shutdown" ("Enum")] -> w1321
              tunnel: w1314 -> [w1328 _]
              frame "None", Default {
                n456 = Or(x=w1328, y=w1330) -> (x .or. y?=w1329:bool)
                n457 = case shown="True" w1328 {
                  tunnel: w1336 -> [w1341 w1347]
                  tunnel: [w1340 w1345] -> w1335
                  frame False {
                    n458 = for {
                      shift-right: [w1343] -> w1340
                      shift-left: w1341 -> [w1344]
                      tunnel: string[] ["READ NAVX", "R-ACW"] ("element") -> [w1342] mode=indexing
                      n459 = Enqueue Element(queue=w1344, element=w1342) -> (queue out=w1343:refnum<queue>)  [unwired: 2 in, 2 out]
                    }
                  }
                  frame True {
                    n460 = for {
                      shift-right: [w1349] -> w1345
                      shift-left: w1347 -> [w1350]
                      tunnel: string[] ["STOP", "RESET ENCODERS", "RESET YAW", ""] -> [w1348] mode=indexing
                      n461 = Enqueue Element(queue=w1350, element=w1348) -> (queue out=w1349:refnum<queue>)  [unwired: 2 in, 2 out]
                    }
                  }
                }
                n462 = Select(t=State_Type_Definitions,_for_0.26g_versions_and_later_2."True Stop" ("Enum"), s=w1330, f=State_Type_Definitions."Task 9C: Rotation alignmnet") -> (s? t:f=w1332:u16)
                n463 = Select(t=w1332, s=w1329, f=State_Type_Definitions,_for_0.26g_versions_and_later_2."Task 9B: Rotate to Angle" ("Enum")) -> (s? t:f=w1338:u16)
              }
              frame "Exit" {
                n464 = for {
                  shift-right: [w1357] -> w1353
                  shift-left: w1354 -> [w1358]
                  tunnel: string[] ["STOP", "RESET ENCODERS", "RESET YAW", ""] -> [w1356] mode=indexing
                  n465 = Enqueue Element(queue=w1358, element=w1356) -> (queue out=w1357:refnum<queue>)  [unwired: 2 in, 2 out]
                }
              }
            }
          }
          frame 39 {
            # ">>> yStepper command>>>"
            n466 = Dequeue Element(queue=w1368, timeout in ms (-1)=w1367, error in (no error)=w1366) -> (element=w1369:T7)  [unwired: 3 out]
            n467 = case shown="\"None\", Default" w1369 {
              tunnel: w1364 -> [w1370 _]
              tunnel: [w1378 State_Type_Definitions,_for_0.26g_versions_and_later_2."True Stop" ("Enum")] -> w1361
              tunnel: w1365 -> [w1376 w1394]
              tunnel: [w1375 w1393] -> w1360
              tunnel: [State_Type_Definitions,_for_0.26g_versions_and_later_2."Idle" ("Enum") State_Type_Definitions,_for_0.26g_versions_and_later_2."Shutdown" ("Enum")] -> w1363
              frame "None", Default {
                n468 = case shown="True" w1370 {
                  tunnel: w1376 -> [w1381 w1387]
                  tunnel: [w1380 w1385] -> w1375
                  frame False {
                    n469 = for {
                      shift-right: [w1383] -> w1380
                      shift-left: w1381 -> [w1384]
                      tunnel: string[] ["READ IR", "FORWARD - IR ASSIST"] ("element") -> [w1382] mode=indexing
                      n470 = Enqueue Element(queue=w1384, element=w1382) -> (queue out=w1383:refnum<queue>)  [unwired: 2 in, 2 out]
                    }
                  }
                  frame True {
                    n471 = for {
                      shift-right: [w1389] -> w1385
                      shift-left: w1387 -> [w1390]
                      tunnel: string[] ["STOP", "RESET ENCODERS", "RESET YAW", ""] -> [w1388] mode=indexing
                      n472 = Enqueue Element(queue=w1390, element=w1388) -> (queue out=w1389:refnum<queue>)  [unwired: 2 in, 2 out]
                    }
                  }
                }
                n473 = Select(t=State_Type_Definitions,_for_0.26g_versions_and_later_2."True Stop" ("Enum"), s=w1370, f=State_Type_Definitions,_for_0.26g_versions_and_later_2."True Stop") -> (s? t:f=w1372:T6)
                n474 = Select(t=w1372, s=w1370, f=State_Type_Definitions."Task 9C: Rotation alignmnet" ("Enum")) -> (s? t:f=w1378:u16)
              }
              frame "Exit" {
                n475 = for {
                  shift-right: [w1397] -> w1393
                  shift-left: w1394 -> [w1398]
                  tunnel: string[] ["STOP", "RESET ENCODERS", "RESET YAW", ""] -> [w1396] mode=indexing
                  n476 = Enqueue Element(queue=w1398, element=w1396) -> (queue out=w1397:refnum<queue>)  [unwired: 2 in, 2 out]
                }
              }
            }
          }
          frame 27 {
            # ">>> yStepper command>>>"
            # ">> Manual override >>"
            n477 = Dequeue Element(queue=w1408, timeout in ms (-1)=w1407, error in (no error)=w1409) -> (element=w1406:T7)  [unwired: 3 out]
            n478 = Equal?(x=w1405, y=u8 60) -> (x = y?=w1403:bool)
            n479 = case shown="\"None\", Default" w1406 {
              tunnel: [w1419 State_Type_Definitions,_for_0.26g_versions_and_later_2."True Stop" ("Enum")] -> w1410
              tunnel: [w1422 w1439] -> w1411
              tunnel: [State_Type_Definitions,_for_0.26g_versions_and_later_2."Idle" ("Enum") State_Type_Definitions,_for_0.26g_versions_and_later_2."Shutdown" ("Enum")] -> w1412
              tunnel: w1403 -> [w1418 _]
              tunnel: w1402 -> [w1417 _]
              tunnel: w1401 -> [w1413 w1436]
              frame "None", Default {
                # "Stays in Task 5_A until stepper reaches desired \nheight"
                # "T: Go back to idle, F: Continue with task\""
                # ">> Manual override >>"
                n480 = case shown="True" w1418 {
                  tunnel: [w1426 w1432] -> w1422
                  tunnel: w1413 -> [w1424 w1430]
                  frame False {
                    n481 = for {
                      tunnel: string[] ["Z STEPPER CAM HEIGHT", "READ STEPPER VALUES"] ("element") -> [w1427] mode=indexing
                      shift-right: [w1429] -> w1426
                      shift-left: w1424 -> [w1428]
                      n482 = Enqueue Element(queue=w1428, element=w1427) -> (queue out=w1429:refnum<queue>)  [unwired: 2 in, 2 out]
                    }
                  }
                  frame True {
                    n483 = for {
                      shift-right: [w1434] -> w1432
                      shift-left: w1430 -> [w1435]
                      tunnel: string[] ["ARDUINO - ULTRASONIC", "READ ULTRASONIC", ""] -> [w1433] mode=indexing
                      n484 = Enqueue Element(queue=w1435, element=w1433) -> (queue out=w1434:refnum<queue>)  [unwired: 2 in, 2 out]
                    }
                  }
                }
                n485 = Or(x=w1418, y=w1417) -> (x .or. y?=w1420:bool)
                n486 = Select(t=State_Type_Definitions,_for_0.26g_versions_and_later_2."True Stop" ("Enum"), s=w1417, f=State_Type_Definitions,_for_0.26g_versions_and_later_2."Task 8B: MOVE TO BOX" ("Enum")) -> (s? t:f=w1414:T6)
                n487 = Select(t=w1414, s=w1420, f=State_Type_Definitions,_for_0.26g_versions_and_later_2."Task 8A: RAISE ARM" ("Enum")) -> (s? t:f=w1419:T6)
              }
              frame "Exit" {
                n488 = for {
                  shift-right: [w1442] -> w1439
                  shift-left: w1436 -> [w1443]
                  tunnel: string[] ["STOP", "RESET ENCODERS", "RESET YAW", "ARDUINO MODE 0"] -> [w1441] mode=indexing
                  n489 = Enqueue Element(queue=w1443, element=w1441) -> (queue out=w1442:refnum<queue>)  [unwired: 2 in, 2 out]
                }
              }
            }
          }
          frame 28 {
            w1450 = u8 20 ("y")
            # ">>> yStepper command>>>"
            n490 = Less?(x=w1447, y=w1450) -> (x < y?=w1448:bool)
            n491 = Dequeue Element(queue=w1454, timeout in ms (-1)=w1453, error in (no error)=w1455) -> (element=w1452:T7)  [unwired: 3 out]
            n492 = Less?(x=w1446, y=w1450) -> (x < y?=w1449:bool)
            n493 = And(x=w1449, y=w1448) -> (x .and. y?=w1445:bool)
            n494 = case shown="\"None\", Default" w1452 {
              tunnel: [w1467 State_Type_Definitions,_for_0.26g_versions_and_later_2."True Stop" ("Enum")] -> w1457
              tunnel: [w1470 w1487] -> w1456
              tunnel: [State_Type_Definitions,_for_0.26g_versions_and_later_2."Idle" ("Enum") State_Type_Definitions,_for_0.26g_versions_and_later_2."Shutdown" ("Enum")] -> w1458
              tunnel: w1460 -> [w1466 _]
              tunnel: w1459 -> [w1462 w1484]
              tunnel: w1445 -> [w1461 _]
              frame "None", Default {
                # "Stays in Task 5_B to capture image over 5 seconds"
                # "T: Go back to idle, F: Continue with task\""
                # ">> Manual override >>"
                n495 = case shown="False" w1461 {
                  tunnel: [w1474 w1480] -> w1470
                  tunnel: w1462 -> [w1472 w1478]
                  frame False {
                    n496 = for {
                      tunnel: string[] ["FORWARD", "READ ULTRASONIC", "READ NAVX"] ("element") -> [w1475] mode=indexing
                      shift-right: [w1477] -> w1474
                      shift-left: w1472 -> [w1476]
                      n497 = Enqueue Element(queue=w1476, element=w1475) -> (queue out=w1477:refnum<queue>)  [unwired: 2 in, 2 out]
                    }
                  }
                  frame True {
                    n498 = for {
                      shift-right: [w1482] -> w1480
                      shift-left: w1478 -> [w1483]
                      tunnel: string[] ["STOP", "RESET ENCODERS", "OPEN LOG CAM", "SET TIMER 2"] -> [w1481] mode=indexing
                      n499 = Enqueue Element(queue=w1483, element=w1481) -> (queue out=w1482:refnum<queue>)  [unwired: 2 in, 2 out]
                    }
                  }
                }
                n500 = Or(x=w1461, y=w1466) -> (x .or. y?=w1468:bool)
                n501 = Select(t=State_Type_Definitions,_for_0.26g_versions_and_later_2."True Stop" ("Enum"), s=w1466, f=State_Type_Definitions,_for_0.26g_versions_and_later_2."Task 8C: CAM BURST" ("Enum")) -> (s? t:f=w1463:T6)
                n502 = Select(t=w1463, s=w1468, f=State_Type_Definitions,_for_0.26g_versions_and_later_2."Task 8B: MOVE TO BOX" ("Enum")) -> (s? t:f=w1467:T6)
              }
              frame "Exit" {
                n503 = for {
                  shift-right: [w1490] -> w1487
                  shift-left: w1484 -> [w1491]
                  tunnel: string[] ["STOP", "RESET ENCODERS", "RESET YAW", "ARDUINO MODE 0"] -> [w1489] mode=indexing
                  n504 = Enqueue Element(queue=w1491, element=w1489) -> (queue out=w1490:refnum<queue>)  [unwired: 2 in, 2 out]
                }
              }
            }
          }
          frame 29 {
            # ">>> Motor control cluster >>>"
            # ">>> yStepper command>>>"
            # ">> Manual override >>"
            n505 = Dequeue Element(queue=w1501, timeout in ms (-1)=w1500, error in (no error)=w1499) -> (element=w1498:T7)  [unwired: 3 out]
            n506 = case shown="\"None\", Default" w1498 {
              tunnel: [w1510 State_Type_Definitions,_for_0.26g_versions_and_later_2."True Stop" ("Enum")] -> w1503
              tunnel: [w1513 w1530] -> w1496
              tunnel: [State_Type_Definitions,_for_0.26g_versions_and_later_2."Idle" ("Enum") State_Type_Definitions,_for_0.26g_versions_and_later_2."Shutdown" ("Enum")] -> w1495
              tunnel: w1497 -> [w1504 _]
              tunnel: w1502 -> [w1509 w1527]
              tunnel: w1493 -> [w1508 _]
              frame "None", Default {
                # ">> Is time up? >>"
                # "Determines if object is in range to pick up"
                # ">> Manual override >>"
                n507 = case shown="True" w1508 {
                  tunnel: [w1517 w1523] -> w1513
                  tunnel: w1509 -> [w1515 w1521]
                  frame False {
                    n508 = for {
                      tunnel: string[] ["CAM ACQ", "START TIMER"] ("element") -> [w1518] mode=indexing
                      shift-right: [w1520] -> w1517
                      shift-left: w1515 -> [w1519]
                      n509 = Enqueue Element(queue=w1519, element=w1518) -> (queue out=w1520:refnum<queue>)  [unwired: 2 in, 2 out]
                    }
                  }
                  frame True {
                    n510 = for {
                      shift-right: [w1525] -> w1523
                      shift-left: w1521 -> [w1526]
                      tunnel: string[] ["CAM CLOSE", "PROCESS IMAGE", "SET TIMER 5"] -> [w1524] mode=indexing
                      n511 = Enqueue Element(queue=w1526, element=w1524) -> (queue out=w1525:refnum<queue>)  [unwired: 2 in, 2 out]
                    }
                  }
                }
                n512 = Or(x=w1508, y=w1504) -> (x .or. y?=w1511:bool)
                n513 = Select(t=State_Type_Definitions,_for_0.26g_versions_and_later_2."True Stop" ("Enum"), s=w1504, f=State_Type_Definitions,_for_0.26g_versions_and_later_2."Task 8D: PROCESS IMAGE" ("Enum")) -> (s? t:f=w1506:T6)
                n514 = Select(t=w1506, s=w1511, f=State_Type_Definitions,_for_0.26g_versions_and_later_2."Task 8C: CAM BURST" ("Enum")) -> (s? t:f=w1510:T6)
              }
              frame "Exit" {
                n515 = for {
                  shift-right: [w1533] -> w1530
                  shift-left: w1527 -> [w1534]
                  tunnel: string[] ["STOP", "RESET ENCODERS", "RESET YAW", "ARDUINO MODE 0"] -> [w1532] mode=indexing
                  n516 = Enqueue Element(queue=w1534, element=w1532) -> (queue out=w1533:refnum<queue>)  [unwired: 2 in, 2 out]
                }
              }
            }
          }
          frame 30 {
            # ">>> yStepper command>>>"
            n517 = Dequeue Element(queue=w1541, timeout in ms (-1)=w1540, error in (no error)=w1539) -> (element=w1538:T7)  [unwired: 3 out]
            n518 = case shown="\"None\", Default" w1538 {
              tunnel: [w1553 State_Type_Definitions,_for_0.26g_versions_and_later_2."True Stop" ("Enum")] -> w1545
              tunnel: [w1556 w1573] -> w1544
              tunnel: [State_Type_Definitions,_for_0.26g_versions_and_later_2."Idle" ("Enum") State_Type_Definitions,_for_0.26g_versions_and_later_2."Shutdown" ("Enum")] -> w1546
              tunnel: w1542 -> [w1552 _]
              tunnel: w1543 -> [w1548 w1570]
              tunnel: w1536 -> [w1547 _]
              frame "None", Default {
                # ">> T: Breaks out of state loop; F: Stays in loop>>"
                # ">> Manual override >>"
                # ">> Checks if time is up>>"
                # "Stays in Task 5D until the object is detected"
                # "T: Go back to idle, F: Continue with task\""
                # ">> Manual override >>"
                n519 = case shown="True" w1547 {
                  tunnel: [w1560 w1566] -> w1556
                  tunnel: w1548 -> [w1558 w1564]
                  frame False {
                    n520 = for {
                      tunnel: string[] ["START TIMER", "PROCESS IMAGE", ""] ("element") -> [w1561] mode=indexing
                      shift-right: [w1563] -> w1560
                      shift-left: w1558 -> [w1562]
                      n521 = Enqueue Element(queue=w1562, element=w1561) -> (queue out=w1563:refnum<queue>)  [unwired: 2 in, 2 out]
                    }
                  }
                  frame True {
                    n522 = for {
                      shift-right: [w1568] -> w1566
                      shift-left: w1564 -> [w1569]
                      tunnel: string[] ["CAM CLOSE", "RESET ENCODERS", ""] -> [w1567] mode=indexing
                      n523 = Enqueue Element(queue=w1569, element=w1567) -> (queue out=w1568:refnum<queue>)  [unwired: 2 in, 2 out]
                    }
                  }
                }
                n524 = Or(x=w1547, y=w1552) -> (x .or. y?=w1554:bool)
                n525 = Select(t=State_Type_Definitions,_for_0.26g_versions_and_later_2."True Stop" ("Enum"), s=w1552, f=State_Type_Definitions,_for_0.26g_versions_and_later_2."Task 8E: ROBOT ADJUST" ("Enum")) -> (s? t:f=w1549:T6)
                n526 = Select(t=w1549, s=w1554, f=State_Type_Definitions,_for_0.26g_versions_and_later_2."Task 8D: PROCESS IMAGE" ("Enum")) -> (s? t:f=w1553:T6)
              }
              frame "Exit" {
                n527 = for {
                  shift-right: [w1576] -> w1573
                  shift-left: w1570 -> [w1577]
                  tunnel: string[] ["STOP", "RESET ENCODERS", "RESET YAW", "ARDUINO MODE 0"] -> [w1575] mode=indexing
                  n528 = Enqueue Element(queue=w1577, element=w1575) -> (queue out=w1576:refnum<queue>)  [unwired: 2 in, 2 out]
                }
              }
            }
          }
          frame 31 {
            # ">>> Motor control cluster >>>"
            # ">>> yStepper command>>>"
            n529 = Dequeue Element(queue=w1594, timeout in ms (-1)=w1593, error in (no error)=w1592) -> (element=w1591:T7)  [unwired: 3 out]
            n530 = Subtract(x=w1589, y=300.0) -> (x-y=w1587:dbl)
            "x-y" <- w1587
            n531 = formula code="if (error < -80 && error >-300){\ndistance = -20;\nxSpeed = -30;\n}\n\nelse if (error <= 61&&error >= -80){\ndistance = -15;\nxSpeed = -30;\n}\n\nelse if (error <= -51 && error >= -60){\ndistance = -10;\nxSpeed = -30;\n}\n\nelse if (error >= -50 && error <= 50){\ndistance = 0;\nxSpeed = 0;\n}\n\nelse if (error >= 51 && error <= 80){\ndistance = 10;\nxSpeed = 30;\n}\n\nelse if (error >= 81 && error <= 100){\ndistance = 15;\nxSpeed = 30;\n}\n\nelse if (error >= 101 && error <= 120){\ndistance = 20;\nxSpeed = 30;\n}\n\nelse if (error >= 121){\ndistance = 25;\nxSpeed = 30;\n}\n\nelse{\ndistance = 0;\nxSpeed = 0;\n}"("error"=w1587) -> ("distance"=w1581:dbl, "xSpeed"=w1584:dbl)
            n532 = Greater Or Equal?(x=w1580, y=w1581) -> (x >= y?=w1582:bool)
            n533 = Greater Than 0?(x=w1581) -> (x > 0?=w1583:bool)
            n534 = Less Or Equal?(x=w1580, y=w1581) -> (x <= y?=w1579:bool)
            n535 = Select(t=w1582, s=w1583, f=w1579) -> (s? t:f=w1578:bool)
            n536 = case shown="\"None\", Default" w1591 {
              tunnel: [w1606 State_Type_Definitions,_for_0.26g_versions_and_later_2."True Stop" ("Enum")] -> w1598
              tunnel: [w1609 w1626] -> w1597
              tunnel: [State_Type_Definitions,_for_0.26g_versions_and_later_2."Idle" ("Enum") State_Type_Definitions,_for_0.26g_versions_and_later_2."Shutdown" ("Enum")] -> w1599
              tunnel: w1595 -> [w1605 _]
              tunnel: w1596 -> [w1601 w1623]
              tunnel: w1578 -> [w1600 _]
              frame "None", Default {
                # ">> T: Breaks out of state loop; F: Stays in loop>>"
                # ">> Manual override >>"
                # ">> Checks if time is up>>"
                # "Stays in Task 5D until the object is detected"
                # "T: Go back to idle, F: Continue with task\""
                # ">> Manual override >>"
                n537 = case shown="True" w1600 {
                  tunnel: [w1613 w1619] -> w1609
                  tunnel: w1601 -> [w1611 w1617]
                  frame False {
                    n538 = for {
                      tunnel: string[] ["X AXIS - SLOW", "READ ENCODERS", "READ YAW"] ("element") -> [w1614] mode=indexing
                      shift-right: [w1616] -> w1613
                      shift-left: w1611 -> [w1615]
                      n539 = Enqueue Element(queue=w1615, element=w1614) -> (queue out=w1616:refnum<queue>)  [unwired: 2 in, 2 out]
                    }
                  }
                  frame True {
                    n540 = for {
                      shift-right: [w1621] -> w1619
                      shift-left: w1617 -> [w1622]
                      tunnel: string[] ["OPEN LOG CAM", "DISPOSE BUFFERS", "SET TIMER 2", "STOP"] -> [w1620] mode=indexing
                      n541 = Enqueue Element(queue=w1622, element=w1620) -> (queue out=w1621:refnum<queue>)  [unwired: 2 in, 2 out]
                    }
                  }
                }
                n542 = Or(x=w1600, y=w1605) -> (x .or. y?=w1607:bool)
                n543 = Select(t=State_Type_Definitions,_for_0.26g_versions_and_later_2."True Stop" ("Enum"), s=w1605, f=State_Type_Definitions,_for_0.26g_versions_and_later_2."Task 8F: CAM BURST 2" ("Enum")) -> (s? t:f=w1602:T6)
                n544 = Select(t=w1602, s=w1607, f=State_Type_Definitions,_for_0.26g_versions_and_later_2."Task 8E: ROBOT ADJUST" ("Enum")) -> (s? t:f=w1606:T6)
              }
              frame "Exit" {
                n545 = for {
                  shift-right: [w1629] -> w1626
                  shift-left: w1623 -> [w1630]
                  tunnel: string[] ["STOP", "RESET ENCODERS", "RESET YAW", "ARDUINO MODE 0"] -> [w1628] mode=indexing
                  n546 = Enqueue Element(queue=w1630, element=w1628) -> (queue out=w1629:refnum<queue>)  [unwired: 2 in, 2 out]
                }
              }
            }
            n547 = Bundle By Name(cluster=w1586, "xSpeed"=w1584) -> (w1585:T8)
          }
          frame 32 {
            # ">>> Motor control cluster >>>"
            # ">>> yStepper command>>>"
            # ">> Manual override >>"
            n548 = Dequeue Element(queue=w1640, timeout in ms (-1)=w1639, error in (no error)=w1638) -> (element=w1637:T7)  [unwired: 3 out]
            n549 = case shown="\"None\", Default" w1637 {
              tunnel: [w1649 State_Type_Definitions,_for_0.26g_versions_and_later_2."True Stop" ("Enum")] -> w1642
              tunnel: [w1652 w1669] -> w1635
              tunnel: [State_Type_Definitions,_for_0.26g_versions_and_later_2."Idle" ("Enum") State_Type_Definitions,_for_0.26g_versions_and_later_2."Shutdown" ("Enum")] -> w1634
              tunnel: w1636 -> [w1643 _]
              tunnel: w1641 -> [w1648 w1666]
              tunnel: w1632 -> [w1647 _]
              frame "None", Default {
                # ">> Is time up? >>"
                # "Determines if object is in range to pick up"
                # ">> Manual override >>"
                n550 = case shown="True" w1647 {
                  tunnel: [w1656 w1662] -> w1652
                  tunnel: w1648 -> [w1654 w1660]
                  frame False {
                    n551 = for {
                      tunnel: string[] ["CAM ACQ", "START TIMER"] ("element") -> [w1657] mode=indexing
                      shift-right: [w1659] -> w1656
                      shift-left: w1654 -> [w1658]
                      n552 = Enqueue Element(queue=w1658, element=w1657) -> (queue out=w1659:refnum<queue>)  [unwired: 2 in, 2 out]
                    }
                  }
                  frame True {
                    n553 = for {
                      shift-right: [w1664] -> w1662
                      shift-left: w1660 -> [w1665]
                      tunnel: string[] ["CAM CLOSE", "PROCESS IMAGE", "SET TIMER 5"] -> [w1663] mode=indexing
                      n554 = Enqueue Element(queue=w1665, element=w1663) -> (queue out=w1664:refnum<queue>)  [unwired: 2 in, 2 out]
                    }
                  }
                }
                n555 = Or(x=w1647, y=w1643) -> (x .or. y?=w1650:bool)
                n556 = Select(t=State_Type_Definitions,_for_0.26g_versions_and_later_2."True Stop" ("Enum"), s=w1643, f=State_Type_Definitions,_for_0.26g_versions_and_later_2."Task 8G: PROCESS IMAGE 2" ("Enum")) -> (s? t:f=w1645:T6)
                n557 = Select(t=w1645, s=w1650, f=State_Type_Definitions,_for_0.26g_versions_and_later_2."Task 8F: CAM BURST 2" ("Enum")) -> (s? t:f=w1649:T6)
              }
              frame "Exit" {
                n558 = for {
                  shift-right: [w1672] -> w1669
                  shift-left: w1666 -> [w1673]
                  tunnel: string[] ["STOP", "RESET ENCODERS", "RESET YAW", "ARDUINO MODE 0"] -> [w1671] mode=indexing
                  n559 = Enqueue Element(queue=w1673, element=w1671) -> (queue out=w1672:refnum<queue>)  [unwired: 2 in, 2 out]
                }
              }
            }
          }
          frame 33 {
            # ">>> yStepper command>>>"
            n560 = Dequeue Element(queue=w1680, timeout in ms (-1)=w1679, error in (no error)=w1678) -> (element=w1677:T7)  [unwired: 3 out]
            n561 = case shown="\"None\", Default" w1677 {
              tunnel: [w1692 State_Type_Definitions,_for_0.26g_versions_and_later_2."True Stop" ("Enum")] -> w1684
              tunnel: [w1695 w1712] -> w1683
              tunnel: [State_Type_Definitions,_for_0.26g_versions_and_later_2."Idle" ("Enum") State_Type_Definitions,_for_0.26g_versions_and_later_2."Shutdown" ("Enum")] -> w1685
              tunnel: w1681 -> [w1691 _]
              tunnel: w1682 -> [w1687 w1709]
              tunnel: w1675 -> [w1686 _]
              frame "None", Default {
                # ">> T: Breaks out of state loop; F: Stays in loop>>"
                # ">> Manual override >>"
                # ">> Checks if time is up>>"
                # "Stays in Task 5D until the object is detected"
                # "T: Go back to idle, F: Continue with task\""
                # ">> Manual override >>"
                n562 = case shown="False" w1686 {
                  tunnel: [w1699 w1705] -> w1695
                  tunnel: w1687 -> [w1697 w1703]
                  frame False {
                    n563 = for {
                      tunnel: string[] ["START TIMER", "PROCESS IMAGE", "CAM CLOSE"] ("element") -> [w1700] mode=indexing
                      shift-right: [w1702] -> w1699
                      shift-left: w1697 -> [w1701]
                      n564 = Enqueue Element(queue=w1701, element=w1700) -> (queue out=w1702:refnum<queue>)  [unwired: 2 in, 2 out]
                    }
                  }
                  frame True {
                    n565 = for {
                      shift-right: [w1707] -> w1705
                      shift-left: w1703 -> [w1708]
                      tunnel: string[] ["CAM CLOSE", "", ""] -> [w1706] mode=indexing
                      n566 = Enqueue Element(queue=w1708, element=w1706) -> (queue out=w1707:refnum<queue>)  [unwired: 2 in, 2 out]
                    }
                  }
                }
                n567 = Or(x=w1686, y=w1691) -> (x .or. y?=w1693:bool)
                n568 = Select(t=State_Type_Definitions,_for_0.26g_versions_and_later_2."True Stop" ("Enum"), s=w1691, f=State_Type_Definitions,_for_0.26g_versions_and_later_2."Task 8H: ARM ADJUST" ("Enum")) -> (s? t:f=w1688:T6)
                n569 = Select(t=w1688, s=w1693, f=State_Type_Definitions,_for_0.26g_versions_and_later_2."Task 8G: PROCESS IMAGE 2" ("Enum")) -> (s? t:f=w1692:T6)
              }
              frame "Exit" {
                n570 = for {
                  shift-right: [w1715] -> w1712
                  shift-left: w1709 -> [w1716]
                  tunnel: string[] ["STOP", "RESET ENCODERS", "RESET YAW", "ARDUINO MODE 0"] -> [w1714] mode=indexing
                  n571 = Enqueue Element(queue=w1716, element=w1714) -> (queue out=w1715:refnum<queue>)  [unwired: 2 in, 2 out]
                }
              }
            }
          }
          frame 34 {
            # ">>> yStepper command>>>"
            n572 = Dequeue Element(queue=w1729, timeout in ms (-1)=w1730, error in (no error)=w1731) -> (element=w1733:T7)  [unwired: 3 out]
            n573 = formula code="if (pos < 100)\ny = 35;\n\nelse if (pos >= 100 && pos <= 140)\ny = 30;\n\nelse if (pos >= 141 && pos <= 170)\ny = 25;\n\nelse if (pos >= 171 &&pos <= 180) \ny = 20;\n\nelse if (pos >= 181&& pos <= 200)\ny = 15;\n\nelse if (pos >= 201 && pos <= 230)\ny = 10;\n\nelse if (pos >= 231 && pos <= 320)\ny = 8;\n\nelse if (pos > 320)\ny = 0;"("pos"=w1721) -> ("y"=w1724:dbl)
            n574 = To Unsigned Byte Integer(number=w1724) -> (unsigned 8bit integer=w1719:u8)
            n575 = Equal?(x=w1720, y=w1719) -> (x = y?=w1718:bool)
            n576 = case shown="\"None\", Default" w1733 {
              tunnel: [w1740 State_Type_Definitions,_for_0.26g_versions_and_later_2."True Stop" ("Enum")] -> w1727
              tunnel: [w1743 w1760] -> w1725
              tunnel: [State_Type_Definitions,_for_0.26g_versions_and_later_2."Idle" ("Enum") State_Type_Definitions,_for_0.26g_versions_and_later_2."Shutdown" ("Enum")] -> w1726
              tunnel: w1732 -> [w1739 _]
              tunnel: w1728 -> [w1735 w1757]
              tunnel: w1718 -> [w1734 _]
              frame "None", Default {
                # ">> T: Breaks out of state loop; F: Stays in loop>>"
                # ">> Manual override >>"
                # ">> Checks if time is up>>"
                # "Stays in Task 5D until the object is detected"
                # "T: Go back to idle, F: Continue with task\""
                # ">> Manual override >>"
                n577 = case shown="True" w1734 {
                  tunnel: [w1747 w1753] -> w1743
                  tunnel: w1735 -> [w1745 w1751]
                  frame False {
                    n578 = for {
                      tunnel: string[] ["READ STEPPER VALUES", "Y STEPPER CONTROL", ""] ("element") -> [w1748] mode=indexing
                      shift-right: [w1750] -> w1747
                      shift-left: w1745 -> [w1749]
                      n579 = Enqueue Element(queue=w1749, element=w1748) -> (queue out=w1750:refnum<queue>)  [unwired: 2 in, 2 out]
                    }
                  }
                  frame True {
                    n580 = for {
                      shift-right: [w1755] -> w1753
                      shift-left: w1751 -> [w1756]
                      tunnel: string[] ["CAM CLOSE", "DISPOSE BUFFERS", ""] -> [w1754] mode=indexing
                      n581 = Enqueue Element(queue=w1756, element=w1754) -> (queue out=w1755:refnum<queue>)  [unwired: 2 in, 2 out]
                    }
                  }
                }
                n582 = Or(x=w1734, y=w1739) -> (x .or. y?=w1741:bool)
                n583 = Select(t=State_Type_Definitions,_for_0.26g_versions_and_later_2."True Stop" ("Enum"), s=w1739, f=State_Type_Definitions,_for_0.26g_versions_and_later_2."Task 8I: ARM GRAB HEIGHT" ("Enum")) -> (s? t:f=w1736:T6)
                n584 = Select(t=w1736, s=w1741, f=State_Type_Definitions,_for_0.26g_versions_and_later_2."Task 8H: ARM ADJUST" ("Enum")) -> (s? t:f=w1740:T6)
              }
              frame "Exit" {
                n585 = for {
                  shift-right: [w1763] -> w1760
                  shift-left: w1757 -> [w1764]
                  tunnel: string[] ["STOP", "RESET ENCODERS", "RESET YAW", "ARDUINO MODE 0"] -> [w1762] mode=indexing
                  n586 = Enqueue Element(queue=w1764, element=w1762) -> (queue out=w1763:refnum<queue>)  [unwired: 2 in, 2 out]
                }
              }
            }
            n587 = Bundle By Name(cluster=w1723, "yStepper desired"=w1719) -> (w1722:T10)
          }
          frame 35 {
            # ">>> Motor control cluster >>>"
            # ">>> yStepper command>>>"
            # ">> Manual override >>"
            n588 = Dequeue Element(queue=w1774, timeout in ms (-1)=w1773, error in (no error)=w1775) -> (element=w1772:T7)  [unwired: 3 out]
            n589 = Equal?(x=w1771, y=u8 1) -> (x = y?=w1769:bool)
            n590 = case shown="\"None\", Default" w1772 {
              tunnel: [w1785 State_Type_Definitions,_for_0.26g_versions_and_later_2."True Stop" ("Enum")] -> w1776
              tunnel: [w1788 w1805] -> w1777
              tunnel: [State_Type_Definitions,_for_0.26g_versions_and_later_2."Idle" ("Enum") State_Type_Definitions,_for_0.26g_versions_and_later_2."Shutdown" ("Enum")] -> w1778
              tunnel: w1769 -> [w1784 _]
              tunnel: w1768 -> [w1783 _]
              tunnel: w1767 -> [w1779 w1802]
              frame "None", Default {
                # "Stays in Task 5F until stepper reaches desired \nheight"
                # "T: Go back to idle, F: Continue with task\""
                # ">> Manual override >>"
                n591 = case shown="True" w1784 {
                  tunnel: [w1792 w1798] -> w1788
                  tunnel: w1779 -> [w1790 w1796]
                  frame False {
                    n592 = for {
                      tunnel: string[] ["Z STEPPER GRAB HEIGHT", "READ STEPPER VALUES"] ("element") -> [w1793] mode=indexing
                      shift-right: [w1795] -> w1792
                      shift-left: w1790 -> [w1794]
                      n593 = Enqueue Element(queue=w1794, element=w1793) -> (queue out=w1795:refnum<queue>)  [unwired: 2 in, 2 out]
                    }
                  }
                  frame True {
                    n594 = for {
                      shift-right: [w1800] -> w1798
                      shift-left: w1796 -> [w1801]
                      tunnel: string[] ["SET TIMER 5", "CLOSE CLAW", ""] -> [w1799] mode=indexing
                      n595 = Enqueue Element(queue=w1801, element=w1799) -> (queue out=w1800:refnum<queue>)  [unwired: 2 in, 2 out]
                    }
                  }
                }
                n596 = Or(x=w1784, y=w1783) -> (x .or. y?=w1786:bool)
                n597 = Select(t=State_Type_Definitions,_for_0.26g_versions_and_later_2."True Stop" ("Enum"), s=w1783, f=State_Type_Definitions,_for_0.26g_versions_and_later_2."Task 8J: CLOSE CLAW" ("Enum")) -> (s? t:f=w1780:T6)
                n598 = Select(t=w1780, s=w1786, f=State_Type_Definitions,_for_0.26g_versions_and_later_2."Task 8I: ARM GRAB HEIGHT" ("Enum")) -> (s? t:f=w1785:T6)
              }
              frame "Exit" {
                n599 = for {
                  shift-right: [w1808] -> w1805
                  shift-left: w1802 -> [w1809]
                  tunnel: string[] ["STOP", "RESET ENCODERS", "RESET YAW", "ARDUINO MODE 0"] -> [w1807] mode=indexing
                  n600 = Enqueue Element(queue=w1809, element=w1807) -> (queue out=w1808:refnum<queue>)  [unwired: 2 in, 2 out]
                }
              }
            }
          }
          frame 36 {
            # ">>> yStepper command>>>"
            # ">> Manual override >>"
            n601 = Dequeue Element(queue=w1819, timeout in ms (-1)=w1818, error in (no error)=w1817) -> (element=w1816:T7)  [unwired: 3 out]
            n602 = case shown="\"None\", Default" w1816 {
              tunnel: [w1828 State_Type_Definitions,_for_0.26g_versions_and_later_2."True Stop" ("Enum")] -> w1821
              tunnel: [w1831 w1848] -> w1814
              tunnel: [State_Type_Definitions,_for_0.26g_versions_and_later_2."Idle" ("Enum") State_Type_Definitions,_for_0.26g_versions_and_later_2."Shutdown" ("Enum")] -> w1813
              tunnel: w1815 -> [w1822 _]
              tunnel: w1820 -> [w1827 w1845]
              tunnel: w1811 -> [w1826 _]
              frame "None", Default {
                # ">> Is time up? >>"
                # "Determines if object is in range to pick up"
                # ">> Manual override >>"
                n603 = case shown="True" w1826 {
                  tunnel: [w1835 w1841] -> w1831
                  tunnel: w1827 -> [w1833 w1839]
                  frame False {
                    n604 = for {
                      tunnel: string[] ["CLOSE CLAW", "START TIMER"] ("element") -> [w1836] mode=indexing
                      shift-right: [w1838] -> w1835
                      shift-left: w1833 -> [w1837]
                      n605 = Enqueue Element(queue=w1837, element=w1836) -> (queue out=w1838:refnum<queue>)  [unwired: 2 in, 2 out]
                    }
                  }
                  frame True {
                    n606 = for {
                      shift-right: [w1843] -> w1841
                      shift-left: w1839 -> [w1844]
                      tunnel: string[] ["READ STEPPER VALUES", "", ""] -> [w1842] mode=indexing
                      n607 = Enqueue Element(queue=w1844, element=w1842) -> (queue out=w1843:refnum<queue>)  [unwired: 2 in, 2 out]
                    }
                  }
                }
                n608 = Or(x=w1826, y=w1822) -> (x .or. y?=w1829:bool)
                n609 = Select(t=State_Type_Definitions,_for_0.26g_versions_and_later_2."True Stop" ("Enum"), s=w1822, f=State_Type_Definitions,_for_0.26g_versions_and_later_2."Task 8K: RAISE MY SWORD" ("Enum")) -> (s? t:f=w1824:T6)
                n610 = Select(t=w1824, s=w1829, f=State_Type_Definitions,_for_0.26g_versions_and_later_2."Task 8J: CLOSE CLAW" ("Enum")) -> (s? t:f=w1828:T6)
              }
              frame "Exit" {
                n611 = for {
                  shift-right: [w1851] -> w1848
                  shift-left: w1845 -> [w1852]
                  tunnel: string[] ["STOP", "RESET ENCODERS", "RESET YAW", "ARDUINO MODE 0"] -> [w1850] mode=indexing
                  n612 = Enqueue Element(queue=w1852, element=w1850) -> (queue out=w1851:refnum<queue>)  [unwired: 2 in, 2 out]
                }
              }
            }
          }
          frame 37 {
            # ">>> yStepper command>>>"
            # ">> Manual override >>"
            n613 = Dequeue Element(queue=w1862, timeout in ms (-1)=w1861, error in (no error)=w1863) -> (element=w1860:T7)  [unwired: 3 out]
            n614 = Equal?(x=w1859, y=u8 60) -> (x = y?=w1857:bool)
            n615 = case shown="\"None\", Default" w1860 {
              tunnel: [w1873 State_Type_Definitions,_for_0.26g_versions_and_later_2."True Stop" ("Enum")] -> w1864
              tunnel: [w1876 w1893] -> w1865
              tunnel: [State_Type_Definitions,_for_0.26g_versions_and_later_2."Idle" ("Enum") State_Type_Definitions,_for_0.26g_versions_and_later_2."Shutdown" ("Enum")] -> w1866
              tunnel: w1857 -> [w1872 _]
              tunnel: w1856 -> [w1871 _]
              tunnel: w1855 -> [w1867 w1890]
              frame "None", Default {
                # "Stays in Task 5_A until stepper reaches desired \nheight"
                # "T: Go back to idle, F: Continue with task\""
                # ">> Manual override >>"
                n616 = case shown="False" w1872 {
                  tunnel: [w1880 w1886] -> w1876
                  tunnel: w1867 -> [w1878 w1884]
                  frame False {
                    n617 = for {
                      tunnel: string[] ["Z STEPPER CAM HEIGHT", "READ STEPPER VALUES"] ("element") -> [w1881] mode=indexing
                      shift-right: [w1883] -> w1880
                      shift-left: w1878 -> [w1882]
                      n618 = Enqueue Element(queue=w1882, element=w1881) -> (queue out=w1883:refnum<queue>)  [unwired: 2 in, 2 out]
                    }
                  }
                  frame True {
                    n619 = for {
                      shift-right: [w1888] -> w1886
                      shift-left: w1884 -> [w1889]
                      tunnel: string[] ["ARDUINO - ULTRASONIC", "READ ULTRASONIC", ""] -> [w1887] mode=indexing
                      n620 = Enqueue Element(queue=w1889, element=w1887) -> (queue out=w1888:refnum<queue>)  [unwired: 2 in, 2 out]
                    }
                  }
                }
                n621 = Or(x=w1872, y=w1871) -> (x .or. y?=w1874:bool)
                n622 = Select(t=State_Type_Definitions,_for_0.26g_versions_and_later_2."True Stop" ("Enum"), s=w1871, f=State_Type_Definitions,_for_0.26g_versions_and_later_2."True Stop" ("Enum")) -> (s? t:f=w1868:T6)
                n623 = Select(t=w1868, s=w1874, f=State_Type_Definitions,_for_0.26g_versions_and_later_2."Task 8K: RAISE MY SWORD" ("Enum")) -> (s? t:f=w1873:T6)
              }
              frame "Exit" {
                n624 = for {
                  shift-right: [w1896] -> w1893
                  shift-left: w1890 -> [w1897]
                  tunnel: string[] ["STOP", "RESET ENCODERS", "RESET YAW", "ARDUINO MODE 0"] -> [w1895] mode=indexing
                  n625 = Enqueue Element(queue=w1897, element=w1895) -> (queue out=w1896:refnum<queue>)  [unwired: 2 in, 2 out]
                }
              }
            }
          }
        }
      }
    }
    n626 = local write "Green LED"(w189) -> ()
  }
  n627 = while {
    tunnel: w48 -> [w2466]
    tunnel: w47 -> [w2463]
    stop <- w2460 stop-if-true
    # "Status Loop for Action Queues"
    n628 = Get Queue Status(queue=w2466, return elements? (F)=TRUE) -> (error out=w2462:errorcluster, # elements in queue=→"Action Queue Items":i32, elements=→"Action Queues items":string[])  [unwired: 1 in, 5 out]
    n629 = Get Queue Status(queue=w2463, return elements? (F)=TRUE) -> (# pending remove=→"State Logic Queue Items":i32, error out=w2461:errorcluster, elements=→"elements":T7[])  [unwired: 1 in, 5 out]
    n630 = Merge Errors(w2462, w2461) -> (w2460:errorcluster)
    n631 = Wait (ms)(milliseconds to wait=u32 500) -> ()  [unwired: 1 out]
  }
  n632 = call <vilib>:"DIO Close.vi"("error in (no error)"=w24, "DIO Info In"=w27) -> ()  [unwired: 9 in, 1 out]
  n633 = call <vilib>:"DIO Close.vi"("error in (no error)"=w34, "DIO Info In"=w36) -> ()  [unwired: 9 in, 1 out]
  n634 = call <vilib>:"NavX Close.vi"("error in (no error)"=w8, "NavX Info In"=w7) -> ()  [unwired: 9 in, 1 out]
  n635 = call <vilib>:"DIO Close.vi"("error in (no error)"=w29, "DIO Info In"=w31) -> ()  [unwired: 9 in, 1 out]
  n636 = call <vilib>:"DIO Close.vi"("error in (no error)"=w15, "DIO Info In"=w16) -> ()  [unwired: 9 in, 1 out]
  n637 = call <vilib>:"DIO Close.vi"("error in (no error)"=w10, "DIO Info In"=w11) -> ()  [unwired: 9 in, 1 out]
  n638 = while {
    stop <- w2470 stop-if-true
    n639 = call <vilib>:"RT Get CPU Loads.vi"() -> ("CPU loads"=→"CPU loads":T5[])  [unwired: 10 in, 1 out]
    n640 = Wait (ms)(milliseconds to wait=u32 100) -> ()  [unwired: 1 out]
    n641 = call "FGV Stop.vi"("Init/Read/Write State"=States_for_Action_Engine."Read") -> ("Output node"=w2470:bool)  [unwired: 2 in, 1 out]
  }
  n642 = while {
    stop <- w2474 stop-if-true
    n643 = call "MOTOR CONTROL WITH PID AE.vi"("AE Mode"=MOTOR_CONTROL_WITH_PID_AE_DATA_MODE_TYPE_DEF."Read from AE") -> ("Speed & distance"=→"Speed & distance":T1)  [unwired: 3 in]
    n644 = call "FGV Stop.vi"("Init/Read/Write State"=States_for_Action_Engine."Read") -> ("Output node"=w2474:bool)  [unwired: 2 in, 1 out]
    n645 = Wait (ms)(milliseconds to wait=u32 5) -> ()  [unwired: 1 out]
  }
  n646 = Merge Errors "Merge Errors"(w64, w63) -> (w46:errorcluster)
  n647 = Merge Errors(w50, w46) -> (w45:errorcluster)
  n648 = Destroy User Event(user event=w67, error in=w45) -> ()  [unwired: 1 out]
  n649 = Destroy User Event(user event=w68, error in=w45) -> ()  [unwired: 1 out]
  n650 = Unregister For Events(event registration refnum=w59, error in=w45) -> ()  [unwired: 1 out]
  n651 = Release Queue(queue=w41, error in (no error)=w45) -> (error out=→"error out":errorcluster)  [unwired: 1 in, 2 out]
  n652 = Release Queue(queue=w58, error in (no error)=w45) -> ()  [unwired: 1 in, 3 out]
